vi "main.vi"() -> ()   [LabVIEW 2014]
uses:
  UerDefineControl/quit.ctl
  UerDefineControl/MMMdsc.ctl
  UerDefineControl/chax.ctl
  UerDefineControl/timee.ctl
  UerDefineControl/power.ctl
  <vilib>/Math Plots/3D Math Plots/3D Surface/3D Surface XCtrl/3D Surface.xctl
  CYY/strr.ctl
  UerDefineControl/qiehuan.ctl
  controls/State.ctl
  Acquisition/User Specified Data.ctl
  Acquisition/HW Configuration.ctl
  Acquisition/AcqControls/Analysis Configuration.ctl
  Acquisition/AcqControls/New Data Behavior.ctl
  support/Message Queue/Enqueue Message (Single).vi
  <vilib>/imath/engines/lvmath2/RunTimeEngine/Managers/WorkSpace/UID Generator.vi
  <vilib>/imath/engines/lvmath2/RunTimeEngine/BuiltInFunctions/max/1 input/NIMS_max(RV).vi
  <instcachedir>/0/NIMS_max(RV)_237633DB1D604D5BA7001287DF3C7957.lvgen/NIMS_max(RV)_237633DB1D604D5BA7001287DF3C7957_000.vi
  <vilib>/imath/engines/lvmath2/RunTimeEngine/BuiltInFunctions/min/1 input/NIMS_min(RV).vi
  <instcachedir>/0/NIMS_min(RV)_EE2DD3E2888846108C5160A664B67832.lvgen/NIMS_min(RV)_EE2DD3E2888846108C5160A664B67832_000.vi
  <vilib>/imath/engines/lvmath2/RunTimeEngine/BuiltInFunctions/linramp/NIMS_linramp.vi
  <vilib>/imath/engines/lvmath2/RunTimeEngine/BuiltInFunctions/meshgrid2d/NIMS_meshgrid2d(V,V).vi
  <instcachedir>/0/NIMS_meshgrid2d(V,V)_3733343E1C554A708015CFB0432C6A59.lvgen/NIMS_meshgrid2d(V,V)_3733343E1C554A708015CFB0432C6A59_000.vi
  <vilib>/imath/engines/lvmath2/RunTimeEngine/BuiltInFunctions/intrp2d_uneven/NIMS_[1o]_intrp2d_uneven.vi
  <vilib>/imath/engines/lvmath2/RunTimeEngine/RunTimeType/NIMS_RunTimeType_From StrictType (excl LVString).vi
  <instcachedir>/0/NIMS_RunTimeType_From StrictType (excl LVString)_15A5391EEA9C4AACB9955AC755B83D29.lvgen/NIMS_RunTimeType_From StrictType (excl LVString)_15A5391EEA9C4AACB9955AC755B83D29_000.vi
  <vilib>/imath/engines/lvmath2/RunTimeEngine/ErrorHandling/NIMS_Error From Error Code.vi
  <vilib>/imath/engines/lvmath2/RunTimeEngine/LocalVariableDefStatement/MC_LocalVariableDefStatement_Display.vi
  <vilib>/imath/engines/lvmath2/RunTimeEngine/Managers/SymbolTable/Clear UID.vi
  <vilib>/imath/engines/lvmath2/RunTimeEngine/NodeEndStatement/NIMS_NodeEndStatement_Output.vi
  <instcachedir>/0/NIMS_NodeEndStatement_Output_53EC0D466D134D7ABD903AC30B43404B.lvgen/NIMS_NodeEndStatement_Output_53EC0D466D134D7ABD903AC30B43404B_002.vi
  <vilib>/imath/engines/lvmath2/RunTimeEngine/ErrorHandling/NIMS_Finalize Error.vi
  <vilib>/Math Plots/3D Math Plots/3D Surface/3D Surface Datatype/Public/Plot Helper (Matrix).vi
  <vilib>/Math Plots/3D Math Plots/3D Mesh/3D Mesh Datatype/Public/Plot Helper (Matrix).vi
  <vilib>/Math Plots/3D Math Plots/3D Contour/3D Contour Datatype/Public/Plot Helper (Matrix).vi
  <vilib>/imath/engines/lvmath2/RunTimeEngine/BuiltInFunctions/plot/NIMS_plot(RM, RM, Str).vi
  <vilib>/imathl/engines/lvmath/Functions/Error Handling/Create Error.vi
  Acquisition/Acquisitions.lvlib
  AreaSettingD/SettingD.llb/SettingD.lvlib
  DetectElecrodes/DetectElectros.lvlib
  PowerElectrode/PowerElectrodes.lvlib
  DSCBoard/Dsc_Board_Dlg.lvlib
  DscBoardDistributeElectrodes/DscBoardDistributeElectrodes.lvlib
  Sample/Sample.lvlib
  DataBase/DataBase.lvlib
  <vilib>/Math Plots/3D Math Plots/3D Surface/3D Surface Datatype/3D Surface Datatype.lvclass
  <vilib>/imath/engines/lvmath2/RunTimeEngine/Managers/SymbolTable/NIMS_WorkSpace.lvlib
  <vilib>/Math Plots/3D Math Plots/3D Contour/3D Contour Datatype/3D Contour Datatype.lvclass
  <vilib>/imath/engines/lvmath2/RunTimeEngine/BuiltInFunctions/mesh/NIMS_mesh(RM, RM).vi
  <vilib>/imath/engines/lvmath2/RunTimeEngine/BuiltInFunctions/grid/NIMS_grid(Enums).vi
  ChaxuConfig/ChaxuConfig.lvlib
  HardWare/HardWareConfig.lvlib
  <vilib>/Math Plots/3D Math Plots/3D Mesh/3D Mesh Datatype/3D Mesh Datatype.lvclass
  PowerControl/PowerControl.lvlib
  support/Message Queue/Message Queue.lvlib
  CYY/cyy.lvlib
  LeakageFenxi/LeakageFenXi.lvlib
panel:
  in  "界面切换":T1
  in  "电源控制":T2
  in  "定时检测":T3
  in  "SampleInfo":bool
  in  "电极配置信息查询":T4
  in  "Mdsc":T5
  in  "手动检测":T6
  in  "退出":T7
  out "采样过程中 ... 请不要进行其它操作":u32(slide) scale=0.0..400.0
  in  "采集板分配电极":bool
  in  "供电电极配置":bool
  in  "检测电极配置":bool
  in  "区域配置":bool
  in  "选项卡控件":enum32{"主界面", "数据监测界面", "测试数据", "测试数据 2"}(tab)
  out "Info 2":string
  out "3D Surface 3":refnum<class "3D Plot Datatype.lvclass">[](xcontrol) caption="三维曲面"
  out "Info":T8
  out "3D Surface":refnum<class "3D Plot Datatype.lvclass">[](xcontrol) caption="三维曲面"
  in  "数据监测界面":i32(listbox)
  out "定时采样信息D":string[][](array[string])
  out "定时检测事件":bool
  out "是否采样":bool
  in  "频率":dbl=1.0
  out "电流":string
  out "字符串":string="下层膜"
  out "选定检测区域":string
  out "数据采集模块地址":string
  out "elecNum":i32
  out "detec_electrode_name":string
  out "电压回来":string
  out "项标识符":string
  out "电压频率":string
  out "电压倍数":string
  out "Hz":i32
  out "实际输出电压":string
  out "电压系数":string
  out "输出电压值":string
  out "电压05V":string
  out "实际输出电压压":dbl
  out "电压系数输出":dbl
  out "回来电压":dbl
  out "NY":bool
  in  "设置按钮":bool
  # "Welcome to use Leakage Detection System !"
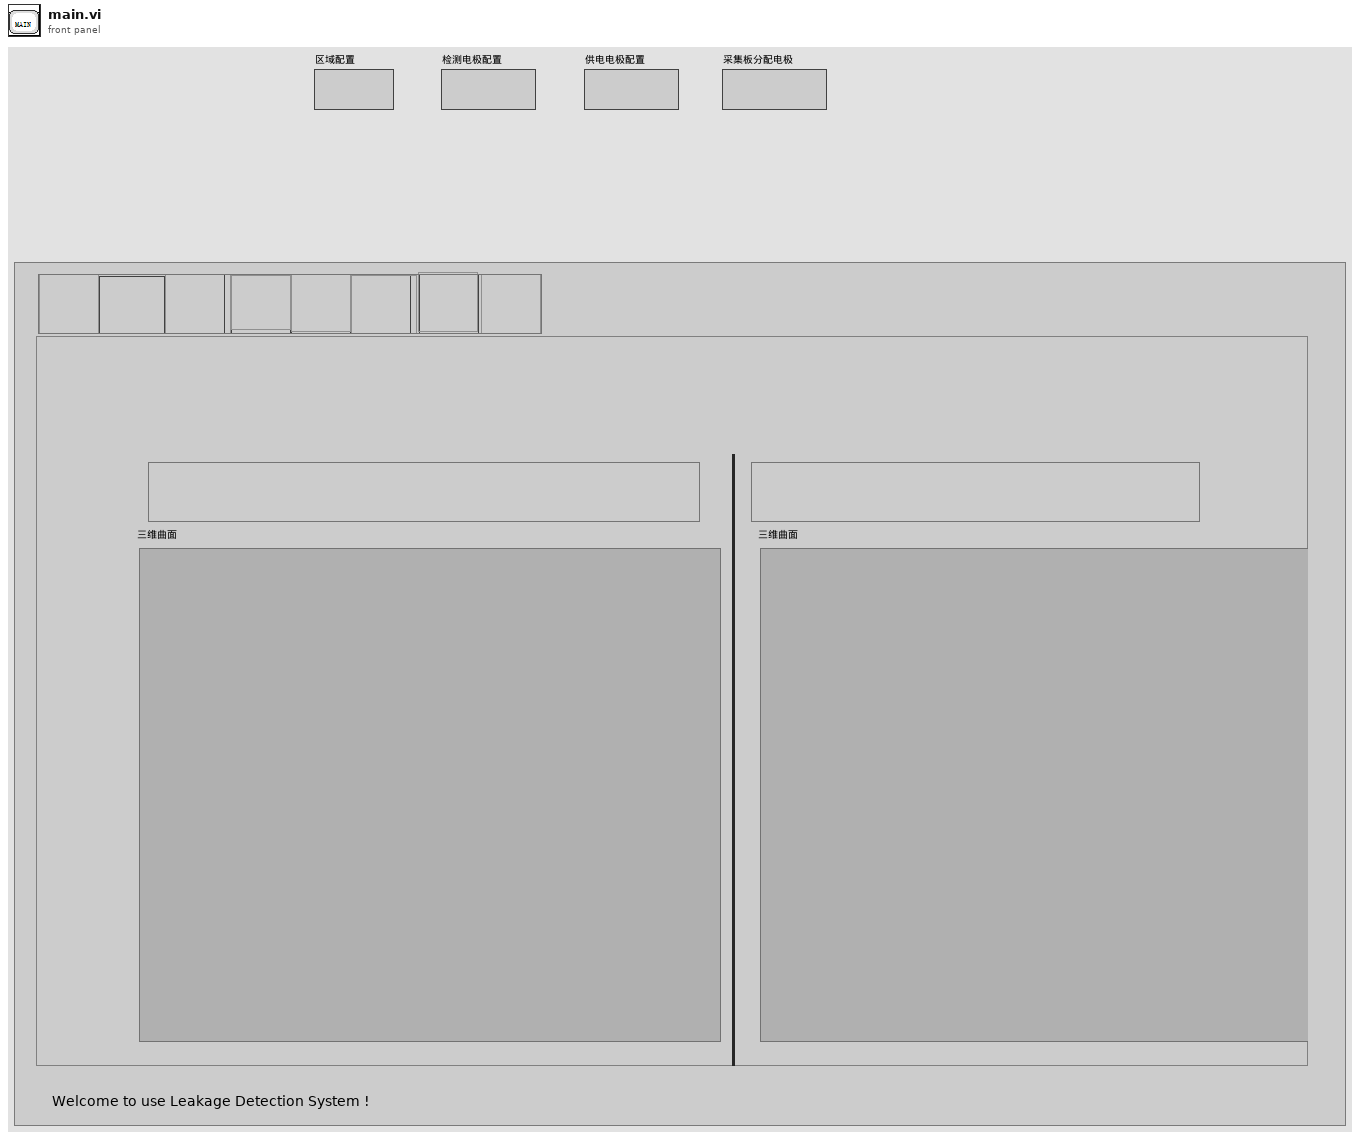
[diagram p1: front panel]
types:
  T1 = typedef "qiehuan.ctl" = bool
  T2 = typedef "power.ctl" = bool
  T3 = typedef "timee.ctl" = bool
  T4 = typedef "chax.ctl" = bool
  T5 = typedef "MMMdsc.ctl" = bool
  T6 = typedef "手动.ctl" = bool
  T7 = typedef "quit.ctl" = bool
  T8 = typedef "strr.ctl" = string
  T9 = cluster{"区域名称":string, "采样位置":string, "采样时间":string, "时":string, "分":string}
  T10 = typedef "State.ctl" = enum16{"Idle", "AOoutputting", "Timing", "SamplingAndSaving", "StartSample", "StopSample"}
  T11 = typedef "Message Queue.lvlib/All Message Queues.ctl" = cluster{"UI":refnum<queue>, "Acquisition":refnum<queue>, "Logging":refnum<queue>}
  T12 = cluster{"Max Input":dbl, "Min Input":dbl, "Sample Rate":dbl, "Sample Num":dbl, "DAQmx Task":refnum<k21>, "物理通道":tag}
  T13 = typedef "HardWareConfig.lvlib/Hardware Configures.ctl" = cluster{"Max Input":dbl, "Min Input":dbl, "Sample Rate":dbl, "Sample Num":dbl, "DAQmx Task":refnum<k21>, "物理通道":tag}
  T14 = enum32{"invalid app kind", "Development System", "Run Time System", "Student Edition", "Embedded LabVIEW", "Evaluation", "Custom"}
  T15 = enum32{"Invalid", "Standard", "Closed", "Hidden", "Minimized", "Maximized"}
  T16 = typedef "Acquisitions.lvlib/HW Configuration.ctl" = cluster{"Physical Channel":tag, "Maximum Input":dbl, "Minimum Input":dbl, "Sample Rate":dbl, "Number of Samples":i32}
  T17 = cluster{"Dev1ASData":cluster{"DevChSampData":cluster{"通道编号":string, "Data":dbl}[], "dscAddress":string}, "Dev2ASData":cluster{"DevChSampData":cluster{"通道编号":string, "Data":dbl}[], "dscAddress":string}, "Dev3ASData":cluster{"DevChSampData":cluster{"通道编号":string, "Data":dbl}[], "dscAddress":string}, "Dev4ASData":cluster{"DevChSampData":cluster{"通道编号":string, "Data":dbl}[], "dscAddress":string}, "Dev5ASData":cluster{"DevChSampData":cluster{"通道编号":string, "Data":dbl}[], "dscAddress":string}, "Dev6ASData":cluster{"DevChSampData":cluster{"通道编号":string, "Data":dbl}[], "dscAddress":string}, "Dev7ASData":cluster{"DevChSampData":cluster{"通道编号":string, "Data":dbl}[], "dscAddress":string}, "Dev8ASData":cluster{"DevChSampData":cluster{"通道编号":string, "Data":dbl}[], "dscAddress":string}, "Dev9ASData":cluster{"DevChSampData":cluster{"通道编号":string, "Data":dbl}[], "dscAddress":string}, "Dev10ASData":cluster{"DevChSampData":cluster{"通道编号":string, "Data":dbl}[], "dscAddress":string}, "Dev11ASData":cluster{"DevChSampData":cluster{"通道编号":string, "Data":dbl}[], "dscAddress":string}, "Dev12ASData":cluster{"DevChSampData":cluster{"通道编号":string, "Data":dbl}[], "dscAddress":string}, "Dev13ASData":cluster{"DevChSampData":cluster{"通道编号":string, "Data":dbl}[], "dscAddress":string}}
  T18 = typedef "Acquisitions.lvlib/User Specified Data.ctl" = cluster{"Hardware Configuration":T16, "Analysis Configuration":T19, "New Data Behavior":T20, "HWInfo":string}
  T19 = typedef "Acquisitions.lvlib/Analysis Configuration.ctl" = cluster{"Statistics":bool}
  T20 = typedef "Acquisitions.lvlib/New Data Behavior.ctl" = enum16{"Replace", "Overlay", "Append"}
  T21 = cluster{"Core":cluster{"Current VI Reference":refnum<vi>, "Close Panel on Exit?":bool}, "Your Boolean data":bool, "Your string data":string, "User Specified":T18, "手动采样信息":cluster{"选定检测区域":string, "采样位置":string, "电源电压":string, "电源电流":string, "电源频率":string, "检测方式":string, "备注":string}, "ManualSampleInfo":cluster{string, "date/time string":string, "选定检测区域":string, "采样位置":string, "检测方式":string, string, string, "电源电压":string, "电源电流":string, "备注":string}, "SampleData":dbl[], "AcquireData":waveform(dbl)[], "DevChSampleData":cluster{"数据采集模块地址":string, "0ChData":cluster{"通道编号":string, "Data":dbl}, "1ChData":cluster{"通道编号":string, "Data":dbl}, "2ChData":cluster{"通道编号":string, "Data":dbl}, "3ChData":cluster{"通道编号":string, "Data":dbl}, "4ChData":cluster{"通道编号":string, "Data":dbl}, "5ChData":cluster{"通道编号":string, "Data":dbl}, "6ChData":cluster{"通道编号":string, "Data":dbl}, "7ChData":cluster{"通道编号":string, "Data":dbl}, "8ChData":cluster{"通道编号":string, "Data":dbl}, "9ChData":cluster{"通道编号":string, "Data":dbl}, "10ChData":cluster{"通道编号":string, "Data":dbl}, "11ChData":cluster{"通道编号":string, "Data":dbl}, "12ChData":cluster{"通道编号":string, "Data":dbl}, "13ChData":cluster{"通道编号":string, "Data":dbl}, "14ChData":cluster{"通道编号":string, "Data":dbl}, "15ChData":cluster{"通道编号":string, "Data":dbl}, "16ChData":cluster{"通道编号":string, "Data":dbl}, "17ChData":cluster{"通道编号":string, "Data":dbl}, "18ChData":cluster{"通道编号":string, "Data":dbl}, "19ChData":cluster{"通道编号":string, "Data":dbl}, "20ChData":cluster{"通道编号":string, "Data":dbl}, "21ChData":cluster{"通道编号":string, "Data":dbl}, "22ChData":cluster{"通道编号":string, "Data":dbl}, "23ChData":cluster{"通道编号":string, "Data":dbl}, "24ChData":cluster{"通道编号":string, "Data":dbl}, "25ChData":cluster{"通道编号":string, "Data":dbl}, "26ChData":cluster{"通道编号":string, "Data":dbl}, "27ChData":cluster{"通道编号":string, "Data":dbl}, "28ChData":cluster{"通道编号":string, "Data":dbl}, "29ChData":cluster{"通道编号":string, "Data":dbl}, "30ChData":cluster{"通道编号":string, "Data":dbl}, "31ChData":cluster{"通道编号":string, "Data":dbl}}, "DevChSampData":cluster{"通道编号":string, "Data":dbl}[], "SampleInfoTime":string, "SampleData":string[][], "3DData":cluster{"X":dbl[], "Y":dbl[], "Z":dbl[]}, "定时采样信息":cluster{"检测区域":string, "检测频率":string, "时":u16, "分钟":u16, "供电位置":string, "是否启动":string, "备注":string}, "TimeSampleInfo":cluster{string, "采样时间":string, "检测区域":string, "供电位置":string, "采样方式":string, string, string, "电源电压":string, "电源电流":string, "备注":string}, "nCHData":cluster{"Dev1SampData":cluster{"通道编号":string, "Data":dbl}[], "Dev2SampData":cluster{"通道编号":string, "Data":dbl}[], "Dev3SampData":cluster{"通道编号":string, "Data":dbl}[], "Dev4SampData":cluster{"通道编号":string, "Data":dbl}[], "Dev5SampData":cluster{"通道编号":string, "Data":dbl}[], "Dev6SampData":cluster{"通道编号":string, "Data":dbl}[], "Dev7SampData":cluster{"通道编号":string, "Data":dbl}[], "Dev8SampData":cluster{"通道编号":string, "Data":dbl}[], "Dev9SampData":cluster{"通道编号":string, "Data":dbl}[], "Dev10SampData":cluster{"通道编号":string, "Data":dbl}[], "Dev11SampData":cluster{"通道编号":string, "Data":dbl}[], "Dev12SampData":cluster{"通道编号":string, "Data":dbl}[], "Dev13SampData":cluster{"通道编号":string, "Data":dbl}[]}, "DevNASSData":cluster{"Dev1ASData":cluster{"DevChSampData":cluster{"通道编号":string, "Data":dbl}[], "dscAddress":string}, "Dev2ASData":cluster{"DevChSampData":cluster{"通道编号":string, "Data":dbl}[], "dscAddress":string}, "Dev3ASData":cluster{"DevChSampData":cluster{"通道编号":string, "Data":dbl}[], "dscAddress":string}, "Dev4ASData":cluster{"DevChSampData":cluster{"通道编号":string, "Data":dbl}[], "dscAddress":string}, "Dev5ASData":cluster{"DevChSampData":cluster{"通道编号":string, "Data":dbl}[], "dscAddress":string}, "Dev6ASData":cluster{"DevChSampData":cluster{"通道编号":string, "Data":dbl}[], "dscAddress":string}, "Dev7ASData":cluster{"DevChSampData":cluster{"通道编号":string, "Data":dbl}[], "dscAddress":string}, "Dev8ASData":cluster{"DevChSampData":cluster{"通道编号":string, "Data":dbl}[], "dscAddress":string}, "Dev9ASData":cluster{"DevChSampData":cluster{"通道编号":string, "Data":dbl}[], "dscAddress":string}, "Dev10ASData":cluster{"DevChSampData":cluster{"通道编号":string, "Data":dbl}[], "dscAddress":string}, "Dev11ASData":cluster{"DevChSampData":cluster{"通道编号":string, "Data":dbl}[], "dscAddress":string}, "Dev12ASData":cluster{"DevChSampData":cluster{"通道编号":string, "Data":dbl}[], "dscAddress":string}, "Dev13ASData":cluster{"DevChSampData":cluster{"通道编号":string, "Data":dbl}[], "dscAddress":string}}, "PowTN":bool, "记录数":i32, "是否存在记录":bool, "power_f":string, "时分":string, "电压倍数":string, "回来电压":string, "回来电流":string, "Area_name":string, "电压系数":string, "基准电压":string, "手动采样到AO电压":string}
  T22 = typedef "LVPoint32TypeDef.ctl" = cluster{"Horizontal":i32, "Vertical":i32}
  T23 = typedef "LVRowAndColumnTypeDef.ctl" = cluster{"Row":i32, "Column":i32}
  T24 = cluster{string, "采样时间":string, "检测区域":string, "供电位置":string, "采样方式":string, string, string, "电源电压":string, "电源电流":string, "备注":string}
  T25 = cluster{"Dev1SampData":cluster{"通道编号":string, "Data":dbl}[], "Dev2SampData":cluster{"通道编号":string, "Data":dbl}[], "Dev3SampData":cluster{"通道编号":string, "Data":dbl}[], "Dev4SampData":cluster{"通道编号":string, "Data":dbl}[], "Dev5SampData":cluster{"通道编号":string, "Data":dbl}[], "Dev6SampData":cluster{"通道编号":string, "Data":dbl}[], "Dev7SampData":cluster{"通道编号":string, "Data":dbl}[], "Dev8SampData":cluster{"通道编号":string, "Data":dbl}[], "Dev9SampData":cluster{"通道编号":string, "Data":dbl}[], "Dev10SampData":cluster{"通道编号":string, "Data":dbl}[], "Dev11SampData":cluster{"通道编号":string, "Data":dbl}[], "Dev12SampData":cluster{"通道编号":string, "Data":dbl}[], "Dev13SampData":cluster{"通道编号":string, "Data":dbl}[]}
  T26 = cluster{"采样时间":string, string, "检测区域":string, "供电位置":string, "采样方式":string, "电源电压":string, string, "电源电流":string, string, "备注":string}
  T27 = cluster{"检测区域":string, "检测频率":string, "时":u16, "分钟":u16, "供电位置":string, "是否启动":string, "备注":string}
  T28 = cluster{"数据采集模块地址":string, "0ChData":cluster{"通道编号":string, "Data":dbl}, "1ChData":cluster{"通道编号":string, "Data":dbl}, "2ChData":cluster{"通道编号":string, "Data":dbl}, "3ChData":cluster{"通道编号":string, "Data":dbl}, "4ChData":cluster{"通道编号":string, "Data":dbl}, "5ChData":cluster{"通道编号":string, "Data":dbl}, "6ChData":cluster{"通道编号":string, "Data":dbl}, "7ChData":cluster{"通道编号":string, "Data":dbl}, "8ChData":cluster{"通道编号":string, "Data":dbl}, "9ChData":cluster{"通道编号":string, "Data":dbl}, "10ChData":cluster{"通道编号":string, "Data":dbl}, "11ChData":cluster{"通道编号":string, "Data":dbl}, "12ChData":cluster{"通道编号":string, "Data":dbl}, "13ChData":cluster{"通道编号":string, "Data":dbl}, "14ChData":cluster{"通道编号":string, "Data":dbl}, "15ChData":cluster{"通道编号":string, "Data":dbl}, "16ChData":cluster{"通道编号":string, "Data":dbl}, "17ChData":cluster{"通道编号":string, "Data":dbl}, "18ChData":cluster{"通道编号":string, "Data":dbl}, "19ChData":cluster{"通道编号":string, "Data":dbl}, "20ChData":cluster{"通道编号":string, "Data":dbl}, "21ChData":cluster{"通道编号":string, "Data":dbl}, "22ChData":cluster{"通道编号":string, "Data":dbl}, "23ChData":cluster{"通道编号":string, "Data":dbl}, "24ChData":cluster{"通道编号":string, "Data":dbl}, "25ChData":cluster{"通道编号":string, "Data":dbl}, "26ChData":cluster{"通道编号":string, "Data":dbl}, "27ChData":cluster{"通道编号":string, "Data":dbl}, "28ChData":cluster{"通道编号":string, "Data":dbl}, "29ChData":cluster{"通道编号":string, "Data":dbl}, "30ChData":cluster{"通道编号":string, "Data":dbl}, "31ChData":cluster{"通道编号":string, "Data":dbl}}
  T29 = cluster{string, "date/time string":string, "选定检测区域":string, "采样位置":string, "检测方式":string, string, string, "电源电压":string, "电源电流":string, "备注":string}
  T30 = cluster{"选定检测区域":string, "采样位置":string, "电源电压":string, "电源电流":string, "电源频率":string, "检测方式":string, "备注":string}
  T31 = cluster{"Current VI Reference":refnum<vi>, "Close Panel on Exit?":bool}
  T32 = cluster{"DevChSampData":cluster{"通道编号":string, "Data":dbl}[], "dscAddress":string}
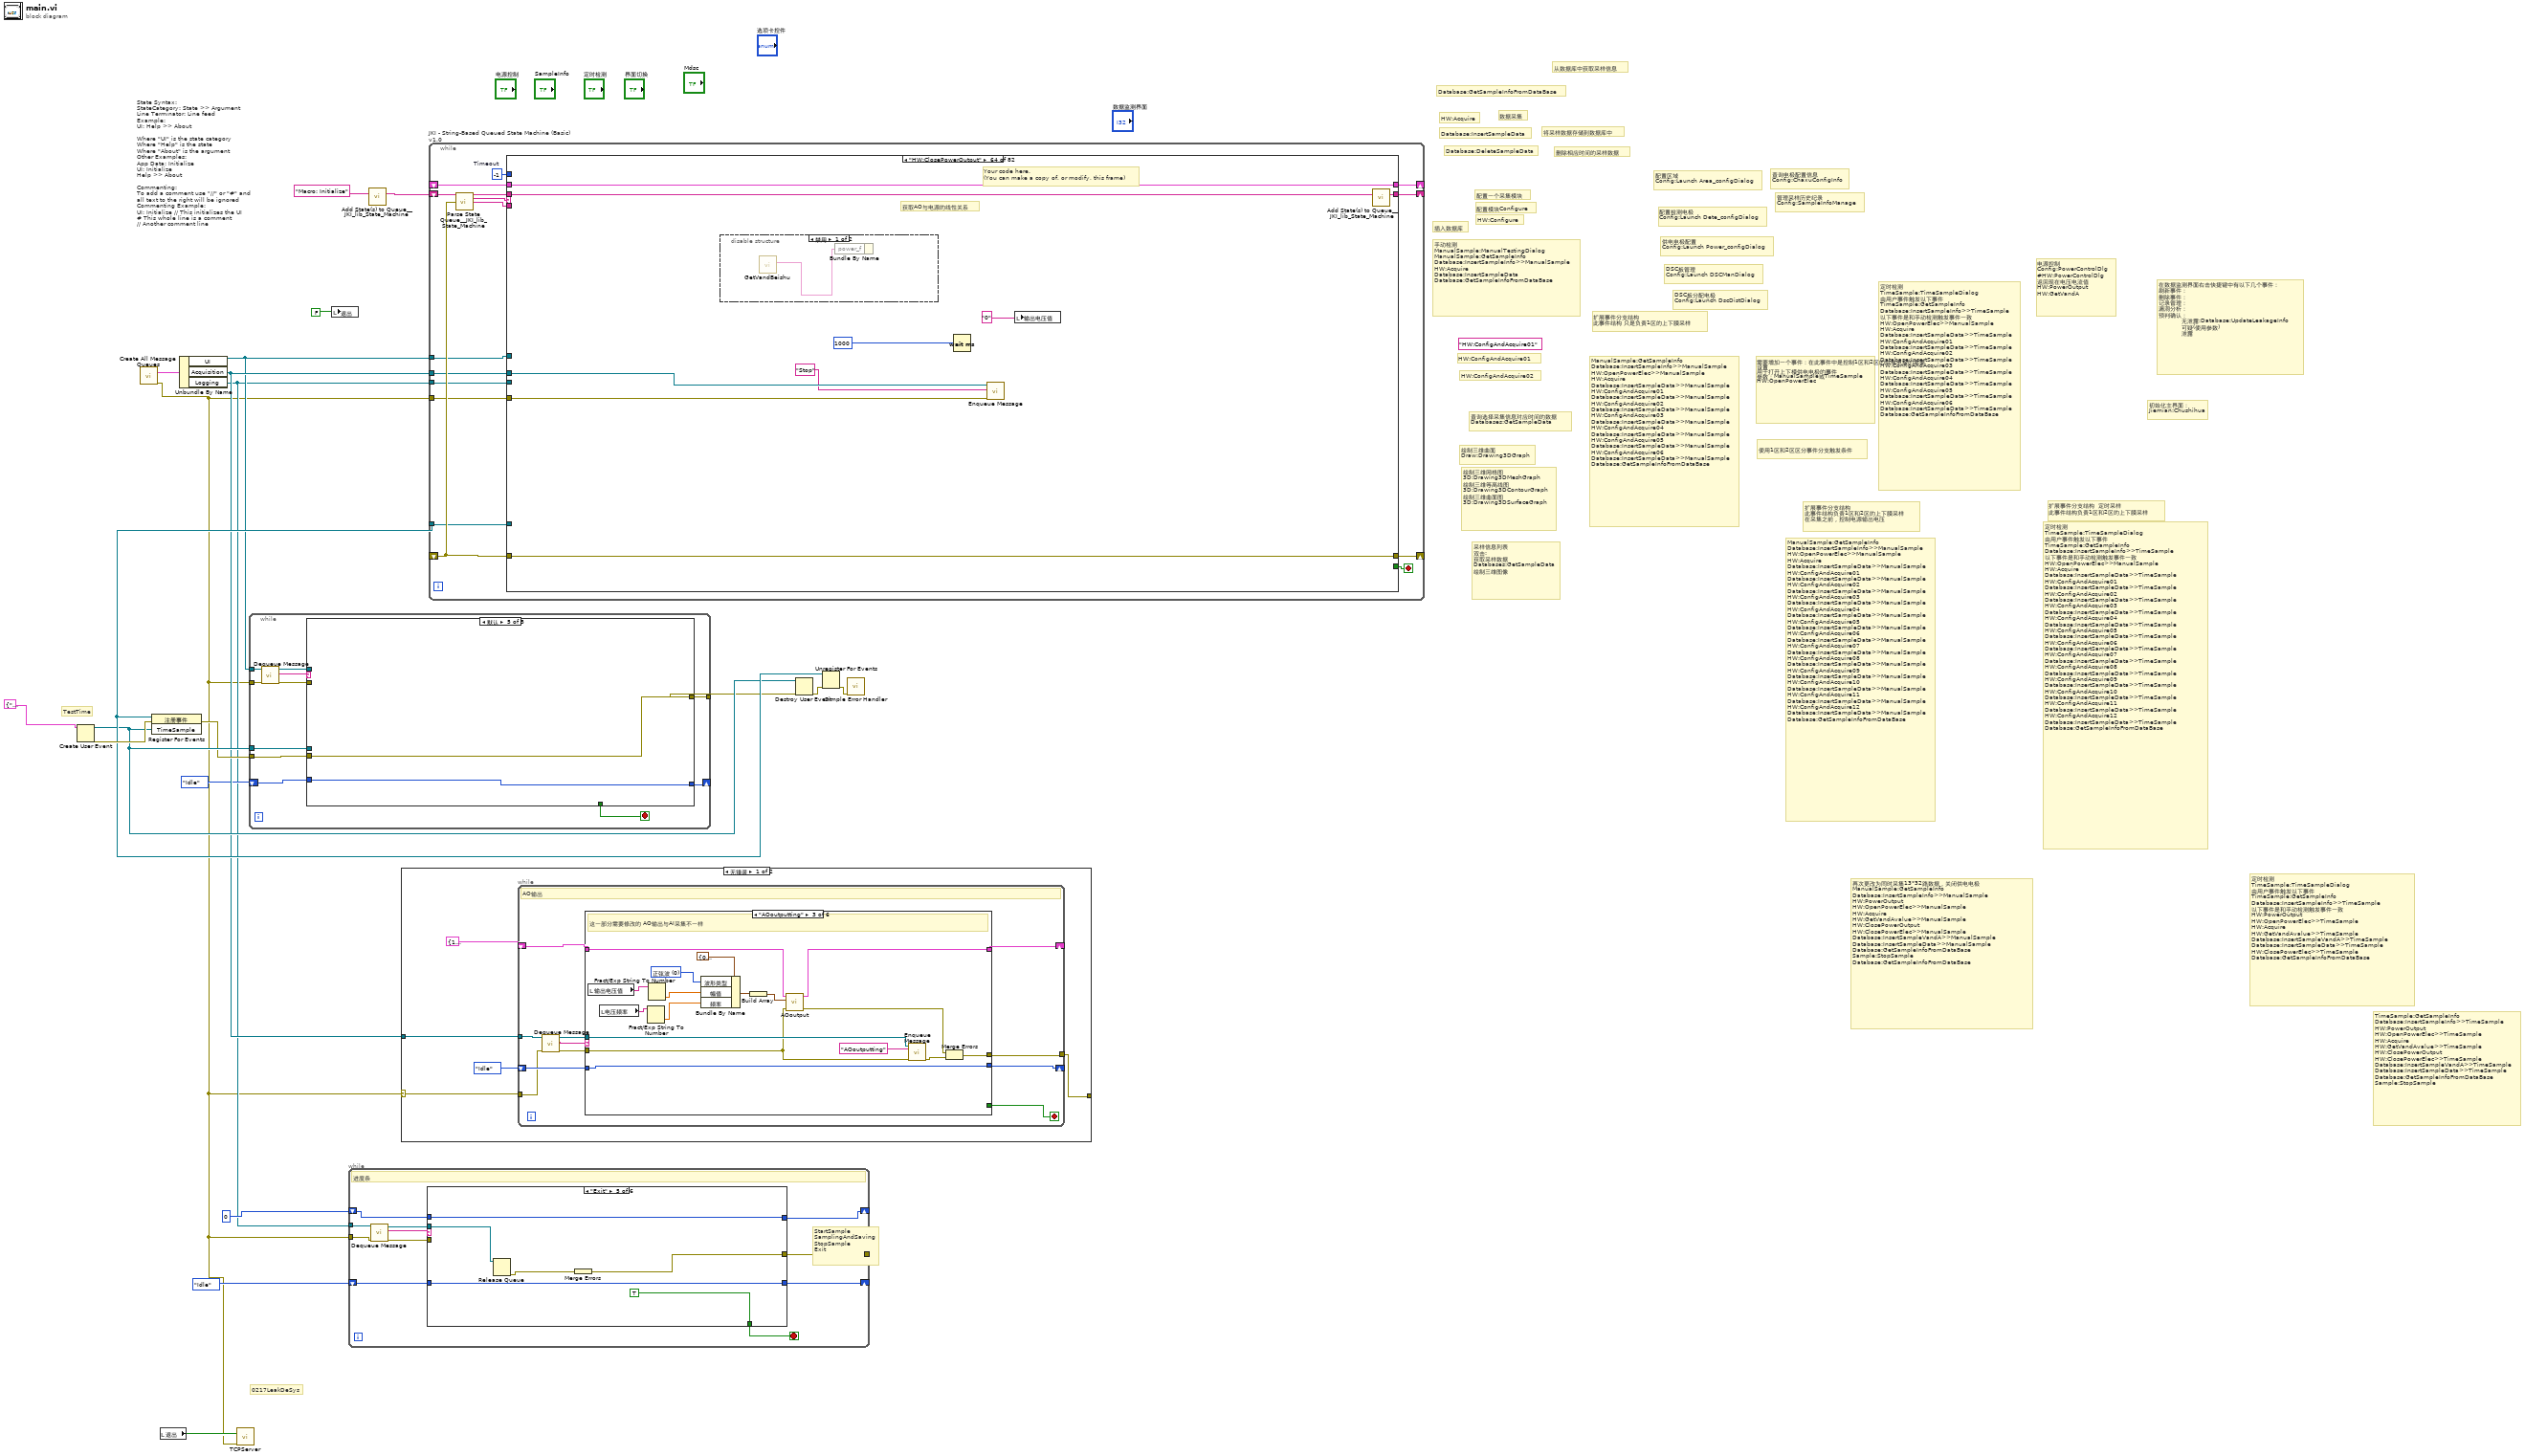
[diagram p0: block diagram]
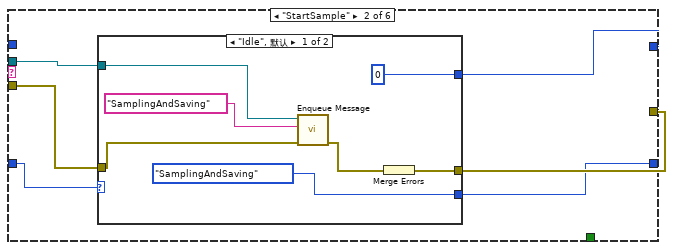
[diagram p3: hidden frame]
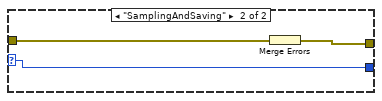
[diagram p4: hidden frame]
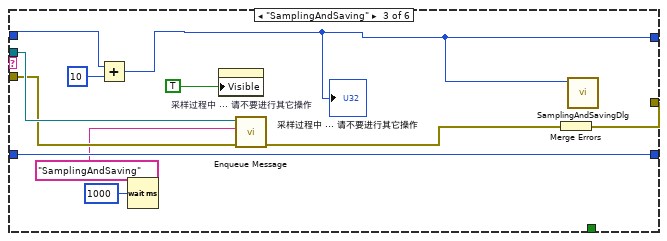
[diagram p5: hidden frame]
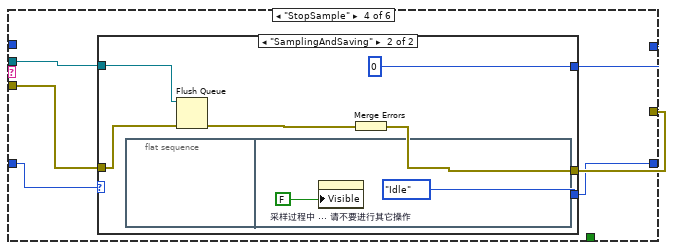
[diagram p6: hidden frame]
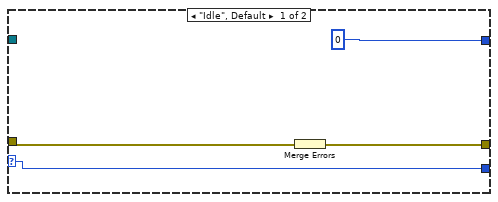
[diagram p7: hidden frame]
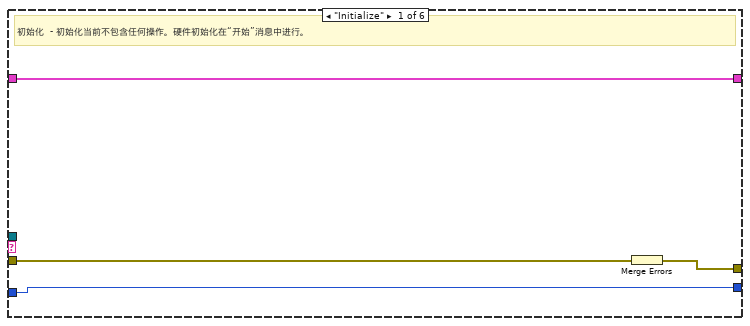
[diagram p9: hidden frame]
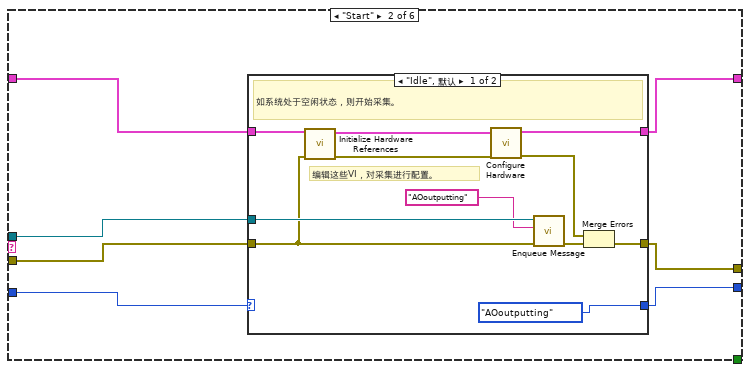
[diagram p10: hidden frame]
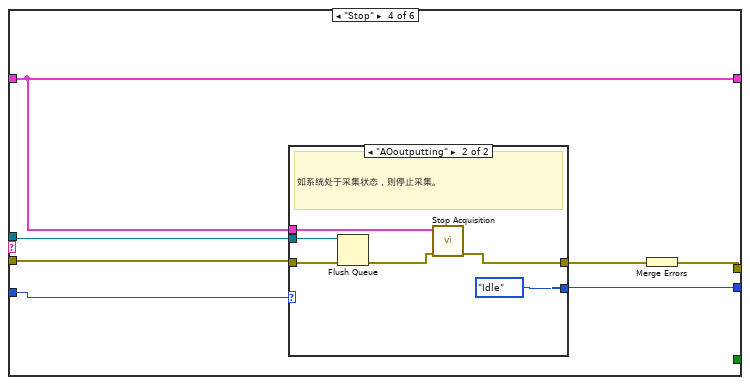
[diagram p12: hidden frame]
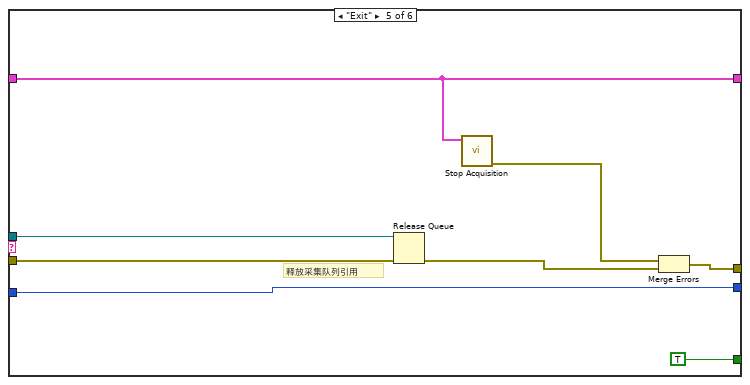
[diagram p14: hidden frame]
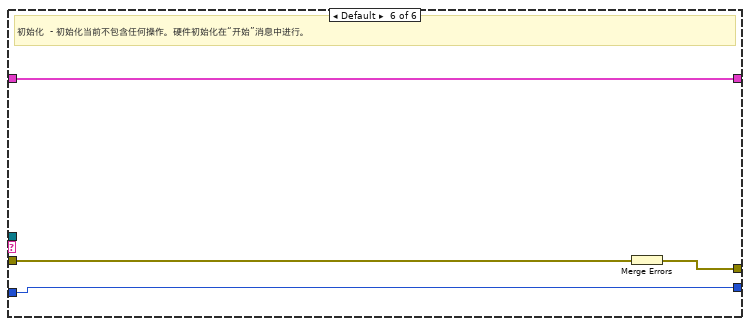
[diagram p15: hidden frame]
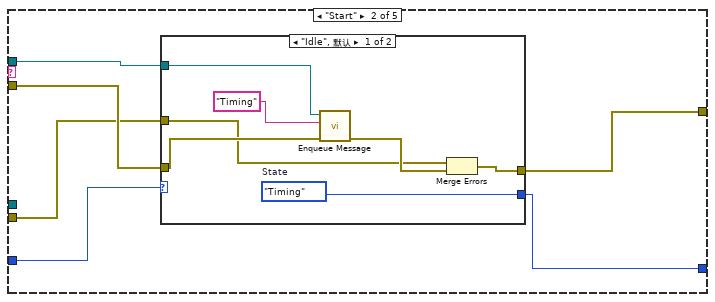
[diagram p18: hidden frame]
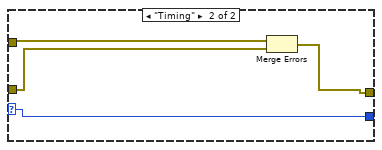
[diagram p19: hidden frame]
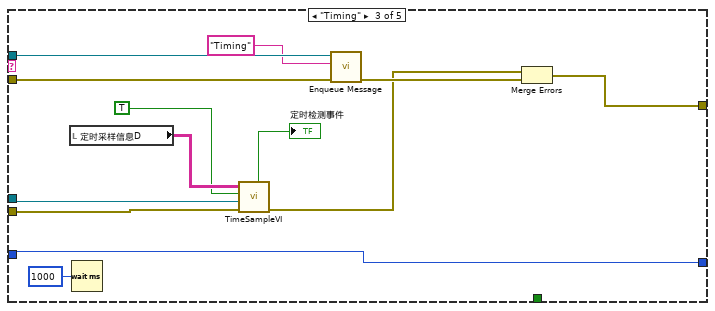
[diagram p20: hidden frame]
diagram:
  (unwired) "HW:ConfigAndAcquire01"
  # "0217LeakDeSys"
  # "TimeSample:GetSampleInfo\nDatabase:InsertSampleInfo>>TimeSample\nHW:PowerOutput\nHW:OpenPowerElec>>TimeSample\nHW:Acquire\nHW:GetVandAvalue>>TimeSample\nHW:ClosePowerOutput\nHW:ClosePowerElec>>TimeSample\nDatabase:InsertSampleVandA>>TimeSample\nDatabase:InsertSampleData>>TimeSample\nDatabase:GetSampleInfoFromDataBase\nSample:StopSample"
  # "StartSample\nSamplingAndSaving\nStopSample\nExit"
  # "采样信息列表\n双击:\n获取采样数据\nDatabases:GetSampleData\n绘制三维图像"
  # "绘制三维网格图\n3D:Drawing3DMeshGraph\n绘制三维等高线图\n3D:Drawing3DContourGraph\n绘制三维曲面图\n3D:Drawing3DSurfaceGraph"
  # "定时检测\nTimeSample:TimeSampleDialog\n由用户事件触发以下事件\nTimeSample:GetSampleInfo\nDatabase:InsertSampleInfo>>TimeSample\n以下事件是和手动检测触发事件一致\nHW:PowerOutput\nHW:OpenPowerElec>>TimeSample\nHW:Acquire\nHW:GetVandAvalue>>TimeSample\nDatabase:InsertSampleVandA>>TimeSample\nDatabase:InsertSampleData>>TimeSample\nHW:ClosePowerElec>>TimeSample\nDatabase:GetSampleInfoFromDataBase"
  # "初始化主界面：\nJiemian:Chushihua"
  # "在数据监测界面右击快捷键中有以下几个事件：\n刷新事件：\n删除事件：\n记录管理：\n漏洞分析：\n预判确认：\n            无泄露:Database:UpdateLeakageInfo\n            可疑(使用参数)\n            泄露"
  # "删除相应时间的采样数据"
  # "Database:DeleteSampleData"
  # "再次更改为同时采集13*32路数据，关闭供电电极\nManualSample:GetSampleInfo\nDatabase:InsertSampleInfo>>ManualSample\nHW:PowerOutput\nHW:OpenPowerElec>>ManualSample\nHW:Acquire\nHW:GetVandAvalue>>ManualSample\nHW:ClosePowerOutput\nHW:ClosePowerElec>>ManualSample\nDatabase:InsertSampleVandA>>ManualSample\nDatabase:InsertSampleData>>ManualSample\nDatabase:GetSampleInfoFromDataBase\nSample:StopSample\nDatabase:GetSampleInfoFromDataBase"
  # "电源控制\nConfig:PowerControlDlg\n#HW:PowerControlDlg\n返回现在电压电流值\nHW:PowerOutput\nHW:GetVandA"
  # "扩展事件分支结构  定时采样\n此事件结构负责1区和2区的上下膜采样"
  # "定时检测\nTimeSample:TimeSampleDialog\n由用户事件触发以下事件\nTimeSample:GetSampleInfo\nDatabase:InsertSampleInfo>>TimeSample\n以下事件是和手动检测触发事件一致\nHW:OpenPowerElec>>ManualSample\nHW:Acquire\nDatabase:InsertSampleData>>TimeSample\nHW:ConfigAndAcquire01\nDatabase:InsertSampleData>>TimeSample\nHW:ConfigAndAcquire02\nDatabase:InsertSampleData>>TimeSample\nHW:ConfigAndAcquire03\nDatabase:InsertSampleData>>TimeSample\nHW:ConfigAndAcquire04\nDatabase:InsertSampleData>>TimeSample\nHW:ConfigAndAcquire05\nDatabase:InsertSampleData>>TimeSample\nHW:ConfigAndAcquire06\nDatabase:InsertSampleData>>TimeSample\nHW:ConfigAndAcquire07\nDatabase:InsertSampleData>>TimeSample\nHW:ConfigAndAcquire08\nDatabase:InsertSampleData>>TimeSample\nHW:ConfigAndAcquire09\nDatabase:InsertSampleData>>TimeSample\nHW:ConfigAndAcquire10\nDatabase:InsertSampleData>>TimeSample\nHW:ConfigAndAcquire11\nDatabase:InsertSampleData>>TimeSample\nHW:ConfigAndAcquire12\nDatabase:InsertSampleData>>TimeSample\nDatabase:GetSampleInfoFromDataBase"
  # "扩展事件分支结构\n此事件结构负责1区和2区的上下膜采样\n在采集之前，控制电源输出电压"
  # "ManualSample:GetSampleInfo\nDatabase:InsertSampleInfo>>ManualSample\nHW:OpenPowerElec>>ManualSample\nHW:Acquire\nDatabase:InsertSampleData>>ManualSample\nHW:ConfigAndAcquire01\nDatabase:InsertSampleData>>ManualSample\nHW:ConfigAndAcquire02\nDatabase:InsertSampleData>>ManualSample\nHW:ConfigAndAcquire03\nDatabase:InsertSampleData>>ManualSample\nHW:ConfigAndAcquire04\nDatabase:InsertSampleData>>ManualSample\nHW:ConfigAndAcquire05\nDatabase:InsertSampleData>>ManualSample\nHW:ConfigAndAcquire06\nDatabase:InsertSampleData>>ManualSample\nHW:ConfigAndAcquire07\nDatabase:InsertSampleData>>ManualSample\nHW:ConfigAndAcquire08\nDatabase:InsertSampleData>>ManualSample\nHW:ConfigAndAcquire09\nDatabase:InsertSampleData>>ManualSample\nHW:ConfigAndAcquire10\nDatabase:InsertSampleData>>ManualSample\nHW:ConfigAndAcquire11\nDatabase:InsertSampleData>>ManualSample\nHW:ConfigAndAcquire12\nDatabase:InsertSampleData>>ManualSample\nDatabase:GetSampleInfoFromDataBase"
  # "使用1区和2区区分事件分支触发条件"
  # "需要增加一个事件：在此事件中是控制1区和2区的供电电极的需要设置\n用于打开上下模供电电极的事件\n参数：ManualSample或TimeSample\nHW:OpenPowerElec"
  # "TestTime"
  # "定时检测\nTimeSample:TimeSampleDialog\n由用户事件触发以下事件\nTimeSample:GetSampleInfo\nDatabase:InsertSampleInfo>>TimeSample\n以下事件是和手动检测触发事件一致\nHW:OpenPowerElec>>ManualSample\nHW:Acquire\nDatabase:InsertSampleData>>TimeSample\nHW:ConfigAndAcquire01\nDatabase:InsertSampleData>>TimeSample\nHW:ConfigAndAcquire02\nDatabase:InsertSampleData>>TimeSample\nHW:ConfigAndAcquire03\nDatabase:InsertSampleData>>TimeSample\nHW:ConfigAndAcquire04\nDatabase:InsertSampleData>>TimeSample\nHW:ConfigAndAcquire05\nDatabase:InsertSampleData>>TimeSample\nHW:ConfigAndAcquire06\nDatabase:InsertSampleData>>TimeSample\nDatabase:GetSampleInfoFromDataBase"
  # "管理采样历史纪录\nConfig:SampleInfoManage"
  # "查询电极配置信息\nConfig:ChaxuConfigInfo"
  # "绘制三维曲面\nDraw:Drawing3DGraph"
  # "查询选择采集信息对应时间的数据\nDatabases:GetSampleData"
  # "HW:ConfigAndAcquire02"
  # "扩展事件分支结构\n此事件结构 只是负责1区的上下膜采样"
  # "ManualSample:GetSampleInfo\nDatabase:InsertSampleInfo>>ManualSample\nHW:OpenPowerElec>>ManualSample\nHW:Acquire\nDatabase:InsertSampleData>>ManualSample\nHW:ConfigAndAcquire01\nDatabase:InsertSampleData>>ManualSample\nHW:ConfigAndAcquire02\nDatabase:InsertSampleData>>ManualSample\nHW:ConfigAndAcquire03\nDatabase:InsertSampleData>>ManualSample\nHW:ConfigAndAcquire04\nDatabase:InsertSampleData>>ManualSample\nHW:ConfigAndAcquire05\nDatabase:InsertSampleData>>ManualSample\nHW:ConfigAndAcquire06\nDatabase:InsertSampleData>>ManualSample\nDatabase:GetSampleInfoFromDataBase"
  # "HW:ConfigAndAcquire01"
  # "将采样数据存储到数据库中"
  # "数据采集"
  # "从数据库中获取采样信息"
  # "Database:InsertSampleData"
  # "Database:GetSampleInfoFromDataBase"
  # "插入数据库"
  # "手动检测\nManualSample:ManualTestingDialog\nManualSample:GetSampleInfo\nDatabase:InsertSampleInfo>>ManualSample\nHW:Acquire\nDatabase:InsertSampleData\nDatabase:GetSampleInfoFromDataBase"
  # "DSC板分配电极\nConfig:Launch DscDistDialog"
  # "DSC板管理\nConfig:Launch DSCManDialog"
  # "供电电极配置\nConfig:Launch Power_configDialog"
  # "配置检测电极\nConfig:Launch Dete_configDialog"
  # "配置区域\nConfig:Launch Area_configDialog"
  # "HW:Acquire"
  # "HW:Configure"
  # "配置模块Configure"
  # "配置一个采集模块"
  # "State Syntax:\nStateCategory: State >> Argument\nLine Terminator: Line feed\nExample:\nUI: Help >> About\n\nWhere \"UI\" is the state category\nWhere \"Help\" is the state\nWhere \"About\" is the argument\nOther Examples:\nApp Data: Initialize\nUI: Initialize\nHelp >> About\n\nCommenting:\nTo add a comment use \"//\" or \"#\" and all text to the right will be ignored\nCommenting Example:\nUI: Initialize // This initializes the UI\n# This whole line is a comment\n// Another comment line"
  n1 = Create User Event(user event datatype=T9 {"区域名称"="", "采样位置"="", "采样时间"="", "时"="", "分"=""} ("TimeSample")) -> (user event=w14:refnum<user-event>, error out=w18:errorcluster)  [unwired: 1 in]
  n2 = call "Create All Message Queues.vi"() -> ("error out"=w1:errorcluster, "Message Queues out"=w11:T11)  [unwired: 10 in]
  n3 = register-events(error in=w18, w14) -> (reference out=w15:refnum<event-registration>, error out=w13:errorcluster)  [unwired: 1 in]
  n4 = local read "退出"() -> (w2:T7)
  n5 = Unbundle By Name(w11) -> ("UI"=w8:refnum<queue>, "Acquisition"=w10:refnum<queue>, "Logging"=w5:refnum<queue>)
  n6 = call "TCPServer.vi"("错误输入（无错误）"=w1, "stop"=w2) -> ()  [unwired: 8 in, 2 out]
  n7 = while {
    tunnel: w14 -> [w31]
    tunnel: w13 -> [w30]
    tunnel: [w29] -> w12
    tunnel: w8 -> [w27]
    tunnel: w1 -> [w26]
    shift-right: [w21] -> _
    shift-left: State."Idle" ("State") -> [w22]
    stop <- w28 stop-if-true
    n8 = call "Dequeue Message.vi"("error in (no error)"=w26, "Message Queue"=w27) -> ("error out"=w23:errorcluster, "Message"=w25:string, "dup Message Queue"=w24:refnum<queue>)  [unwired: 6 in, 1 out]
    n9 = case shown="默认" w25 {
      tunnel: w31 -> [_ _ w52 _ _]
      tunnel: w30 -> [w33 w37 w63 w65 w71]
      tunnel: [w33 w36 w56 w64 w71] -> w29
      tunnel: [_ _ _ TRUE _] -> w28
      tunnel: w24 -> [_ w39 w60 w66 _]
      tunnel: w23 -> [_ w38 w59 _ _]
      tunnel: w22 -> [w32 w34 w61 w68 w70]
      tunnel: [w32 w35 w61 w68 w70] -> w21
      frame "Initialize" {
      }
      frame "Start" {
        n10 = case shown="\"Idle\", 默认" w34 {
          selector: w34 -> [_ w50]
          tunnel: w39 -> [w46 _]
          tunnel: w38 -> [w45 w47]
          tunnel: [w44 w49] -> w36
          tunnel: [w40 w50] -> w35
          tunnel: w37 -> [w41 w48]
          frame "Idle", Default {
            w40 = State."Timing"  # State
            n11 = call-poly "Enqueue Message.vi"("error in (no error)"=w45, "Message"="Timing", "Message Queue"=w46) -> ("error out"=w43:errorcluster)  [unwired: 7 in, 1 out]
            n12 = Merge Errors(w41, w43) -> (w44:errorcluster)
          }
          frame "Timing" {
            n13 = Merge Errors(w48, w47) -> (w49:errorcluster)
          }
        }
      }
      frame "Timing" {
        n14 = local read "定时采样信息D"() -> (w54:string[][])
        n15 = Wait (ms)(milliseconds to wait=u32 1000 ("等待时间（毫秒）")) -> ()  [unwired: 1 out]
        n16 = call "TimeSampleVI.vi"("定时采样信息D"=w54, "错误输入（无错误）"=w63, "TimeSample"=w52, "开启定时采样"=TRUE) -> ("错误输出"=w57:errorcluster, "布尔"=→"定时检测事件":bool)  [unwired: 5 in, 1 out]
        n17 = call-poly "Enqueue Message.vi"("error in (no error)"=w59, "Message"="Timing", "Message Queue"=w60) -> ("error out"=w58:errorcluster)  [unwired: 7 in, 1 out]
        n18 = Merge Errors(w57, w58) -> (w56:errorcluster)
      }
      frame "Exit" {
        n19 = Release Queue(queue=w66, error in (no error)=w65) -> (error out=w67:errorcluster)  [unwired: 1 in, 2 out]
        n20 = Merge Errors(w65, w67) -> (w64:errorcluster)
      }
      frame Default {
      }
    }
  }
  n21 = local write "退出"(FALSE) -> ()
  n22 = while {
    tunnel: [w82] -> _
    shift-right: [w76] -> _
    shift-left: State."Idle" ("State") -> [w77]
    shift-right: [w74] -> _
    shift-left: 0 -> [w75]
    tunnel: w5 -> [w73]
    tunnel: w1 -> [w72]
    stop <- w81 stop-if-true
    # "进度条"
    n23 = call "Dequeue Message.vi"("error in (no error)"=w72, "Message Queue"=w73) -> ("error out"=w78:errorcluster, "Message"=w80:string, "dup Message Queue"=w79:refnum<queue>)  [unwired: 6 in, 1 out]
    n24 = case shown="\"Exit\"" w80 {
      tunnel: [w84 w89 w107 w116 w131 w137] -> w82
      tunnel: [_ _ _ _ TRUE _] -> w81
      tunnel: w79 -> [_ w91 w110 w118 w132 _]
      tunnel: w78 -> [w84 w90 w109 w117 _ w137]
      tunnel: w77 -> [w85 w87 w111 w114 w134 w138]
      tunnel: [w85 w88 w111 w115 w134 w138] -> w76
      tunnel: w75 -> [w83 _ w103 _ w130 w136]
      tunnel: [w83 w86 w102 w113 w130 w136] -> w74
      frame "Initialize" {
      }
      frame "StartSample" {
        n25 = case shown="\"Idle\", 默认" w87 {
          selector: w87 -> [_ w101]
          tunnel: w91 -> [w98 _]
          tunnel: w90 -> [w97 w99]
          tunnel: [w96 w100] -> w89
          tunnel: [State."SamplingAndSaving" ("State") w101] -> w88
          tunnel: [0 _] -> w86
          frame "Idle", Default {
            n26 = call-poly "Enqueue Message.vi"("error in (no error)"=w97, "Message"="SamplingAndSaving", "Message Queue"=w98) -> ("error out"=w95:errorcluster)  [unwired: 7 in, 1 out]
            n27 = Merge Errors(w95) -> (w96:errorcluster)
          }
          frame "SamplingAndSaving" {
            n28 = Merge Errors(w99) -> (w100:errorcluster)
          }
        }
      }
      frame "SamplingAndSaving" {
        n29 = Add(x=w103, y=10) -> (x+y=w102:i32)
        "采样过程中 ... 请不要进行其它操作" <- w102
        n30 = Wait (ms)(milliseconds to wait=u32 1000 ("等待时间（毫秒）")) -> ()  [unwired: 1 out]
        n31 = property on="采样过程中 ... 请不要进行其它操作" class="Slide (严格)"("Visible"=TRUE) -> ()  [unwired: 2 in, 2 out]
        n32 = call-poly "Enqueue Message.vi"("error in (no error)"=w109, "Message"="SamplingAndSaving", "Message Queue"=w110) -> ("error out"=w108:errorcluster)  [unwired: 7 in, 1 out]
        n33 = Merge Errors(w108) -> (w107:errorcluster)
        n34 = call "SamplingAndSavingDlg.vi"("采样过程中...in"=w102) -> ()  [unwired: 11 in]
      }
      frame "StopSample" {
        n35 = case shown="\"SamplingAndSaving\"" w114 {
          selector: w114 -> [w121 _]
          tunnel: w118 -> [_ w126]
          tunnel: w117 -> [w120 w125]
          tunnel: [w122 w128] -> w116
          tunnel: [w121 State."Idle" ("State")] -> w115
          tunnel: [0 0] -> w113
          frame "Idle", Default {
            n36 = Merge Errors(w120) -> (w122:errorcluster)
          }
          frame "SamplingAndSaving" {
            n37 = flat-sequence {
              frame #0 {
              }
              frame #1 {
                n38 = property on="采样过程中 ... 请不要进行其它操作" class="Slide (严格)"("Visible"=FALSE) -> ()  [unwired: 2 in, 2 out]
              }
            }
            n39 = Flush Queue(queue=w126, error in (no error)=w125) -> (error out=w124:errorcluster)  [unwired: 2 out]
            n40 = Merge Errors(w124) -> (w128:errorcluster)
          }
        }
      }
      frame "Exit" {
        n41 = Release Queue(queue=w132) -> (error out=w133:errorcluster)  [unwired: 2 in, 2 out]
        n42 = Merge Errors(w133) -> (w131:errorcluster)
      }
      frame Default {
      }
    }
  }
  n43 = call <vilib>:"Add State(s) to Queue__JKI_lib_State_Machine.vi"("State(s) in (\"\")"="Macro: Initialize") -> ("States Out"=w20:string)  [unwired: 14 in]
  n44 = case shown="无错误" w1 {
    selector: w1 -> [w142 w224]
    tunnel: [w143 w224] -> _
    tunnel: w10 -> [w139 _]
    frame No Error {
      n45 = while {
        tunnel: [w154] -> w143
        tunnel: w142 -> [w147]
        shift-right: [w152] -> _
        shift-left: State."Idle" ("State") -> [w151]
        shift-right: [w153] -> _
        shift-left: T12 {"Max Input"=10.0, "Min Input"=-10.0, "Sample Rate"=5000.0, "Sample Num"=5000.0, "DAQmx Task"="", "物理通道"="Dev17/ao0"} ("Hardware Configuration") -> [w145]
        tunnel: w139 -> [w146]
        stop <- w150 stop-if-true
        # "AO输出"
        n46 = call "Dequeue Message.vi"("error in (no error)"=w147, "Message Queue"=w146) -> ("error out"=w148:errorcluster, "Message"=w144:string, "dup Message Queue"=w149:refnum<queue>)  [unwired: 6 in, 1 out]
        n47 = case shown="\"AOoutputting\"" w144 {
          tunnel: [w156 w160 w193 w199 w215 w221] -> w154
          tunnel: w145 -> [w158 w161 w196 w197 w213 w223]
          tunnel: [w158 w159 w195 w197 w213 w223] -> w153
          tunnel: w148 -> [w157 w163 w190 w203 w218 w222]
          tunnel: [w155 w164 w188 w200 w217 w220] -> w152
          tunnel: w151 -> [w155 w165 w188 w201 w217 w220]
          tunnel: w149 -> [_ w162 w191 w202 w219 _]
          tunnel: [_ _ _ _ TRUE _] -> w150
          frame "Initialize" {
            # "初始化  - 初始化当前不包含任何操作。硬件初始化在“开始”消息中进行。"
            n48 = Merge Errors(w157) -> (w156:errorcluster)
          }
          frame "Start" {
            n49 = case shown="\"Idle\", 默认" w165 {
              selector: w165 -> [_ w177]
              tunnel: [w176 w179] -> w160
              tunnel: w161 -> [w170 w178]
              tunnel: w163 -> [w169 w179]
              tunnel: w162 -> [w174 _]
              tunnel: [w166 w178] -> w159
              tunnel: [State."AOoutputting" ("State") w177] -> w164
              frame "Idle", Default {
                # "编辑这些VI，对采集进行配置。"
                # "如系统处于空闲状态，则开始采集。"
                n50 = call "Initialize Hardware References.vi"("error in (no error)"=w169, "Hardware Resources in"=w170) -> ("error out"=w168:errorcluster, "Hardware Resources out"=w167:T13)  [unwired: 8 in]
                n51 = call "Configure Hardware.vi"("error in (no error)"=w168, "Hardware Resources in"=w167) -> ("error out"=w173:errorcluster, "Hardware Resources out"=w166:T13)  [unwired: 8 in]
                n52 = call-poly "Enqueue Message.vi"("error in (no error)"=w169, "Message"="AOoutputting", "Message Queue"=w174) -> ("error out"=w175:errorcluster)  [unwired: 7 in, 1 out]
                n53 = Merge Errors(w173, w175) -> (w176:errorcluster)
              }
              frame "AOoutputting" {
                # "系统已开始采集。忽略“开始”消息。"
              }
            }
          }
          frame "AOoutputting" {
            w184 = u16 0 items=["正弦波", "三角波", "方波", "锯齿波"] ("波形类型")
            # "这一部分需要修改的 AO输出与AI采集不一样"
            n54 = local read "输出电压值"() -> (w183:string)
            n55 = local read "电压频率"() -> (w181:string)
            n56 = Fract/Exp String To Number(string=w181) -> (number=w180:dbl)  [unwired: 3 in, 1 out]
            n57 = Fract/Exp String To Number(string=w183) -> (number=w182:dbl)  [unwired: 3 in, 1 out]
            n58 = Bundle By Name(cluster=cluster{"波形类型":u16, "幅值":dbl, "频率":dbl} {"波形类型"=0, "幅值"=1.0, "频率"=1.0} ("簇"), "波形类型"=w184, "幅值"=w182, "频率"=w180) -> (w186:cluster{"波形类型":u16, "幅值":dbl, "频率":dbl})
            n59 = Build Array(w186) -> (w185:cluster{"波形类型":u16, "幅值":dbl, "频率":dbl}[])
            n60 = call "AOoutput.vi"("error in (no error)"=w190, "波形参数"=w185, "Hardware Resources in"=w196) -> ("error out"=w194:errorcluster, "Hardware Resources out"=w195:T13)  [unwired: 6 in, 1 out]
            n61 = call-poly "Enqueue Message.vi"("error in (no error)"=w190, "Message"="AOoutputting", "Message Queue"=w191) -> ("error out"=w189:errorcluster)  [unwired: 7 in, 1 out]
            n62 = Merge Errors(w194, w189) -> (w193:errorcluster)
          }
          frame "Stop" {
            n63 = case shown="\"AOoutputting\"" w201 {
              selector: w201 -> [w205 _]
              tunnel: w203 -> [w204 w211]
              tunnel: w202 -> [_ w210]
              tunnel: [w205 State."Idle" ("State")] -> w200
              tunnel: [w204 w206] -> w198
              tunnel: w197 -> [_ w208]
              frame "Idle", Default {
                # "系统已处于空闲状态。忽略“停止”消息。"
              }
              frame "AOoutputting" {
                # "如系统处于采集状态，则停止采集。"
                n64 = Flush Queue(queue=w210, error in (no error)=w211) -> (error out=w207:errorcluster)  [unwired: 2 out]
                n65 = call "Stop Acquisition.vi"("error in (no error)"=w207, "Hardware Resources in"=w208) -> ("error out"=w206:errorcluster)  [unwired: 9 in]
              }
            }
            n66 = Merge Errors(w198) -> (w199:errorcluster)
          }
          frame "Exit" {
            # "释放采集队列引用"
            n67 = Release Queue(queue=w219, error in (no error)=w218) -> (error out=w214:errorcluster)  [unwired: 1 in, 2 out]
            n68 = call "Stop Acquisition.vi"("Hardware Resources in"=w213) -> ("error out"=w212:errorcluster)  [unwired: 10 in]
            n69 = Merge Errors(w212, w214) -> (w215:errorcluster)
          }
          frame Default {
            # "初始化  - 初始化当前不包含任何操作。硬件初始化在“开始”消息中进行。"
            n70 = Merge Errors(w222) -> (w221:errorcluster)
          }
        }
      }
    }
    frame Error {
    }
  }
  n71 = while "JKI - String-Based Queued State Machine (Basic) v1.0" {
    shift-right: [w233] -> _
    shift-left: _ -> [w232]
    shift-right: [w236] -> _
    shift-left: _ -> [w230]
    shift-right: [w235] -> _
    shift-left: w20 -> [w237]
    tunnel: w15 -> [w229]
    tunnel: w10 -> [w228]
    tunnel: w1 -> [w227]
    tunnel: w8 -> [w226]
    tunnel: w5 -> [w225]
    stop <- w234 stop-if-true
    w231 = -1  # Timeout
    n72 = call <vilib>:"Parse State Queue__JKI_lib_State_Machine.vi"("State Queue"=w237, "Error In (no error)"=w230) -> ("Remaining States"=w239:string, "Current State"=w240:string, "Arguments"=w238:string)  [unwired: 11 in]
    n73 = case shown="\"HW:ClosePowerOutput\"" w240 {
      selector: w240 -> [_ _ w438 _ _ _ _ _ _ _ _ _ _ _ _ _ _ _ _ _ _ _ _ _ _ _ _ _ _ _ _ _ _ _ _ _ _ _ _ _ _ _ _ _ _ _ _ _ _ _ _ _ _ _ _ _ _ _ _ _ _ _ _ _ _ _ _ _ _ _ _ _ _ _ _ _ _ _ _ _ _ _]
      tunnel: w239 -> [w250 w437 w442 w460 w466 w471 w475 w508 w514 w518 w524 w530 w541 w567 w572 w588 w592 w596 w600 w604 w616 w627 w861 w1095 w1103 w1222 w1326 w1430 w1530 w1582 w1595 w1599 w1607 w1615 w1622 w1632 w1659 w1669 w1687 w1698 w1706 w1715 w1722 w1729 w1733 w1756 w1765 w1773 w1789 w1803 w1810 w1814 w1824 w1837 w1842 w1847 w1852 w1857 w1862 w1867 w1871 w1879 w1926 w1949 w1969 w2008 w2025 w2128 w2138 w2148 w2159 w2170 w2181 w2192 w2203 w2214 w2225 w2236 w2247 w2258 w2269 w2277]
      tunnel: w238 -> [_ _ _ _ _ _ _ _ _ _ _ w525 w535 _ _ _ _ _ _ _ _ _ _ _ _ _ _ _ _ _ _ _ w1600 _ _ w1623 _ w1665 _ w1692 _ _ _ _ _ _ _ _ _ _ _ _ _ _ _ _ _ _ _ _ _ w1875 _ _ _ w2003 w2022 _ _ _ _ _ _ _ _ _ _ _ _ _ _ _]
      tunnel: w232 -> [w248 w434 w440 w451 w463 w469 w472 _ w509 w515 w522 w528 w537 w564 w569 w585 w589 w593 w597 w601 w613 w624 w858 w1093 w1100 w1219 w1323 w1427 w1527 w1579 w1590 w1596 w1604 w1613 w1619 w1629 w1653 w1663 w1685 w1696 w1703 w1712 w1719 w1726 w1730 w1744 w1761 w1770 w1775 w1797 w1807 w1811 w1820 w1835 w1840 w1845 w1850 w1855 w1860 w1865 w1868 w1874 w1923 w1943 w1952 w1995 w2021 w2122 w2130 w2140 w2150 w2161 w2172 w2183 w2194 w2205 w2216 w2227 w2238 w2249 w2260 w2271]
      tunnel: [w247 w435 w444 w457 errorcluster {"status"=FALSE, "code"=0, "source"=""} ("error out") w468 w473 w505 w510 w516 w521 w526 w538 w565 w570 w586 w590 w594 w598 w602 w614 w625 w859 w1085 w1101 w1220 w1324 w1428 w1528 w1580 w1593 w1597 w1605 w1608 w1620 w1630 w1655 w1667 w1677 w1693 w1704 w1713 w1720 w1727 w1731 w1754 w1762 w1771 w1777 w1800 w1808 w1812 w1821 w1833 w1838 w1843 w1848 w1853 w1858 w1863 w1869 w1872 w1924 w1947 w1967 w2006 w2018 w2118 w2136 w2146 w2157 w2168 w2179 w2190 w2201 w2212 w2223 w2234 w2245 w2256 w2267 w2273] -> w236
      tunnel: w230 -> [w246 w435 w443 w457 w462 w468 w473 w505 w511 w516 w521 w527 w539 w565 w570 w586 w590 w594 w598 w602 w614 w625 w859 w1085 w1101 w1220 w1324 w1428 w1528 w1580 w1593 w1597 w1605 w1609 w1620 w1630 w1656 w1667 w1677 w1694 w1704 w1713 w1720 w1727 w1731 w1754 w1763 w1771 w1777 w1801 w1808 w1812 w1822 w1834 w1839 w1844 w1849 w1854 w1859 w1864 w1869 w1873 w1924 w1947 w1967 w2006 w2019 w2118 w2136 w2146 w2157 w2168 w2179 w2190 w2201 w2212 w2223 w2234 w2245 w2256 w2267 w2274]
      tunnel: [w249 w436 w441 w459 w465 w470 w474 w507 w513 w517 w523 w529 w540 w566 w571 w587 w591 w595 w599 w603 w615 w626 w860 w1094 w1102 w1221 w1325 w1429 w1529 w1581 w1594 w1598 w1606 w1614 w1621 w1631 w1658 w1668 w1686 w1697 w1705 w1714 w1721 w1728 w1732 w1755 w1764 w1772 w1788 w1802 w1809 w1813 w1823 w1836 w1841 w1846 w1851 w1856 w1861 w1866 w1870 w1878 w1925 w1948 w1968 w2007 w2024 w2127 w2137 w2147 w2158 w2169 w2180 w2191 w2202 w2213 w2224 w2235 w2246 w2257 w2268 w2276] -> w235
      tunnel: [_ _ _ _ _ TRUE _ _ _ _ _ _ _ _ _ _ _ _ _ _ _ _ _ _ _ _ _ _ _ _ _ _ _ _ _ _ _ _ _ _ _ _ _ _ _ _ _ _ _ _ _ _ _ _ _ _ _ _ _ _ _ _ _ _ _ _ _ _ _ _ _ _ _ _ _ _ _ _ _ _ _ _] -> w234
      tunnel: [w245 w434 w440 w458 w463 w469 w472 w506 w509 w515 w522 w528 w537 w564 w569 w585 w589 w593 w597 w601 w613 w624 w858 w1093 w1100 w1219 w1323 w1427 w1527 w1579 w1589 w1596 w1604 w1613 w1619 w1629 w1652 w1663 w1685 w1696 w1703 w1712 w1719 w1726 w1730 w1743 w1760 w1770 w1774 w1796 w1807 w1811 w1819 w1835 w1840 w1845 w1850 w1855 w1860 w1865 w1868 w1874 w1922 w1943 w1951 w1987 w2021 w2126 w2129 w2139 w2149 w2160 w2171 w2182 w2193 w2204 w2215 w2226 w2237 w2248 w2259 w2270] -> w233
      tunnel: w231 -> [w244 _ _ _ _ _ _ _ _ _ _ _ _ _ _ _ _ _ _ _ _ _ _ _ _ _ _ _ _ _ _ _ _ _ _ _ _ _ _ _ _ _ _ _ _ _ _ _ _ _ _ _ _ _ _ _ _ _ _ _ _ _ _ _ _ _ _ _ _ _ _ _ _ _ _ _ _ _ _ _ _ _]
      tunnel: w229 -> [w243 _ _ _ _ _ _ _ _ _ _ _ _ _ _ _ _ _ _ _ _ _ _ _ _ _ _ _ _ _ _ _ _ _ _ _ _ _ _ _ _ _ _ _ _ _ _ _ _ _ _ _ _ _ _ _ _ _ _ _ _ _ _ _ _ _ _ _ _ _ _ _ _ _ _ _ _ _ _ _ _ _]
      tunnel: w228 -> [_ _ _ _ _ _ _ _ _ _ _ _ _ _ _ w578 _ _ _ _ _ _ _ _ _ _ _ _ _ _ _ _ _ _ _ _ _ _ _ _ _ _ _ _ _ _ _ _ _ _ _ _ _ _ _ _ _ _ _ _ _ _ w1920 w1946 _ _ _ _ _ _ _ _ _ _ _ _ _ _ _ _ _ _]
      tunnel: w227 -> [w241 _ _ _ _ _ _ _ _ _ _ _ _ _ _ w575 _ _ _ _ _ _ _ _ _ _ _ _ _ _ _ _ _ _ _ _ _ _ _ _ _ _ w1717 w1723 _ _ _ _ _ w1793 _ _ _ _ _ _ _ _ _ _ _ _ w1921 w1944 _ _ _ _ _ _ _ _ _ _ _ _ _ _ _ _ _ _]
      tunnel: w226 -> [_ _ _ _ _ _ _ _ _ _ _ _ _ _ _ w577 _ _ _ _ _ _ _ _ _ _ _ _ _ _ _ _ _ _ _ _ _ _ _ _ _ _ w1718 _ _ _ _ _ _ _ _ _ _ _ _ _ _ _ _ _ _ _ _ _ _ _ _ _ _ _ _ _ _ _ _ _ _ _ _ _ _ _]
      tunnel: w225 -> [w242 _ _ _ _ _ _ _ _ _ _ _ _ _ _ w576 _ _ _ _ _ _ _ _ _ _ _ _ _ _ _ _ _ _ _ _ _ _ _ _ _ _ _ w1725 _ _ _ _ _ w1792 _ _ _ _ _ _ _ _ _ _ _ _ _ _ _ _ _ _ _ _ _ _ _ _ _ _ _ _ _ _ _ _]
      frame "", "Event Structure", "Idle" {
        # "executes when the state queue is empty"
        n74 = event shown="[7] \"数据监测界面\": 双击" {
          selector: w243 -> [_ _ _ _ _ _ _ _ _ _ _ _ _ _ _ _ _ _ _ _]
          dyn-events: _ -> [_ _ _ _ _ _ _ _ _ _ _ _ _ _ _ _ _ _ _ _]
          timeout: w244 -> [_ _ _ _ _ _ _ _ _ _ _ _ _ _ _ _ _ _ _ _]
          tunnel: w250 -> [w254 w261 w269 w275 w308 w313 w318 w331 w340 w382 w387 w392 w397 w402 w407 w412 w417 w422 w427 w433]
          tunnel: [w253 w260 w268 w274 w307 w312 w317 w330 w339 w381 w386 w391 w396 w401 w406 w411 w416 w421 w426 w432] -> w249
          tunnel: w248 -> [w251 w258 w266 w272 w301 w310 w315 w324 w333 w379 w384 w389 w394 w399 w404 w409 w414 w419 w424 w430]
          tunnel: [w252 w259 w267 w273 w306 w311 w316 w329 w338 w380 w385 w390 w395 w400 w405 w410 w415 w420 w425 w431] -> w247
          tunnel: w246 -> [w252 w259 w267 w273 w306 w311 w316 w329 w338 w380 w385 w390 w395 w400 w405 w410 w415 w420 w425 w431]
          tunnel: [w251 w258 w266 w272 w300 w310 w315 w323 w332 w379 w384 w389 w394 w399 w404 w409 w414 w419 w424 w430] -> w245
          tunnel: w242 -> [_ _ _ _ w303 _ _ _ _ _ _ _ _ _ _ _ _ _ _ _]
          tunnel: w241 -> [_ _ _ _ w302 _ _ _ _ _ _ _ _ _ _ _ _ _ _ _]
          event Timeout {
            n75 = event-data() -> ()  [unwired: 1 in, 1 out]
            n76 = call <vilib>:"Add State(s) to Queue__JKI_lib_State_Machine.vi"("State(s) in (\"\")"=w254) -> ("States Out"=w253:string)  [unwired: 14 in]
          }
          event Value Change {
            n77 = event-data() -> ("NewVal"=w257:T1)  [unwired: 1 in, 5 out]
            n78 = case shown="真" w257 {
              tunnel: [0 1] -> w256
              tunnel: ["jiemian:GengxinJiemian" "jiemian:chushihuaSampleInfo"] -> w255
              frame False {
                (unwired) "Jiemian:Chushihua"
                # "Jiemian:Chushihua"
              }
              frame True {
              }
            }
            n79 = local write "选项卡控件"(w256) -> ()
            n80 = call <vilib>:"Add State(s) to Queue__JKI_lib_State_Machine.vi"("State(s) in Front (\"\")"=w255, "State(s) in (\"\")"=w261) -> ("States Out"=w260:string)  [unwired: 13 in]
          }
          event "选项卡控件": Value Change {
            n81 = event-data() -> ()  [unwired: 1 in, 6 out]
            n82 = call <vilib>:"Add State(s) to Queue__JKI_lib_State_Machine.vi"("State(s) in (\"\")"=w269) -> ("States Out"=w268:string)  [unwired: 14 in]
          }
          event Menu Selection (User) {
            n83 = event-data() -> ("ItemTag"=w271:string)  [unwired: 1 in, 6 out]
            "项标识符" <- w271
            n84 = case shown="\"帮助(H)\", 默认" w271 {
              tunnel: ["Congfig:helpDlg" "" "" "Macro: Exit" "Macro: Exit" "ManualSample:ManualTestingDialog>>About" "TimeSample:TimeSampleDialog" "Config:SampleInfoManage" "Config:PowerControlDlg" "Config:Launch Area_configDialog" "Config:Launch Dete_configDialog" "Config:Launch Power_configDialog" "Config:Launch DSCManDialog" "Config:Launch DscDistDialog" "Config:ChaxuConfigInfo"] -> w270
              frame "帮助(H)", Default {
              }
              frame "数据监测" {
                n85 = local write "选项卡控件"(0) -> ()
              }
              frame "数据显示" {
                n86 = local write "选项卡控件"(1) -> ()
              }
              frame "ExitExit" {
              }
              frame "ExitE" {
              }
              frame "手动检测" {
              }
              frame "定时检测" {
              }
              frame "检测记录查询" {
              }
              frame "电源控制" {
              }
              frame "区域配置" {
              }
              frame "检测电极配置" {
              }
              frame "供电电极配置" {
              }
              frame "DSC板配置" {
              }
              frame "DSC板电极分配" {
              }
              frame "配置信息查询" {
              }
            }
            n87 = call <vilib>:"Add State(s) to Queue__JKI_lib_State_Machine.vi"("State(s) in Front (\"\")"=w270, "State(s) in (\"\")"=w275) -> ("States Out"=w274:string)  [unwired: 13 in]
          }
          event User Event {
            (unwired) "TimeSample:GetSampleInfo\nDatabase:InsertSampleInfo>>TimeSample\nHW:OpenPowerElec>>ManualSample\nHW:Acquire\nDatabase:InsertSampleData>>TimeSample\nHW:ConfigAndAcquire01\nDatabase:InsertSampleData>>TimeSample\nHW:ConfigAndAcquire02\nDatabase:InsertSampleData>>TimeSample\nHW:ConfigAndAcquire03\nDatabase:InsertSampleData>>TimeSample\nHW:ConfigAndAcquire04\nDatabase:InsertSampleData>>TimeSample\nHW:ConfigAndAcquire05\nDatabase:InsertSampleData>>TimeSample\nHW:ConfigAndAcquire06\nDatabase:InsertSampleData>>TimeSample\nHW:ConfigAndAcquire07\nDatabase:InsertSampleData>>TimeSample\nHW:ConfigAndAcquire08\nDatabase:InsertSampleData>>TimeSample\nHW:ConfigAndAcquire09\nDatabase:InsertSampleData>>TimeSample\nHW:ConfigAndAcquire10\nDatabase:InsertSampleData>>TimeSample\nHW:ConfigAndAcquire11\nDatabase:InsertSampleData>>TimeSample\nHW:ConfigAndAcquire12\nDatabase:InsertSampleData>>TimeSample\nDatabase:GetSampleInfoFromDataBase"
            n88 = event-data() -> ("区域名称"=w299:string, "采样位置"=w298:string, "采样时间"=w297:string, "时"=w296:string, "分"=w294:string)  [unwired: 1 in, 4 out]
            n89 = Decimal String To Number(string=w294) -> (number=w293:i32)  [unwired: 2 in, 1 out]
            n90 = Decimal String To Number(string=w296) -> (number=w295:i32)  [unwired: 2 in, 1 out]
            n91 = Bundle By Name(cluster=w301, "定时采样信息.检测区域"=w299, "定时采样信息.供电位置"=w298, "时分"=w297, "定时采样信息.分钟"=w293, "定时采样信息.时"=w295) -> (w300:T21)
            n92 = call-poly "Enqueue Message.vi"("error in (no error)"=w302, "Message"="StartSample", "Message Queue"=w303) -> ()  [unwired: 7 in, 2 out]
            n93 = call <vilib>:"Add State(s) to Queue__JKI_lib_State_Machine.vi"("State(s) in Front (\"\")"="TimeSample:GetSampleInfo\nDatabase:InsertSampleInfo>>TimeSample\nHW:PowerOutput\nHW:OpenPowerElec>>TimeSample\nHW:Acquire\nHW:GetVandAvalue>>TimeSample\nHW:ClosePowerOutput\nHW:ClosePowerElec>>TimeSample\nDatabase:InsertSampleVandA>>TimeSample\nDatabase:InsertSampleData>>TimeSample\nDatabase:GetSampleInfoFromDataBase\nSample:StopSample\njiemian:GengxinJiemian", "State(s) in (\"\")"=w308) -> ("States Out"=w307:string)  [unwired: 13 in]
          }
          event "SampleInfo": Value Change {
            n94 = event-data() -> ()  [unwired: 1 in, 6 out]
            n95 = call <vilib>:"Add State(s) to Queue__JKI_lib_State_Machine.vi"("State(s) in Front (\"\")"="Config:SampleInfoManage", "State(s) in (\"\")"=w313) -> ("States Out"=w312:string)  [unwired: 13 in]
          }
          event Value Change {
            n96 = event-data() -> ()  [unwired: 1 in, 6 out]
            n97 = call <vilib>:"Add State(s) to Queue__JKI_lib_State_Machine.vi"("State(s) in Front (\"\")"="Config:ChaxuConfigInfo", "State(s) in (\"\")"=w318) -> ("States Out"=w317:string)  [unwired: 13 in]
          }
          event "数据监测界面": Double Click {
            (unwired) "Databases:GetSampleData\nDraw:Drawing3DGraph\n3D:Drawing3DSurfaceGraph\nDraw:Drawing3DDlg"
            # "查询当前行所对应时间存储的数据"
            n98 = event-data() -> ("Row"=w327:i32)  [unwired: 1 in, 8 out]
            n99 = property on="数据监测界面" class="MCListbox (严格)"() -> ("ItemNames"=w328:string[][])  [unwired: 2 in, 2 out]
            n100 = Index Array(array=w328, index (row)=w327) -> (element=w321:string[])  [unwired: 1 in]
            n101 = Index Array(array=w321, index=0 ("索引")) -> (element=w325:string)
            n102 = Index Array(array=w321, index=1) -> (element=w319:string)
            n103 = Bundle By Name(cluster=w324, "SampleInfoTime"=w325, "Area_name"=w319) -> (w323:T21)
            n104 = call <vilib>:"Add State(s) to Queue__JKI_lib_State_Machine.vi"("State(s) in Front (\"\")"="Databases:GetSampleData\nDraw:Drawing3DGraph\nDraw:Drawing3DDlg", "State(s) in (\"\")"=w331) -> ("States Out"=w330:string)  [unwired: 13 in]
          }
          event "数据监测界面": Shortcut Menu Selection (User) {
            (unwired) "Databases:GetSampleData\nDraw:Drawing3DGraph\n3D:Drawing3DSurfaceGraph\nDraw:Drawing3DDlg"
            # "查询当前行所对应时间存储的数据"
            n105 = event-data() -> ("ItemTag"=w337:string, "Coords"=w335:T22)  [unwired: 1 in, 6 out]
            n106 = invoke on="数据监测界面" class="MCListbox (严格)" method="Point To Row Column"("Point"=w335) -> ("CellPosition"=w334:T23)  [unwired: 6 in, 6 out]
            n107 = case shown="\"无泄漏\"" w337 {
              tunnel: ["jiemian:genxinjianceshuju" "Databases:DeleteOneSampleInfo\nDatabase:GetSampleInfoFromDataBase\nDatabase:DeleteSampleData\n" "Config:SampleInfoManage" "Databases:GetSampleData\nDraw:Drawing3DGraph\nDraw:Drawing3DDlg" _ "Database:UpdateLeakageInfo>>无泄漏\nDatabase:GetSampleInfoFromDataBase" "Database:UpdateLeakageInfo>>可疑\nDatabase:GetSampleInfoFromDataBase" "Database:UpdateLeakageInfo>>泄露\nDatabase:GetSampleInfoFromDataBase"] -> w336
              tunnel: w334 -> [_ w348 _ w355 _ w364 w370 w376]
              tunnel: w333 -> [w342 w346 w349 w353 w359 w361 w367 w373]
              tunnel: [w342 w345 w349 w352 w359 w360 w366 w372] -> w332
              frame "刷新", Default {
                (unwired) "Database:GetSampleInfoFromDataBase"
                # "获取所有采样信息"
              }
              frame "删除" {
                # "删除选中的采样信息记录"
                n108 = control-ref of="数据监测界面"() -> (w343:refnum<vi>)
                n109 = call "GetSampleTime.vi"("CellPosition"=w348, "MulticolumnListbox输入"=w343) -> ("SampleTime"=w347:string)  [unwired: 8 in, 1 out]
                n110 = Bundle By Name(cluster=w346, "SampleInfoTime"=w347) -> (w345:T21)
              }
              frame "记录管理" {
              }
              frame "漏洞分析" {
                # "5是曲面图\n4是网格图\n3是等高线图"
                n111 = control-ref of="数据监测界面"() -> (w356:refnum<vi>)
                n112 = disable-structure shown="禁用" {
                  frame Disabled {
                    n113 = local write "选项卡控件"(5) -> ()
                  }
                  frame Enabled {
                  }
                }
                n114 = call "GetSampleTime.vi"("CellPosition"=w355, "MulticolumnListbox输入"=w356) -> ("Area_name"=w351:string, "SampleTime"=w354:string)  [unwired: 8 in]
                n115 = Bundle By Name(cluster=w353, "SampleInfoTime"=w354, "Area_name"=w351) -> (w352:T21)
              }
              frame "预判确认" {
              }
              frame "无泄漏" {
                n116 = control-ref of="数据监测界面"() -> (w363:refnum<vi>)
                n117 = call "GetSampleTime.vi"("CellPosition"=w364, "MulticolumnListbox输入"=w363) -> ("SampleTime"=w362:string)  [unwired: 8 in, 1 out]
                n118 = Bundle By Name(cluster=w361, "SampleInfoTime"=w362) -> (w360:T21)
              }
              frame "可疑" {
                n119 = control-ref of="数据监测界面"() -> (w369:refnum<vi>)
                n120 = call "GetSampleTime.vi"("CellPosition"=w370, "MulticolumnListbox输入"=w369) -> ("SampleTime"=w368:string)  [unwired: 8 in, 1 out]
                n121 = Bundle By Name(cluster=w367, "SampleInfoTime"=w368) -> (w366:T21)
              }
              frame "泄漏" {
                n122 = control-ref of="数据监测界面"() -> (w375:refnum<vi>)
                n123 = call "GetSampleTime.vi"("CellPosition"=w376, "MulticolumnListbox输入"=w375) -> ("SampleTime"=w374:string)  [unwired: 8 in, 1 out]
                n124 = Bundle By Name(cluster=w373, "SampleInfoTime"=w374) -> (w372:T21)
              }
            }
            n125 = call <vilib>:"Add State(s) to Queue__JKI_lib_State_Machine.vi"("State(s) in Front (\"\")"=w336, "State(s) in (\"\")"=w340) -> ("States Out"=w339:string)  [unwired: 13 in]
          }
          event Value Change {
            (unwired) "Config:PowerControlDlg\nHW:PowerOutput\nHW:GetVandA"
            n126 = event-data() -> ()  [unwired: 1 in, 6 out]
            n127 = call <vilib>:"Add State(s) to Queue__JKI_lib_State_Machine.vi"("State(s) in Front (\"\")"="Config:PowerControlDlg", "State(s) in (\"\")"=w382) -> ("States Out"=w381:string)  [unwired: 13 in]
          }
          event Value Change {
            n128 = event-data() -> ()  [unwired: 1 in, 6 out]
            n129 = call <vilib>:"Add State(s) to Queue__JKI_lib_State_Machine.vi"("State(s) in Front (\"\")"="ManualSample:ManualTestingDialog>>About", "State(s) in (\"\")"=w387) -> ("States Out"=w386:string)  [unwired: 13 in]
          }
          event Value Change {
            n130 = event-data() -> ()  [unwired: 1 in, 6 out]
            n131 = call <vilib>:"Add State(s) to Queue__JKI_lib_State_Machine.vi"("State(s) in Front (\"\")"="TimeSample:TimeSampleDialog", "State(s) in (\"\")"=w392) -> ("States Out"=w391:string)  [unwired: 13 in]
          }
          event "区域配置": Value Change {
            n132 = event-data() -> ()  [unwired: 1 in, 6 out]
            n133 = call <vilib>:"Add State(s) to Queue__JKI_lib_State_Machine.vi"("State(s) in Front (\"\")"="Config:Launch Area_configDialog", "State(s) in (\"\")"=w397) -> ("States Out"=w396:string)  [unwired: 13 in]
          }
          event "检测电极配置": Value Change {
            n134 = event-data() -> ()  [unwired: 1 in, 6 out]
            n135 = call <vilib>:"Add State(s) to Queue__JKI_lib_State_Machine.vi"("State(s) in Front (\"\")"="Config:Launch Dete_configDialog", "State(s) in (\"\")"=w402) -> ("States Out"=w401:string)  [unwired: 13 in]
          }
          event "供电电极配置": Value Change {
            n136 = event-data() -> ()  [unwired: 1 in, 6 out]
            n137 = call <vilib>:"Add State(s) to Queue__JKI_lib_State_Machine.vi"("State(s) in Front (\"\")"="Config:Launch Power_configDialog", "State(s) in (\"\")"=w407) -> ("States Out"=w406:string)  [unwired: 13 in]
          }
          event Value Change {
            n138 = event-data() -> ()  [unwired: 1 in, 6 out]
            n139 = call <vilib>:"Add State(s) to Queue__JKI_lib_State_Machine.vi"("State(s) in Front (\"\")"="Config:Launch DSCManDialog", "State(s) in (\"\")"=w412) -> ("States Out"=w411:string)  [unwired: 13 in]
          }
          event "采集板分配电极": Value Change {
            n140 = event-data() -> ()  [unwired: 1 in, 6 out]
            n141 = call <vilib>:"Add State(s) to Queue__JKI_lib_State_Machine.vi"("State(s) in Front (\"\")"="Config:Launch DscDistDialog", "State(s) in (\"\")"=w417) -> ("States Out"=w416:string)  [unwired: 13 in]
          }
          event "设置按钮": Value Change {
            n142 = event-data() -> ()  [unwired: 1 in, 6 out]
            n143 = call <vilib>:"Add State(s) to Queue__JKI_lib_State_Machine.vi"("State(s) in Front (\"\")"="HW:Configure", "State(s) in (\"\")"=w422) -> ("States Out"=w421:string)  [unwired: 13 in]
          }
          event Value Change {
            # "Exit Button Value Change (pressed) Event\n(this executes Macro: Exit to terminate the VI)"
            n144 = event-data() -> ()  [unwired: 1 in, 1 out]
            n145 = call <vilib>:"Add State(s) to Queue__JKI_lib_State_Machine.vi"("State(s) in Front (\"\")"="Macro: Exit", "State(s) in (\"\")"=w427) -> ("States Out"=w426:string)  [unwired: 13 in]
          }
          event Panel Close? {
            # "Discard the event because we'll close the front panel ourselves in Macro: Exit"
            # "Close Panel button (pressed) Event\n(this executes Macro: Exit to terminate the VI)"
            n146 = event-data() -> ()  [unwired: 1 in, 1 out]
            n147 = call <vilib>:"Add State(s) to Queue__JKI_lib_State_Machine.vi"("State(s) in Front (\"\")"="Macro: Exit", "State(s) in (\"\")"=w433) -> ("States Out"=w432:string)  [unwired: 13 in]
            n148 = event-data("Discard?"=TRUE) -> ()  [unwired: 1 in, 1 out]
          }
        }
      }
      frame "---------- Core ----------" {
        # "Do not put any code in this frame.\n(it is a separator no-op)"
        n149 = call <vilib>:"Add State(s) to Queue__JKI_lib_State_Machine.vi"("State(s) in (\"\")"=w437) -> ("States Out"=w436:string)  [unwired: 14 in]
      }
      frame Default {
        w447 = 42 items=["No error", "Argument error", "Memory is full", "Out of zone", "End of file", "File already open", "Generic file I/O error", "File not found", "File permission error", "Disk is full", "Duplicate path", "Too many files open", "System feature not enabled", "Resource file not found", "Cannot add resource", "Resource not found", "Image not found", "Image memory error", "Pen does not exist", "Config type invalid", "Config token not found", "Config parse error", "Config memory error", "Bad external code format", "Bad external code offset", "External code not present", "Null window", "Destroy window error", "Null menu", "Print aborted", "Bad print record", "Print driver error", "Windows error during printing", "Memory error during printing", "Print dialog error", "Generic print error", "Invalid device refnum", "Device not found", "Device parameter error", "Device unit error", "Cannot open device", "Device call aborted", "Generic error", "Cancelled by user", "Object ID too low", "Object ID too high", "Object not in heap", "Unknown heap", "Unknown object (invalid DefProc)", "Unknown object (DefProc not in table)", "Message out of range", "Invalid (null) method", "Unknown message", "Manager call not supported", "Bad address", "Network operation in progress", "Network operation timed out", "Connection is busy", "Network attribute not supported", "Network error", "Address in use", "System out of memory", "Connection aborted", "Connection refused", "Not connected", "Already connected", "Connection closed", "Initialization error (interapplication manager)", "Bad occurrence", "Wait on unbound occurrence handler", "Occurrence queue overflow", "Datalog type conflict", "Unused", "Unrecognized type (interapplication manager)", "Memory corrupt", "Failed to make temporary DLL", "Old CIN version", "Drag socket not found", "Failed to load drop-object", "Failed to register OLE object", "Failed to release OLE object", "Format specifier type mismatch", "Unknown format specifier", "Too few format specifiers", "Too many format specifiers", "Scan failed", "Newer CIN version", "Error converting to variant", "Runtime menu error", "Password tampered", "Variant attribute not found", "Incompatible variant data type", "Event data is not available", "Event Store is not present", "Occurrence is not found", "Event Queue is not created", "Event info is not available", "Refnum passed is NULL", "Error retrieving Class GUID", "Error retrieving CoClass GUID", "Error retrieving TypeLib GUID.", "Bad built application magic bytes.", "Specific driver is different from the specific driver associated with the Logical Name.", "There is no session opened to the class driver.", "Max Error", "MAX - Error with config objects", "MAX - Error loading configuration", "MAX - Group not supported"]
        # "Current State"
        # "Do not delete, rename, or modify this frame.\n(this is used to capture unhandled states and typos)"
        # "Handle mistyped state name (developer tool)"
        n150 = Format Into String(format string="Software Exception: Unhandled State \"%s\"." ("message"), error in=w443, w438) -> (resulting string=w446:string, error out=w445:errorcluster)  [unwired: 1 in]
        n151 = call <vilib>:"Error Cluster From Error Code.vi"("show call chain? (False)"=TRUE, "error in (no error)"=w445, "error message (\"\")"=w446, "error code (0)"=w447) -> ("error out"=w444:errorcluster)  [unwired: 5 in]
        n152 = call <vilib>:"Add State(s) to Queue__JKI_lib_State_Machine.vi"("State(s) in (\"\")"=w442) -> ("States Out"=w441:string)  [unwired: 14 in]
      }
      frame "Initialize Core Data" {
        # "Do not delete, rename, or modify this frame.\n(this is used to determine panel behavior on exit)"
        # "originally closed?"
        # "exe?"
        # "If panel starts closed or is an EXE, then close it when we exit"
        n153 = property class="VI"() -> ("Front Panel.Open"=w456:bool)  [unwired: 2 in, 2 out]
        n154 = property class="App"() -> ("App.Kind"=w455:T14)  [unwired: 2 in, 2 out]
        n155 = control-ref of="Current VI Reference"() -> (w449:refnum<vi>)
        n156 = Not(x=w456) -> (.not. x?=w453:bool)
        n157 = Equal?(x=w455, y=T14."Run Time System" ("Application:Kind")) -> (x = y?=w452:bool)
        n158 = Or(x=w453, y=w452) -> (x .or. y?=w450:bool)
        n159 = Bundle By Name(cluster=w451, "Core.Current VI Reference"=w449, "Core.Close Panel on Exit?"=w450) -> (w458:T21)
        n160 = call <vilib>:"Add State(s) to Queue__JKI_lib_State_Machine.vi"("State(s) in (\"\")"=w460) -> ("States Out"=w459:string)  [unwired: 14 in]
      }
      frame "Error Handler" {
        # "Unhandled Error -- Display it"
        # "Handle any errors here.\nYou can also output any states to clean-up after errors occur"
        # "Clear error"
        n161 = call <vilib>:"General Error Handler.vi"("error in (no error)"=w462) -> ()  [unwired: 10 in, 5 out]
        n162 = call <vilib>:"Add State(s) to Queue__JKI_lib_State_Machine.vi"("State(s) in Front (\"\")"="/* Post Error States", "State(s) in (\"\")"=w466) -> ("States Out"=w465:string)  [unwired: 13 in]
      }
      frame "Exit" {
        # "Do not put any code in this frame.\n(No errors that occur here will be handled.)"
        n163 = call <vilib>:"Add State(s) to Queue__JKI_lib_State_Machine.vi"("State(s) in (\"\")"=w471) -> ("States Out"=w470:string)  [unwired: 14 in]
      }
      frame "---------- Data ----------" {
        # "Do not put any code in this frame.\n(It is a separator no-op. You can make a copy of this frame to create a new Data frame)"
        n164 = call <vilib>:"Add State(s) to Queue__JKI_lib_State_Machine.vi"("State(s) in (\"\")"=w475) -> ("States Out"=w474:string)  [unwired: 14 in]
      }
      frame "Data: Initialize" {
        w476 = ""  # 手动采样到AO电压
        w477 = ""  # 基准电压
        w478 = ""  # 电压系数
        w479 = ""  # Area_name
        w480 = ""  # 回来电流
        w481 = ""  # 回来电压
        w482 = ""  # 电压倍数
        w483 = ""  # 时分
        w484 = ""  # power_f
        w485 = TRUE  # 是否存在记录
        w486 = 0  # 记录数
        w487 = TRUE  # PowTN
        w488 = T24 {"", "采样时间"="", "检测区域"="", "供电位置"="", "采样方式"="", "", "", "电源电压"="", "电源电流"="", "备注"=""}  # TimeSampleInfo
        w489 = T17 {"Dev1ASData"={"DevChSampData"=[], "dscAddress"=""}, "Dev2ASData"={"DevChSampData"=[], "dscAddress"=""}, "Dev3ASData"={"DevChSampData"=[], "dscAddress"=""}, "Dev4ASData"={"DevChSampData"=[], "dscAddress"=""}, "Dev5ASData"={"DevChSampData"=[], "dscAddress"=""}, "Dev6ASData"={"DevChSampData"=[], "dscAddress"=""}, "Dev7ASData"={"DevChSampData"=[], "dscAddress"=""}, "Dev8ASData"={"DevChSampData"=[], "dscAddress"=""}, "Dev9ASData"={"DevChSampData"=[], "dscAddress"=""}, "Dev10ASData"={"DevChSampData"=[], "dscAddress"=""}, "Dev11ASData"={"DevChSampData"=[], "dscAddress"=""}, "Dev12ASData"={"DevChSampData"=[], "dscAddress"=""}, "Dev13ASData"={"DevChSampData"=[], "dscAddress"=""}}  # DevNASSData
        w490 = T25 {"Dev1SampData"=[], "Dev2SampData"=[], "Dev3SampData"=[], "Dev4SampData"=[], "Dev5SampData"=[], "Dev6SampData"=[], "Dev7SampData"=[], "Dev8SampData"=[], "Dev9SampData"=[], "Dev10SampData"=[], "Dev11SampData"=[], "Dev12SampData"=[], "Dev13SampData"=[]}  # nCHData
        (unwired) T26 {"采样时间"="", "", "检测区域"="", "供电位置"="", "采样方式"="", "电源电压"="", "", "电源电流"="", "", "备注"=""}  # TimeSampleInfo
        w491 = T27 {"检测区域"="2区", "检测频率"="每天采样", "时"=10, "分钟"=26, "供电位置"="下层膜检测", "是否启动"="是", "备注"=""}  # 定时采样信息
        w492 = cluster{"X":dbl[], "Y":dbl[], "Z":dbl[]} {"X"=[], "Y"=[], "Z"=[]}  # 3DData
        w494 = ""  # SampleInfoTime
        w495 = cluster{"通道编号":string, "Data":dbl}[] []  # DevChSampData
        w496 = T28 {"数据采集模块地址"="", "0ChData"={"通道编号"="", "Data"=0.0}, "1ChData"={"通道编号"="", "Data"=0.0}, "2ChData"={"通道编号"="", "Data"=0.0}, "3ChData"={"通道编号"="", "Data"=0.0}, "4ChData"={"通道编号"="", "Data"=0.0}, "5ChData"={"通道编号"="", "Data"=0.0}, "6ChData"={"通道编号"="", "Data"=0.0}, "7ChData"={"通道编号"="", "Data"=0.0}, "8ChData"={"通道编号"="", "Data"=0.0}, "9ChData"={"通道编号"="", "Data"=0.0}, "10ChData"={"通道编号"="", "Data"=0.0}, "11ChData"={"通道编号"="", "Data"=0.0}, "12ChData"={"通道编号"="", "Data"=0.0}, "13ChData"={"通道编号"="", "Data"=0.0}, "14ChData"={"通道编号"="", "Data"=0.0}, "15ChData"={"通道编号"="", "Data"=0.0}, "16ChData"={"通道编号"="", "Data"=0.0}, "17ChData"={"通道编号"="", "Data"=0.0}, "18ChData"={"通道编号"="", "Data"=0.0}, "19ChData"={"通道编号"="", "Data"=0.0}, "20ChData"={"通道编号"="", "Data"=0.0}, "21ChData"={"通道编号"="", "Data"=0.0}, "22ChData"={"通道编号"="", "Data"=0.0}, "23ChData"={"通道编号"="", "Data"=0.0}, "24ChData"={"通道编号"="", "Data"=0.0}, "25ChData"={"通道编号"="", "Data"=0.0}, "26ChData"={"通道编号"="", "Data"=0.0}, "27ChData"={"通道编号"="", "Data"=0.0}, "28ChData"={"通道编号"="", "Data"=0.0}, "29ChData"={"通道编号"="", "Data"=0.0}, "30ChData"={"通道编号"="", "Data"=0.0}, "31ChData"={"通道编号"="", "Data"=0.0}}  # DevChSampleData
        w497 = waveform(dbl)[] []  # AcquireData
        w498 = dbl[] []  # SampleData
        w499 = T29 {"", "date/time string"="", "选定检测区域"="", "采样位置"="", "检测方式"="", "", "", "电源电压"="", "电源电流"="", "备注"=""}  # ManualSampleInfo
        w500 = T30 {"选定检测区域"="", "采样位置"="", "电源电压"="", "电源电流"="", "电源频率"="", "检测方式"="", "备注"=""}  # 手动采样信息
        w501 = T18 {"Hardware Configuration"={"Physical Channel"="", "Maximum Input"=0.0, "Minimum Input"=0.0, "Sample Rate"=0.0, "Number of Samples"=0}, "Analysis Configuration"={"Statistics"=TRUE}, "New Data Behavior"=enum."Replace", "HWInfo"=""}  # User Specified
        w502 = T31 {"Current VI Reference"=refnum, "Close Panel on Exit?"=FALSE}  # Core
        w504 = TRUE  # Your Boolean data
        w503 = ""  # Your string data
        # "Data names and types of shift register data are defined by this bundle."
        # "Initialize the shift-register data, here.\n(data names are defined by what you wire into the bundle function)"
        n165 = call <vilib>:"Add State(s) to Queue__JKI_lib_State_Machine.vi"("State(s) in (\"\")"=w508) -> ("States Out"=w507:string)  [unwired: 14 in]
        n166 = Bundle("Core"=w502, "Your Boolean data"=w504, "Your string data"=w503, "User Specified"=w501, "手动采样信息"=w500, "ManualSampleInfo"=w499, "SampleData"=w498, "AcquireData"=w497, "DevChSampleData"=w496, "DevChSampData"=w495, "SampleInfoTime"=w494, "SampleData"=string[][] [["001", "39", "0", "-1"], ["102", "37", "0", "0"], ["103", "40", "2", "1"], ["104", "38", "2", "2"], ["105", "36", "2", "3"], ["106", "41", "4", "4"], ["107", "39", "4", "4"], ["108", "37", "4", "5"], ["109", "35", "4", "6"], ["110", "40", "6", "7"], ["111", "36", "6", "7"], ["112", "41", "8", "8"], ["113", "39", "8", "8"], ["114", "37", "8", "9"], ["115", "35", "8", "9"], ["116", "40", "10", "9"], ["117", "38", "10", "9"], ["118", "36", "10", "10"], ["119", "34", "10", "10"], ["120", "39", "12", "10"], ["121", "37", "12", "9"], ["122", "40", "14", "10"], ["123", "38", "14", "9"], ["124", "36", "14", "9"], ["125", "41", "16", "9"], ["126", "39", "16", "8"], ["127", "37", "16", "8"], ["128", "35", "16", "7"], ["129", "40", "18", "7"], ["130", "36", "17.75", "6"], ["131", "70", "0", "6"], ["132", "60", "0", "5"], ["133", "50", "0", "-1"], ["134", "40", "8", "0"], ["135", "32", "8", "1"], ["136", "40", "0", "2"], ["137", "32", "0", "3"], ["138", "40", "8", "4"], ["139", "32", "8", "4"], ["140", "40", "0", "5"], ["141", "70", "0", "6"], ["142", "60", "0", "7"], ["201", "33", "0", "7"], ["202", "31", "0", "8"], ["203", "34", "2", "8"], ["204", "32", "2", "9"], ["205", "30", "2", "9"], ["206", "28", "2", "9"], ["207", "33", "4", "9"], ["208", "31", "4", "10"], ["209", "29", "4", "10"], ["210", "27", "4", "10"], ["211", "34", "6", "9"], ["212", "30", "6", "10"], ["213", "28", "6", "9"], ["214", "33", "8", "9"], ["215", "31", "8", "9"], ["216", "29", "8", "8"], ["217", "27", "8", "8"], ["218", "32", "10", "7"], ["219", "30", "10", "7"], ["220", "28", "10", "6"], ["221", "33", "12", "6"], ["222", "31", "12", "5"], ["223", "34", "14", "-1"], ["224", "32", "14", "0"], ["225", "30", "14", "1"], ["226", "28", "14", "2"], ["227", "33", "16", "3"], ["228", "31", "16", "4"], ["229", "29", "16", "4"], ["230", "34", "17.5", "5"], ["231", "30", "17", "6"], ["232", "28", "17", "7"], ["233", "40", "0", "7"], ["234", "30", "0", "8"], ["235", "24", "8", "8"], ["236", "16", "8", "9"], ["237", "24", "0", "9"], ["238", "16", "0", "9"], ["239", "24", "8", "9"], ["240", "32", "0", "10"], ["241", "24", "0", "10"], ["242", "16", "0", "10"], ["243", "50", "0", "9"], ["244", "40", "0", "10"], ["245", "30", "0", "9"], ["301", "23", "27", "9"], ["302", "24", "25", "9"], ["303", "25", "21", "8"], ["304", "26", "19", "8"], ["305", "27", "26", "7"], ["306", "28", "24", "7"], ["307", "29", "22", "6"], ["308", "30", "20", "6"], ["309", "31", "18", "5"], ["310", "32", "25", "-1"], ["311", "33", "23", "0"], ["312", "34", "21", "1"], ["313", "35", "19", "2"], ["314", "36", "17", "3"], ["315", "37", "24", "4"], ["316", "38", "22", "4"], ["317", "39", "18", "5"], ["318", "40", "25", "6"], ["319", "41", "23", "7"], ["320", "42", "21", "7"], ["321", "43", "19", "8"], ["322", "44", "26", "8"], ["323", "45", "24", "9"], ["324", "46", "22", "9"], ["325", "47", "20", "9"], ["326", "48", "18", "9"], ["327", "49", "27", "10"], ["328", "50", "25", "10"], ["329", "51", "21", "10"], ["330", "52", "19", "9"], ["331", "53", "26", "10"], ["332", "54", "24", "9"], ["333", "55", "22", "9"], ["334", "56", "20", "9"], ["335", "57", "27", "8"], ["336", "58", "25", "8"], ["337", "59", "23", "7"], ["338", "60", "21", "7"], ["339", "61", "19", "6"], ["340", "24", "17", "6"], ["341", "22", "17", "5"], ["342", "18", "17.5", "-1"], ["401", "15", "0", "0"], ["402", "13", "0", "1"], ["403", "16", "2", "2"], ["404", "14", "2", "3"], ["405", "12", "2", "4"], ["406", "15", "4", "4"], ["", "", "", "5"], ["408", "11", "4", "6"], ["409", "16", "6", "7"], ["410", "12", "6", "7"], ["411", "47", "8", "8"], ["412", "15", "8", "8"], ["413", "13", "8", "9"], ["414", "11", "8", "9"], ["415", "16", "10", "9"], ["416", "14", "10", "9"], ["417", "12", "10", "10"], ["418", "10", "10", "10"], ["419", "15", "12", "10"], ["420", "13", "12", "9"], ["421", "18", "14", "10"], ["422", "16", "14", "9"], ["423", "14", "14", "9"], ["424", "12", "14", "9"], ["425", "17", "16", "8"], ["426", "15", "16", "8"], ["427", "13", "16", "7"], ["428", "16", "17.5", "7"], ["429", "12", "18", "6"], ["430", "10", "18", "6"], ["431", "30", "0", "5"], ["432", "20", "0", "-1"], ["433", "0", "0", "0"], ["434", "8", "0", "1"], ["435", "0", "0", "2"], ["436", "16", "8", "3"], ["437", "8", "8", "4"], ["438", "0", "8", "4"], ["439", "20", "0", "5"], ["440", "10", "0", "6"], ["441", "0", "0", "7"], ["501", "10", "2", "7"], ["502", "8", "2", "8"], ["503", "6", "2", "8"], ["504", "4", "2", "9"], ["505", "2", "2", "9"], ["506", "0", "2", "9"], ["507", "9", "4", "9"], ["508", "7", "4", "10"], ["509", "5", "4", "10"], ["510", "3", "4", "10"], ["511", "1", "4", "9"], ["512", "10", "6", "10"], ["513", "6", "6", "9"], ["514", "4", "6", "9"], ["515", "2", "6", "9"], ["516", "0", "6", "8"], ["517", "9", "8", "8"], ["518", "7", "8", "7"], ["519", "5", "8", "7"], ["520", "3", "8", "6"], ["521", "1", "8", "6"], ["522", "8", "10", "5"], ["523", "6", "10", "-1"], ["524", "4", "10", "0"], ["525", "2", "10", "1"], ["526", "0", "10", "2"], ["527", "9", "12", "3"], ["528", "7", "12", "4"], ["529", "3", "12", "4"], ["530", "1", "12", "5"], ["531", "0", "18", "6"], ["532", "10", "14", "7"], ["533", "8", "14", "7"], ["534", "6", "14", "8"], ["535", "4", "14", "8"], ["536", "2", "14", "9"], ["537", "0", "14", "9"], ["538", "11", "16", "9"], ["539", "9", "16", "9"], ["540", "7", "16", "10"], ["541", "5", "16", "10"], ["542", "3", "16", "10"], ["543", "1", "16", "9"], ["544", "6", "18", "10"], ["545", "4", "18", "9"], ["", "", "", "9"], ["", "", "", "9"], ["", "", "", "8"], ["", "", "", "8"], ["", "", "", "7"], ["", "", "", "7"], ["", "", "", "6"], ["", "", "", "6"], ["", "", "", "5"]], "3DData"=w492, "定时采样信息"=w491, "TimeSampleInfo"=w488, "nCHData"=w490, "DevNASSData"=w489, "PowTN"=w487, "记录数"=w486, "是否存在记录"=w485, "power_f"=w484, "时分"=w483, "电压倍数"=w482, "回来电压"=w481, "回来电流"=w480, "Area_name"=w479, "电压系数"=w478, "基准电压"=w477, "手动采样到AO电压"=w476) -> (w506:T21)  [unwired: 1 in]
      }
      frame "Data: Cleanup" {
        # "Cleanup any data and references, here.\n(this is called automatically, by the Macro: Exit)"
        n167 = Unbundle By Name(w509) -> ("Core.Current VI Reference"=w512:refnum<vi>)
        n168 = Close Reference(reference=w512, error in (no error)=w511) -> (error out=w510:errorcluster)
        n169 = call <vilib>:"Add State(s) to Queue__JKI_lib_State_Machine.vi"("State(s) in (\"\")"=w514) -> ("States Out"=w513:string)  [unwired: 14 in]
      }
      frame "---------- UI ----------" {
        # "Do not put any code in this frame.\n(It is a separator no-op. You can make a copy of this frame to create a new UI frame)"
        n170 = call <vilib>:"Add State(s) to Queue__JKI_lib_State_Machine.vi"("State(s) in (\"\")"=w518) -> ("States Out"=w517:string)  [unwired: 14 in]
      }
      frame "UI: Initialize" {
        (unwired) "Database:GetSampleInfoFromDataBase\nJiemian:Chushihua"
        # "Initialize the User Interface, here.\n(this is called automatically, by the Macro: Init)"
        n171 = property on="采样过程中 ... 请不要进行其它操作" class="Slide (严格)"("Visible"=FALSE) -> ()  [unwired: 2 in, 2 out]
        n172 = call <vilib>:"Add State(s) to Queue__JKI_lib_State_Machine.vi"("State(s) in Front (\"\")"="jiemian:chushihuaSampleInfo\nJiemian:Chushihua", "State(s) in (\"\")"=w524) -> ("States Out"=w523:string)  [unwired: 13 in]
      }
      frame "UI: Cursor Set" {
        # "Argument"
        # "Set and Unset Cursor Busy.\n(Usage: \"UI: Cursor Set >> Busy|Idle\")"
        n173 = case shown="\"Idle\", 默认" w525 {
          tunnel: w527 -> [w532 w534]
          tunnel: [w531 w533] -> w526
          frame "Idle", Default {
            n174 = call <vilib>:"Unset Busy.vi"("error in (no error)"=w532) -> ("error out"=w531:errorcluster)  [unwired: 10 in]
          }
          frame "Busy" {
            n175 = call <vilib>:"Set Busy.vi"("error in (no error)"=w534) -> ("error out"=w533:errorcluster)  [unwired: 9 in, 1 out]
          }
        }
        n176 = call <vilib>:"Add State(s) to Queue__JKI_lib_State_Machine.vi"("State(s) in (\"\")"=w530) -> ("States Out"=w529:string)  [unwired: 14 in]
      }
      frame "UI: Front Panel State" {
        # "Argument"
        # "Set Front Panel Open or Closed\n(Usage: \"UI: Front Panel State >> Open|Close\")"
        n177 = Unbundle By Name(w537) -> ("Core.Current VI Reference"=w536:refnum<vi>)
        n178 = case shown="\"Open\", 默认" w535 {
          tunnel: w539 -> [w545 w558]
          tunnel: [w547 w559] -> w538
          tunnel: w536 -> [w546 w556]
          frame "Open", Default {
            n179 = property class="VI"(reference=w546, error in=w545) -> (reference out=w543:refnum<vi>, error out=w544:errorcluster, "Front Panel.Open"=w542:bool)
            n180 = case shown="假" w542 {
              tunnel: [w550 w553] -> w547
              tunnel: w544 -> [w549 w553]
              tunnel: w543 -> [w548 _]
              frame False {
                n181 = invoke class="VI" method="FP.Open"(reference=w548, error in=w549, "Activate"=TRUE, "State"=T15."Standard") -> (error out=w550:errorcluster)  [unwired: 1 in, 4 out]
              }
              frame True {
              }
            }
          }
          frame "Close" {
            n182 = property class="VI"(reference=w556, error in=w558) -> (reference out=w555:refnum<vi>, error out=w557:errorcluster, "Front Panel.Open"=w554:bool)
            n183 = case shown="真" w554 {
              tunnel: [w560 w563] -> w559
              tunnel: w557 -> [w560 w562]
              tunnel: w555 -> [_ w561]
              frame False {
              }
              frame True {
                n184 = invoke class="VI" method="FP.Close"(reference=w561, error in=w562) -> (error out=w563:errorcluster)  [unwired: 1 in, 2 out]
              }
            }
          }
        }
        n185 = call <vilib>:"Add State(s) to Queue__JKI_lib_State_Machine.vi"("State(s) in (\"\")"=w541) -> ("States Out"=w540:string)  [unwired: 14 in]
      }
      frame "---------- Macro ----------" {
        # "Do not put any code in this frame.\n(It is a separator no-op. You can make a copy of this frame to create a new Macro frame)"
        n186 = call <vilib>:"Add State(s) to Queue__JKI_lib_State_Machine.vi"("State(s) in (\"\")"=w567) -> ("States Out"=w566:string)  [unwired: 14 in]
      }
      frame "Macro: Initialize" {
        w568 = "Data: Initialize\nInitialize Core Data\nUI: Initialize\nUI: Front Panel State >> Open\nSample:LoadSampleSetInfo\nSample:StartTimeSample"  # Data: Initialize Initialize Core Data UI: Initialize UI: Front Panel State >> Open Sample:LoadSampleSetInfo Sample:StartTimeSample
        # "Initialization Macro\n(This is called once, when the VI starts)"
        n187 = call <vilib>:"Add State(s) to Queue__JKI_lib_State_Machine.vi"("State(s) in Front (\"\")"=w568, "State(s) in (\"\")"=w572) -> ("States Out"=w571:string)  [unwired: 13 in]
      }
      frame "Macro: Exit" {
        w573 = TRUE ("Priority Message? (F)")
        w574 = "Exit"
        # "Exit Macro\n(This is called once, when the VI exits)"
        n188 = Unbundle By Name(w585) -> ("Core.Close Panel on Exit?"=w584:bool)
        n189 = call-poly "Enqueue Message.vi"("Priority Message? (F)"=w573, "error in (no error)"=w575, "Message"=w574, "Message Queue"=w578) -> ()  [unwired: 6 in, 2 out]
        n190 = call-poly "Enqueue Message.vi"("Priority Message? (F)"=w573, "error in (no error)"=w575, "Message"=w574, "Message Queue"=w576) -> ()  [unwired: 6 in, 2 out]
        n191 = call-poly "Enqueue Message.vi"("Priority Message? (F)"=w573, "error in (no error)"=w575, "Message"=w574, "Message Queue"=w577) -> ()  [unwired: 6 in, 2 out]
        n192 = Select(t="UI: Front Panel State >> Close", s=w584, f="") -> (s? t:f=w581:string)
        n193 = call <vilib>:"Add State(s) to Queue__JKI_lib_State_Machine.vi"("State(s) in (\"\")"=w581, "State(s) at Back (\"\")"="Data: Cleanup\nExit") -> ("States Out"=w579:string)  [unwired: 13 in]
        n194 = call <vilib>:"Add State(s) to Queue__JKI_lib_State_Machine.vi"("State(s) in Front (\"\")"=w579, "State(s) in (\"\")"=w588) -> ("States Out"=w587:string)  [unwired: 13 in]
      }
      frame "---------- New Category ----------" {
        # "Template Separator\n(You can make a copy of, or modify, this frame)"
        n195 = call <vilib>:"Add State(s) to Queue__JKI_lib_State_Machine.vi"("State(s) in (\"\")"=w592) -> ("States Out"=w591:string)  [unwired: 14 in]
      }
      frame "New Category: 1" {
        # "Your code here.\n(You can make a copy of, or modify, this frame)"
        n196 = call <vilib>:"Add State(s) to Queue__JKI_lib_State_Machine.vi"("State(s) in (\"\")"=w596) -> ("States Out"=w595:string)  [unwired: 14 in]
      }
      frame "New Category: 2" {
        # "Your code here.\n(You can make a copy of, or modify, this frame)"
        n197 = call <vilib>:"Add State(s) to Queue__JKI_lib_State_Machine.vi"("State(s) in (\"\")"=w600) -> ("States Out"=w599:string)  [unwired: 14 in]
      }
      frame "------------Jiemian--------------" {
        # "Your code here.\n(You can make a copy of, or modify, this frame)"
        n198 = call <vilib>:"Add State(s) to Queue__JKI_lib_State_Machine.vi"("State(s) in (\"\")"=w604) -> ("States Out"=w603:string)  [unwired: 14 in]
      }
      frame "jiemian:genxinjianceshuju" {
        # "Your code here.\n(You can make a copy of, or modify, this frame)"
        n199 = call "SelectData.vi"("SQL query"="select * from t_sample_info;") -> ("recordset data"=w609:variant[][])  [unwired: 7 in, 1 out]
        n200 = call "ReadDataFromDatabase.vi"("长度"=10, "index"=0, "recordset data"=w609) -> ("所有记录"=w607:string[][])  [unwired: 7 in, 1 out]
        n201 = control-ref of="数据监测界面"() -> (w606:refnum<vi>)
        n202 = Array Subset(array=w607, index (col)=1 ("禁用的索引 (列)")) -> (w611:string[][])  [unwired: 3 in]
        n203 = property on="属性节点" class="MCListbox (严格)"(reference=w606, "ItemNames"=w611) -> ()  [unwired: 1 in, 2 out]
        n204 = call <vilib>:"Add State(s) to Queue__JKI_lib_State_Machine.vi"("State(s) in (\"\")"=w616) -> ("States Out"=w615:string)  [unwired: 14 in]
      }
      frame "Jiemian:Chushihua" {
        # "Your code here.\n(You can make a copy of, or modify, this frame)"
        n205 = call "SelectData.vi"("SQL query"="select area_name from t_area;") -> ("recordset data"=w622:variant[][])  [unwired: 7 in, 1 out]
        n206 = local write "选项卡控件"(0) -> ()
        n207 = call "ReadDataFromDatabase.vi"("长度"=1, "index"=0, "recordset data"=w622) -> ("所有记录"=w619:string[][])  [unwired: 7 in, 1 out]
        n208 = for {
          N: 2 -> [_]
          tunnel: w619 -> [w638] mode=indexing
          i -> [w632]
          n209 = call "GetSampleTime.vi"("所有记录输入"=w638) -> ("area_name"=w630:string, "所有记录输出"=w637:string[][])  [unwired: 9 in]
          n210 = Index Array(array=w637, index (row)=0 ("索引 (行)")) -> (element=w635:string[])  [unwired: 1 in]
          n211 = Index Array(array=w635, index=0 ("索引")) -> (element=w629:string)
          n212 = call "GetSampleData.vi"("SampleInfoTime"=w629) -> ("记录数"=w628:i32, "所有记录"=w633:string[][])  [unwired: 7 in, 2 out]
          n213 = call "IndexSampleData.vi"("SampleData"=w633) -> ("SampleDataXYZ"=w631:cluster{"X":dbl[], "Y":dbl[], "Z":dbl[]})  [unwired: 7 in, 3 out]
          n214 = case shown="1" w632 {
            tunnel: w631 -> [w643 w749]
            tunnel: w630 -> [w642 w748]
            tunnel: w629 -> [w641 w747]
            tunnel: w628 -> [w639 w746]
            frame 0, Default {
              n215 = Greater Than 0?(x=w639) -> (x > 0?=w640:bool)
              n216 = case shown="真" w640 {
                tunnel: w643 -> [_ w655]
                tunnel: w642 -> [_ w647]
                tunnel: w641 -> [_ w646]
                frame False {
                  n217 = local write "Info"("无采样数据") -> ()
                }
                frame True {
                  n218 = Unbundle By Name(w655) -> ("X"=w654:dbl[], "Y"=w653:dbl[], "Z"=w652:dbl[])
                  n219 = mathscript code="xi=linspace(min(a),max(a),70);\nyi=linspace(min(b),max(b),27);\n[Xi,Yi]=meshgrid(xi,yi);\nZi=griddata(a,b,c,Xi,Yi,'cubic')"("a"=w654, "b"=w653, "c"=w652) -> ("Xi"=w650:dbl[][], "Yi"=w649:dbl[][], "Zi"=w648:dbl[][])  [unwired: 1 in, 1 out]
                  n220 = call "lianjieStr.vi"("data"=w646, "area_name"=w647) -> ("连接后字符串"=→"Info":string)  [unwired: 9 in]
                  n221 = call-poly <vilib>:"Plot Helper.vi"("z matrix"=w648, "y matrix"=w649, "x matrix"=w650) -> ("3D Plot lvclass Array out"=→"3D Surface":refnum<class "3D Plot Datatype.lvclass">[])  [unwired: 3 in, 5 out]
                }
              }
            }
            frame 1 {
              n222 = Greater Than 0?(x=w746) -> (x > 0?=w745:bool)
              n223 = case shown="真" w745 {
                tunnel: w749 -> [_ w758]
                tunnel: w748 -> [_ w753]
                tunnel: w747 -> [_ w752]
                frame False {
                  n224 = local write "Info 2"("无采样数据") -> ()
                }
                frame True {
                  n225 = Unbundle By Name(w758) -> ("X"=w761:dbl[], "Y"=w760:dbl[], "Z"=w759:dbl[])
                  n226 = call "lianjieStr.vi"("data"=w752, "area_name"=w753) -> ("连接后字符串"=→"Info 2":string)  [unwired: 9 in]
                  n227 = mathscript code="xi=linspace(min(a),max(a),70);\nyi=linspace(min(b),max(b),27);\n[Xi,Yi]=meshgrid(xi,yi);\nZi=griddata(a,b,c,Xi,Yi,'cubic')\n%mesh(Xi,Yi,Zi);\n%grid on\n%surfc(Xi,Yi,Zi);"("a"=w761, "b"=w760, "c"=w759) -> ("Xi"=w756:dbl[][], "Yi"=w755:dbl[][], "Zi"=w754:dbl[][])  [unwired: 1 in, 1 out]
                  n228 = call-poly <vilib>:"Plot Helper.vi"("z matrix"=w754, "y matrix"=w755, "x matrix"=w756) -> ("3D Plot lvclass Array out"=→"3D Surface 3":refnum<class "3D Plot Datatype.lvclass">[])  [unwired: 3 in, 5 out]
                }
              }
            }
          }
        }
        n229 = call <vilib>:"Add State(s) to Queue__JKI_lib_State_Machine.vi"("State(s) in (\"\")"=w627) -> ("States Out"=w626:string)  [unwired: 14 in]
      }
      frame "jiemian:GengxinJiemian" {
        # "Your code here.\n(You can make a copy of, or modify, this frame)"
        n230 = call "SelectData.vi"("SQL query"="select area_name from t_area;") -> ("recordset data"=w856:variant[][])  [unwired: 7 in, 1 out]
        n231 = local write "选项卡控件"(0) -> ()
        n232 = call "ReadDataFromDatabase.vi"("长度"=1, "index"=0, "recordset data"=w856) -> ("所有记录"=w853:string[][])  [unwired: 7 in, 1 out]
        n233 = for {
          N: 2 -> [_]
          tunnel: w853 -> [w872] mode=indexing
          i -> [w866]
          n234 = call "GetSampleTime.vi"("所有记录输入"=w872) -> ("area_name"=w864:string, "所有记录输出"=w871:string[][])  [unwired: 9 in]
          n235 = Index Array(array=w871, index (row)=0 ("索引 (行)")) -> (element=w869:string[])  [unwired: 1 in]
          n236 = Index Array(array=w869, index=0 ("索引")) -> (element=w863:string)
          n237 = call "GetSampleData.vi"("SampleInfoTime"=w863) -> ("记录数"=w862:i32, "所有记录"=w867:string[][])  [unwired: 7 in, 2 out]
          n238 = call "IndexSampleData.vi"("SampleData"=w867) -> ("SampleDataXYZ"=w865:cluster{"X":dbl[], "Y":dbl[], "Z":dbl[]})  [unwired: 7 in, 3 out]
          n239 = case shown="0, 默认" w866 {
            tunnel: w865 -> [w877 w983]
            tunnel: w864 -> [w876 w982]
            tunnel: w863 -> [w875 w981]
            tunnel: w862 -> [w873 w980]
            frame 0, Default {
              n240 = Greater Than 0?(x=w873) -> (x > 0?=w874:bool)
              n241 = case shown="真" w874 {
                tunnel: w877 -> [_ w889]
                tunnel: w876 -> [_ w885]
                tunnel: w875 -> [_ w884]
                frame False {
                  n242 = local write "Info"("无采样数据") -> ()
                }
                frame True {
                  n243 = Unbundle By Name(w889) -> ("X"=w888:dbl[], "Y"=w887:dbl[], "Z"=w886:dbl[])
                  n244 = mathscript code="xi=linspace(min(a),max(a),70);\nyi=linspace(min(b),max(b),27);\n[Xi,Yi]=meshgrid(xi,yi);\nZi=griddata(a,b,c,Xi,Yi,'cubic')"("a"=w888, "b"=w887, "c"=w886) -> ("Xi"=w883:dbl[][], "Yi"=w882:dbl[][], "Zi"=w881:dbl[][])  [unwired: 1 in, 1 out]
                  n245 = call "lianjieStr.vi"("data"=w884, "area_name"=w885) -> ("连接后字符串"=w879:string)  [unwired: 9 in]
                  n246 = local write "Info"(w879) -> ()
                  n247 = call-poly <vilib>:"Plot Helper.vi"("z matrix"=w881, "y matrix"=w882, "x matrix"=w883) -> ("3D Plot lvclass Array out"=w880:refnum<class "3D Plot Datatype.lvclass">[])  [unwired: 3 in, 5 out]
                  n248 = local write "3D Surface"(w880) -> ()
                }
              }
            }
            frame 1 {
              n249 = Greater Than 0?(x=w980) -> (x > 0?=w979:bool)
              n250 = case shown="假" w979 {
                tunnel: w983 -> [_ w992]
                tunnel: w982 -> [_ w988]
                tunnel: w981 -> [_ w987]
                frame False {
                  n251 = local write "Info 2"("无采样数据") -> ()
                }
                frame True {
                  n252 = Unbundle By Name(w992) -> ("X"=w995:dbl[], "Y"=w994:dbl[], "Z"=w993:dbl[])
                  n253 = call "lianjieStr.vi"("data"=w987, "area_name"=w988) -> ("连接后字符串"=w985:string)  [unwired: 9 in]
                  n254 = mathscript code="xi=linspace(min(a),max(a),70);\nyi=linspace(min(b),max(b),27);\n[Xi,Yi]=meshgrid(xi,yi);\nZi=griddata(a,b,c,Xi,Yi,'cubic')\n%mesh(Xi,Yi,Zi);\n%grid on\n%surfc(Xi,Yi,Zi);"("a"=w995, "b"=w994, "c"=w993) -> ("Xi"=w991:dbl[][], "Yi"=w990:dbl[][], "Zi"=w989:dbl[][])  [unwired: 1 in, 1 out]
                  n255 = local write "Info 2"(w985) -> ()
                  n256 = call-poly <vilib>:"Plot Helper.vi"("z matrix"=w989, "y matrix"=w990, "x matrix"=w991) -> ("3D Plot lvclass Array out"=w986:refnum<class "3D Plot Datatype.lvclass">[])  [unwired: 3 in, 5 out]
                  n257 = local write "3D Surface 3"(w986) -> ()
                }
              }
            }
          }
        }
        n258 = call <vilib>:"Add State(s) to Queue__JKI_lib_State_Machine.vi"("State(s) in (\"\")"=w861) -> ("States Out"=w860:string)  [unwired: 14 in]
      }
      frame "jiemian:chushihuaSampleInfo" {
        # "Your code here.\n(You can make a copy of, or modify, this frame)"
        n259 = disable-structure shown="禁用" {
          frame Disabled {
            n260 = call "SelectData.vi"("SQL query"="select *from t_sample_info;") -> ("recordset data"=w1098:variant[][])  [unwired: 7 in, 1 out]
            n261 = call "ReadDataFromDatabase.vi"("长度"=10, "index"=0, "recordset data"=w1098) -> ()  [unwired: 7 in, 2 out]
          }
          frame Enabled {
          }
        }
        n262 = call "SelectData.vi"("SQL query"="select *from t_sample_info;") -> ("recordset data"=w1089:variant[][])  [unwired: 7 in, 1 out]
        n263 = call "ReadDataFromDatabase.vi"("长度"=10, "index"=0, "recordset data"=w1089) -> ("所有记录"=w1086:string[][])  [unwired: 7 in, 1 out]
        n264 = Array Subset(array=w1086, index (col)=1 ("禁用的索引 (列)")) -> (w1091:string[][])  [unwired: 3 in]
        n265 = property on="数据监测界面" class="MCListbox (严格)"("ItemNames"=w1091) -> ()  [unwired: 2 in, 2 out]
        n266 = call <vilib>:"Add State(s) to Queue__JKI_lib_State_Machine.vi"("State(s) in (\"\")"=w1095) -> ("States Out"=w1094:string)  [unwired: 14 in]
      }
      frame "---------------3D----------------" {
        # "Your code here.\n(You can make a copy of, or modify, this frame)"
        n267 = disable-structure shown="禁用" {
          disable-tunnel: w1100 -> [w1107 _]
          frame Disabled {
            n268 = Unbundle By Name(w1107) -> ("3DData.X"=w1106:dbl[], "3DData.Y"=w1105:dbl[], "3DData.Z"=w1104:dbl[])
            n269 = mathscript code="xi=linspace(min(a),max(a),70);\nyi=linspace(min(b),max(b),27);\n[Xi,Yi]=meshgrid(xi,yi);\nZi=griddata(a,b,c,Xi,Yi,'cubic')\nmesh(Xi,Yi,Zi);\ngrid on"("a"=w1106, "b"=w1105, "c"=w1104) -> ()  [unwired: 1 in, 1 out]
          }
          frame Enabled {
          }
        }
        n270 = call <vilib>:"Add State(s) to Queue__JKI_lib_State_Machine.vi"("State(s) in (\"\")"=w1103) -> ("States Out"=w1102:string)  [unwired: 14 in]
      }
      frame "3D:Drawing3DSurfaceGraph" {
        # "3D曲面图\n3D Surface Graph\n3D网格图\n3D Mesh Graph"
        # "Your code here.\n(You can make a copy of, or modify, this frame)"
        n271 = Unbundle By Name(w1219) -> ("3DData.X"=w1218:dbl[], "3DData.Y"=w1217:dbl[], "3DData.Z"=w1216:dbl[], "记录数"=w1215:i32)
        n272 = Greater Than 0?(x=w1215) -> (x > 0?=w1214:bool)
        n273 = case shown="真" w1214 {
          tunnel: w1218 -> [_ w1228]
          tunnel: w1217 -> [_ w1227]
          tunnel: w1216 -> [_ w1226]
          frame False {
          }
          frame True {
            n274 = mathscript code="xi=linspace(min(a),max(a),70);\nyi=linspace(min(b),max(b),27);\n[Xi,Yi]=meshgrid(xi,yi);\nZi=griddata(a,b,c,Xi,Yi,'cubic')\n%mesh(Xi,Yi,Zi);\n%grid on\n%surfc(Xi,Yi,Zi);"("a"=w1228, "b"=w1227, "c"=w1226) -> ("Xi"=w1225:dbl[][], "Yi"=w1223:dbl[][], "Zi"=w1224:dbl[][])  [unwired: 1 in, 1 out]
            n275 = call-poly <vilib>:"Plot Helper.vi"("z matrix"=w1224, "y matrix"=w1223, "x matrix"=w1225) -> ()  [unwired: 3 in, 6 out]
          }
        }
        n276 = call <vilib>:"Add State(s) to Queue__JKI_lib_State_Machine.vi"("State(s) in (\"\")"=w1222) -> ("States Out"=w1221:string)  [unwired: 14 in]
      }
      frame "3D:Drawing3DMeshGraph" {
        # "3D曲面图\n3D Surface Graph\n3D网格图\n3D Mesh Graph\n3D等高线\n3DContourGraph"
        # "Your code here.\n(You can make a copy of, or modify, this frame)"
        n277 = Unbundle By Name(w1323) -> ("3DData.X"=w1322:dbl[], "3DData.Y"=w1321:dbl[], "3DData.Z"=w1320:dbl[], "记录数"=w1319:i32)
        n278 = Greater Than 0?(x=w1319) -> (x > 0?=w1318:bool)
        n279 = case shown="真" w1318 {
          tunnel: w1322 -> [_ w1332]
          tunnel: w1321 -> [_ w1331]
          tunnel: w1320 -> [_ w1330]
          frame False {
          }
          frame True {
            n280 = mathscript code="xi=linspace(min(a),max(a),70);\nyi=linspace(min(b),max(b),27);\n[Xi,Yi]=meshgrid(xi,yi);\nZi=griddata(a,b,c,Xi,Yi,'cubic')\n%mesh(Xi,Yi,Zi);\n%grid on\n%surfc(Xi,Yi,Zi);"("a"=w1332, "b"=w1331, "c"=w1330) -> ("Xi"=w1329:dbl[][], "Yi"=w1328:dbl[][], "Zi"=w1327:dbl[][])  [unwired: 1 in, 1 out]
            n281 = call-poly <vilib>:"Plot Helper.vi"("z matrix"=w1327, "y matrix"=w1328, "x matrix"=w1329) -> ()  [unwired: 3 in, 6 out]
          }
        }
        n282 = call <vilib>:"Add State(s) to Queue__JKI_lib_State_Machine.vi"("State(s) in (\"\")"=w1326) -> ("States Out"=w1325:string)  [unwired: 14 in]
      }
      frame "3D:Drawing3DContourGraph" {
        # "3D曲面图\n3D Surface Graph\n3D网格图\n3D Mesh Graph\n3D等高线\n3DContourGraph"
        n283 = Unbundle By Name(w1427) -> ("3DData.X"=w1426:dbl[], "3DData.Y"=w1425:dbl[], "3DData.Z"=w1424:dbl[], "记录数"=w1423:i32)
        n284 = Greater Than 0?(x=w1423) -> (x > 0?=w1422:bool)
        n285 = case shown="真" w1422 {
          tunnel: w1426 -> [_ w1436]
          tunnel: w1425 -> [_ w1435]
          tunnel: w1424 -> [_ w1434]
          frame False {
          }
          frame True {
            n286 = mathscript code="xi=linspace(min(a),max(a),70);\nyi=linspace(min(b),max(b),27);\n[Xi,Yi]=meshgrid(xi,yi);\nZi=griddata(a,b,c,Xi,Yi,'cubic')\n%mesh(Xi,Yi,Zi);\n%grid on\n%surfc(Xi,Yi,Zi);"("a"=w1436, "b"=w1435, "c"=w1434) -> ("Xi"=w1433:dbl[][], "Yi"=w1432:dbl[][], "Zi"=w1431:dbl[][])  [unwired: 1 in, 1 out]
            n287 = call-poly <vilib>:"Plot Helper.vi"("z matrix"=w1431, "y matrix"=w1432, "x matrix"=w1433) -> ()  [unwired: 3 in, 6 out]
          }
        }
        n288 = call <vilib>:"Add State(s) to Queue__JKI_lib_State_Machine.vi"("State(s) in (\"\")"=w1430) -> ("States Out"=w1429:string)  [unwired: 14 in]
      }
      frame "----------Draw---------" {
        w1526 = i32[] [1, 2, 3, 4, 5, 6, 7, 7]
        # "Your code here.\n(You can make a copy of, or modify, this frame)"
        n289 = mathscript code="%x=[1,2,3,4,5,6,7];\n%y=[1,2,3,4.5,4,5,6]\nplot(x,y)"("x"=w1526, "y"=w1526) -> ()  [unwired: 1 in, 1 out]
        n290 = call <vilib>:"Add State(s) to Queue__JKI_lib_State_Machine.vi"("State(s) in (\"\")"=w1530) -> ("States Out"=w1529:string)  [unwired: 14 in]
      }
      frame "Draw:Drawing3DDlg" {
        # "Your code here.\n(You can make a copy of, or modify, this frame)"
        n291 = Unbundle By Name(w1579) -> ("SampleData"=w1576:string[][], "3DData"=w1578:cluster{"X":dbl[], "Y":dbl[], "Z":dbl[]}, "是否存在记录"=w1577:bool, "SampleInfoTime"=w1575:string, "Area_name"=w1574:string)
        n292 = case shown="真" w1577 {
          selector: w1577 -> [_ w1587]
          tunnel: w1578 -> [_ w1588]
          tunnel: w1576 -> [_ w1586]
          tunnel: w1575 -> [_ w1585]
          tunnel: w1574 -> [_ w1584]
          frame False {
            n293 = One Button Dialog(message="无采集数据可以分析，请重新选择需要分析的采样日期" ("消息")) -> ()  [unwired: 1 in, 1 out]
          }
          frame True {
            (unwired) TRUE ("是否存在记录")
            (unwired) cluster{"X":dbl[], "Y":dbl[], "Z":dbl[]} {"X"=[], "Y"=[], "Z"=[]} ("3DData")
            n294 = call "LeakageFenxi.vi"("采样时间"=w1585, "Area_name"=w1584, "采样数据"=w1586, "是否存在记录"=w1587, "3DData"=w1588) -> ()  [unwired: 7 in]
          }
        }
        n295 = call <vilib>:"Add State(s) to Queue__JKI_lib_State_Machine.vi"("State(s) in (\"\")"=w1582) -> ("States Out"=w1581:string)  [unwired: 14 in]
      }
      frame "Draw:Drawing3DGraph" {
        (unwired) "3D:Drawing3DSurfaceGraph"
        n296 = Unbundle By Name(w1590) -> ("SampleData"=w1592:string[][])
        n297 = call "IndexSampleData.vi"("SampleData"=w1592) -> ("SampleDataXYZ"=w1591:cluster{"X":dbl[], "Y":dbl[], "Z":dbl[]})  [unwired: 7 in, 3 out]
        n298 = Bundle By Name(cluster=w1590, "3DData"=w1591) -> (w1589:T21)
        n299 = call <vilib>:"Add State(s) to Queue__JKI_lib_State_Machine.vi"("State(s) in (\"\")"=w1595) -> ("States Out"=w1594:string)  [unwired: 14 in]
      }
      frame "---------------DataBase------------" {
        # "Your code here.\n(You can make a copy of, or modify, this frame)"
        n300 = call <vilib>:"Add State(s) to Queue__JKI_lib_State_Machine.vi"("State(s) in (\"\")"=w1599) -> ("States Out"=w1598:string)  [unwired: 14 in]
      }
      frame "Database:UpdateLeakageInfo" {
        # "Your code here.\n(更新确认无泄露信息)"
        n301 = Unbundle By Name(w1604) -> ("SampleInfoTime"=w1601:string)
        n302 = Format Into String(format string="update t_sample_info\nset predict_yesno='%s'\nwhere sample_info_time='%s';", w1600, w1601) -> (resulting string=w1602:string)  [unwired: 2 in, 1 out]
        n303 = call "updateData.vi"("SQL query"=w1602) -> ()  [unwired: 10 in, 1 out]
        n304 = call <vilib>:"Add State(s) to Queue__JKI_lib_State_Machine.vi"("State(s) in (\"\")"=w1607) -> ("States Out"=w1606:string)  [unwired: 14 in]
      }
      frame "Database:DeleteSampleData" {
        # "Your code here.\n(You can make a copy of, or modify, this frame)"
        n305 = Unbundle By Name(w1613) -> ("SampleInfoTime"=w1611:string)
        n306 = Format Into String(format string="delete from t_test_data where sample_info_time='%s';", w1611) -> (resulting string=w1610:string)  [unwired: 2 in, 1 out]
        n307 = call "deleteData.vi"("error in"=w1609, "SQL query"=w1610) -> ("error out"=w1608:errorcluster)  [unwired: 9 in]
        n308 = call <vilib>:"Add State(s) to Queue__JKI_lib_State_Machine.vi"("State(s) in (\"\")"=w1615) -> ("States Out"=w1614:string)  [unwired: 14 in]
      }
      frame "Databases:DeleteOneSampleInfo" {
        # "Your code here.\n(You can make a copy of, or modify, this frame)"
        n309 = Unbundle By Name(w1619) -> ("SampleInfoTime"=w1617:string)
        n310 = Format Into String(format string="delete from t_sample_info where sample_info_time='%s';", w1617) -> (resulting string=w1616:string)  [unwired: 2 in, 1 out]
        n311 = call "deleteData.vi"("SQL query"=w1616) -> ()  [unwired: 10 in, 1 out]
        n312 = call <vilib>:"Add State(s) to Queue__JKI_lib_State_Machine.vi"("State(s) in (\"\")"=w1622) -> ("States Out"=w1621:string)  [unwired: 14 in]
      }
      frame "Database:InsertSampleVandA" {
        # "Your code here.\n(把电压值和电流值保存在数据库中)"
        n313 = case shown="\"ManualSample\"" w1623 {
          tunnel: w1629 -> [w1638 w1649]
          tunnel: [w1637 w1648] -> w1625
          tunnel: [w1635 w1645] -> w1627
          tunnel: [w1634 w1647] -> w1626
          frame "TimeSample", Default {
            n314 = Unbundle By Name(w1638) -> ("TimeSampleInfo.采样时间"=w1637:string, "回来电压"=w1636:string, "回来电流"=w1634:string)  [unwired: 1 out]
            n315 = call "GetOutputVandA.vi"("电压系数输入"="0.01", "回来电压"=w1636) -> ("实际输出电压"=w1635:string)  [unwired: 4 in, 5 out]
          }
          frame "ManualSample" {
            n316 = Unbundle By Name(w1649) -> ("ManualSampleInfo.date/time string"=w1648:string, "回来电压"=w1646:string, "回来电流"=w1647:string)  [unwired: 1 out]
            n317 = call "GetOutputVandA.vi"("电压系数输入"="0.01", "回来电压"=w1646) -> (0:"电压系数输出"=→"电压系数输出":dbl, 1:"实际输出电压"=→"实际输出电压":string, "字符串"=w1645:string, 3:"电压系数输出"=→"电压系数":string, "回来电压"=→"回来电压":dbl, 5:"实际输出电压"=→"实际输出电压压":dbl)  [unwired: 4 in]
          }
        }
        n318 = Format Into String(format string="update t_sample_info\nset supply_voltage='%s',supply_current='%s'\nwhere sample_info_time='%s';\n ", w1627, w1626, w1625) -> (resulting string=w1624:string)  [unwired: 2 in, 1 out]
        n319 = call "updateData.vi"("SQL query"=w1624) -> ()  [unwired: 10 in, 1 out]
        n320 = call <vilib>:"Add State(s) to Queue__JKI_lib_State_Machine.vi"("State(s) in (\"\")"=w1632) -> ("States Out"=w1631:string)  [unwired: 14 in]
      }
      frame "Databases:GetSampleData" {
        # "获取对应时间的数据"
        n321 = Unbundle By Name(w1653) -> ("SampleInfoTime"=w1657:string)
        n322 = call "GetSampleData.vi"("错误输入（无错误）"=w1656, "SampleInfoTime"=w1657) -> ("错误输出"=w1655:errorcluster, "是否存在记录"=w1650:bool, "记录数"=w1651:i32, "所有记录"=w1654:string[][])  [unwired: 6 in]
        n323 = Bundle By Name(cluster=w1653, "SampleData"=w1654, "记录数"=w1651, "是否存在记录"=w1650) -> (w1652:T21)
        n324 = call <vilib>:"Add State(s) to Queue__JKI_lib_State_Machine.vi"("State(s) in (\"\")"=w1659) -> ("States Out"=w1658:string)  [unwired: 14 in]
      }
      frame "Database:InsertSampleData" {
        # "Your code here.\n(You can make a copy of, or modify, this frame)"
        n325 = case shown="\"TimeSample\", 默认" w1665 {
          tunnel: w1663 -> [w1673 w1676]
          tunnel: [w1672 w1675] -> w1666
          tunnel: [w1671 w1674] -> w1664
          frame "TimeSample", Default {
            n326 = Unbundle By Name(w1673) -> ("TimeSampleInfo.采样时间"=w1672:string, "TimeSampleInfo.检测区域"=w1671:string)
          }
          frame "ManualSample" {
            n327 = Unbundle By Name(w1676) -> ("ManualSampleInfo.date/time string"=w1675:string, "ManualSampleInfo.选定检测区域"=w1674:string)
          }
        }
        "选定检测区域" <- w1664
        n328 = disable-structure shown="禁用" {
          disable-tunnel: w1663 -> [w1670 _]
          frame Disabled {
            n329 = Unbundle By Name(w1670) -> ()  [unwired: 2 out]
          }
          frame Enabled {
          }
        }
        n330 = Unbundle By Name(w1663) -> ("DevNASSData"=w1662:T17)
        n331 = call "InsertDevDataN.vi"("DevNASSData"=w1662, "选定检测区域"=w1664, "date/time string"=w1666) -> ("detec_electrode_name"=→"detec_electrode_name":string, "elecNum"=→"elecNum":i32)  [unwired: 5 in, 2 out]
        n332 = call <vilib>:"Add State(s) to Queue__JKI_lib_State_Machine.vi"("State(s) in (\"\")"=w1669) -> ("States Out"=w1668:string)  [unwired: 14 in]
      }
      frame "Database:GetSampleInfoFromDataBase" {
        # "Your code here.\n(You can make a copy of, or modify, this frame)"
        n333 = call "SelectData.vi"("SQL query"="select *from t_sample_info;") -> ("recordset data"=w1681:variant[][])  [unwired: 7 in, 1 out]
        n334 = disable-structure shown="禁用" {
          frame Disabled {
            n335 = call "SelectData.vi"("SQL query"="select *from t_sample_info;") -> ("recordset data"=w1690:variant[][])  [unwired: 7 in, 1 out]
            n336 = call "ReadDataFromDatabase.vi"("长度"=10, "index"=0, "recordset data"=w1690) -> ()  [unwired: 7 in, 2 out]
          }
          frame Enabled {
          }
        }
        n337 = call "ReadDataFromDatabase.vi"("长度"=10, "index"=0, "recordset data"=w1681) -> ("所有记录"=w1678:string[][])  [unwired: 7 in, 1 out]
        n338 = Array Subset(array=w1678, index (col)=1 ("禁用的索引 (列)")) -> (w1683:string[][])  [unwired: 3 in]
        n339 = property on="数据监测界面" class="MCListbox (严格)"("ItemNames"=w1683) -> ()  [unwired: 2 in, 2 out]
        n340 = call <vilib>:"Add State(s) to Queue__JKI_lib_State_Machine.vi"("State(s) in (\"\")"=w1687) -> ("States Out"=w1686:string)  [unwired: 14 in]
      }
      frame "Database:InsertSampleInfo" {
        # "Your code here.\n(You can make a copy of, or modify, this frame)"
        n341 = case shown="\"ManualSample\"" w1692 {
          tunnel: w1696 -> [w1700 w1702]
          tunnel: [w1699 w1701] -> w1695
          frame "TimeSample", Default {
            n342 = Unbundle By Name(w1700) -> ("TimeSampleInfo"=w1699:T24)
          }
          frame "ManualSample" {
            n343 = Unbundle By Name(w1702) -> ("ManualSampleInfo"=w1701:T29)
          }
        }
        n344 = call "InsertDataSampleInfo.vi"("error in"=w1694, "检测电极"=w1695) -> ("error out"=w1693:errorcluster)  [unwired: 9 in]
        n345 = call <vilib>:"Add State(s) to Queue__JKI_lib_State_Machine.vi"("State(s) in (\"\")"=w1698) -> ("States Out"=w1697:string)  [unwired: 14 in]
      }
      frame "---------Sample---------" {
        # "Your code here.\n(You can make a copy of, or modify, this frame)"
        n346 = call <vilib>:"Add State(s) to Queue__JKI_lib_State_Machine.vi"("State(s) in (\"\")"=w1706) -> ("States Out"=w1705:string)  [unwired: 14 in]
      }
      frame "Sample:LoadSampleSetInfo" {
        # "此状态只运行一次"
        # "Your code here.\n(You can make a copy of, or modify, this frame)"
        n347 = call "SelectData.vi"("SQL query"="select * from t_sample_set;") -> ("recordset data"=w1710:variant[][])  [unwired: 7 in, 1 out]
        n348 = call "ReadDataFromDatabase.vi"("长度"=9, "index"=0, "recordset data"=w1710) -> ("所有记录"=w1707:string[][])  [unwired: 7 in, 1 out]
        n349 = local write "定时采样信息D"(w1707) -> ()
        n350 = call <vilib>:"Add State(s) to Queue__JKI_lib_State_Machine.vi"("State(s) in (\"\")"=w1715) -> ("States Out"=w1714:string)  [unwired: 14 in]
      }
      frame "Sample:StartTimeSample" {
        # "Your code here.\n(You can make a copy of, or modify, this frame)"
        n351 = call-poly "Enqueue Message.vi"("error in (no error)"=w1717, "Message"="Start", "Message Queue"=w1718) -> ()  [unwired: 7 in, 2 out]
        n352 = call <vilib>:"Add State(s) to Queue__JKI_lib_State_Machine.vi"("State(s) in (\"\")"=w1722) -> ("States Out"=w1721:string)  [unwired: 14 in]
      }
      frame "Sample:StopSample" {
        # "Your code here.\n(You can make a copy of, or modify, this frame)"
        n353 = call-poly "Enqueue Message.vi"("error in (no error)"=w1723, "Message"="StopSample", "Message Queue"=w1725) -> ()  [unwired: 7 in, 2 out]
        n354 = call <vilib>:"Add State(s) to Queue__JKI_lib_State_Machine.vi"("State(s) in (\"\")"=w1729) -> ("States Out"=w1728:string)  [unwired: 14 in]
      }
      frame "-----------TimeSample----------" {
        # "Your code here.\n(You can make a copy of, or modify, this frame)"
        n355 = call <vilib>:"Add State(s) to Queue__JKI_lib_State_Machine.vi"("State(s) in (\"\")"=w1733) -> ("States Out"=w1732:string)  [unwired: 14 in]
      }
      frame "TimeSample:GetSampleInfo" {
        w1737 = T24 {"", "采样时间"="", "检测区域"="", "供电位置"="", "采样方式"="", "", "", "电源电压"="", "电源电流"="", "备注"=""}  # TimeSampleInfo
        w1749 = ""
        # "预判"
        # "Your code here.\n(定时检测信息)"
        n356 = Unbundle By Name(w1744) -> ("定时采样信息.检测区域"=w1736:string, "定时采样信息.时"=w1739:u16, "定时采样信息.分钟"=w1738:u16, "定时采样信息.供电位置"=w1735:string, "定时采样信息.备注"=w1747:string, "时分"=w1734:string)  [unwired: 2 out]
        n357 = Format Date/Time String(time format string (%c)="%Y-%m-%d" ("时间格式字符串(%c)")) -> (date/time string=w1742:string)  [unwired: 2 in]
        n358 = Number To Decimal String(number=w1739) -> ()  [unwired: 1 in, 1 out]
        n359 = Number To Decimal String ("数值至十进制数字符串转换")(number=w1738, width (-)=i16 2 ("宽度(-)")) -> ()  [unwired: 1 out]
        n360 = call "DigitToStr.vi"("时/分"=w1739) -> ()  [unwired: 10 in, 1 out]
        n361 = call "DigitToStr.vi"("时/分"=w1738) -> ()  [unwired: 10 in, 1 out]
        n362 = call <vilib>:"Space Constant.vi"() -> ("String"=w1741:string)
        n363 = Concatenate Strings(w1742, w1741, w1734) -> (w1751:string)
        n364 = Bundle(cluster=w1737, "0", "采样时间"=w1751, "检测区域"=w1736, "供电位置"=w1735, "采样方式"="定时检测", w1749, w1749, "电源电压"="", "电源电流"="", "备注"=w1747) -> (w1745:T24)
        n365 = Bundle By Name(cluster=w1744, "TimeSampleInfo"=w1745) -> (w1743:T21)
        n366 = call <vilib>:"Add State(s) to Queue__JKI_lib_State_Machine.vi"("State(s) in (\"\")"=w1756) -> ("States Out"=w1755:string)  [unwired: 14 in]
      }
      frame "TimeSample:TimeSampleDialog" {
        # "Your code here.\n(定时采样对话框)"
        n367 = call "TimeSampleDlg.vi"() -> ("定时采样信息"=→"定时采样信息D":string[][], "是否采样"=→"是否采样":bool)  [unwired: 8 in, 2 out]
        n368 = disable-structure shown="禁用" {
          disable-tunnel: w1763 -> [w1769 _]
          disable-tunnel: [w1768 _] -> w1762
          disable-tunnel: [w1767 _] -> w1757
          disable-tunnel: [w1766 _] -> _
          frame Disabled {
            n369 = call "TimeTestingDialog.vi"("错误输入"=w1769) -> ("错误输出"=w1768:errorcluster, "OKCancel"=w1766:bool, "定时采样设置输出"=w1767:T27)  [unwired: 8 in]
          }
          frame Enabled {
          }
        }
        n370 = Bundle By Name(cluster=w1761, "定时采样信息"=w1757) -> (w1760:T21)
        n371 = call <vilib>:"Add State(s) to Queue__JKI_lib_State_Machine.vi"("State(s) in (\"\")"=w1765) -> ("States Out"=w1764:string)  [unwired: 14 in]
      }
      frame "-----------ManualSample---------" {
        n372 = call <vilib>:"Add State(s) to Queue__JKI_lib_State_Machine.vi"("State(s) in (\"\")"=w1773) -> ("States Out"=w1772:string)  [unwired: 14 in]
      }
      frame "ManualSample:GetSampleInfo" {
        w1782 = ""
        n373 = Unbundle By Name(w1775) -> ("手动采样信息.选定检测区域"=w1785:string, "手动采样信息.采样位置"=w1784:string, "手动采样信息.电源电压"=w1781:string, "手动采样信息.电源电流"=w1780:string, "手动采样信息.检测方式"=w1783:string, "手动采样信息.备注"=w1779:string)  [unwired: 1 out]
        n374 = Format Date/Time String(time format string (%c)="%Y-%m-%d %H:%M" ("时间格式字符串(%c)")) -> (date/time string=w1786:string)  [unwired: 2 in]
        n375 = Bundle("0", "date/time string"=w1786, "选定检测区域"=w1785, "采样位置"=w1784, "检测方式"=w1783, w1782, w1782, "电源电压"=w1781, "电源电流"=w1780, "备注"=w1779) -> (w1776:T29)  [unwired: 1 in]
        n376 = Bundle By Name(cluster=w1775, "ManualSampleInfo"=w1776) -> (w1774:T21)
        n377 = call <vilib>:"Add State(s) to Queue__JKI_lib_State_Machine.vi"("State(s) in (\"\")"=w1789) -> ("States Out"=w1788:string)  [unwired: 14 in]
      }
      frame "ManualSample:ManualTestingDialog" {
        (unwired) "ManualSample:GetSampleInfo\nDatabase:InsertSampleInfo>>ManualSample\nHW:Acquire\nDatabase:InsertSampleData\nHW:ConfigAndAcquire01\nDatabase:InsertSampleData\nDatabase:GetSampleInfoFromDataBase"
        (unwired) "ManualSample:GetSampleInfo\nDatabase:InsertSampleInfo>>ManualSample\nHW:PowerOutput\nHW:OpenPowerElec>>ManualSample\nHW:Acquire\nHW:ClosePowerOutput\nHW:ClosePowerElec>>ManualSample\nDatabase:InsertSampleVandA>>ManualSample\nDatabase:InsertSampleData>>ManualSample\nDatabase:GetSampleInfoFromDataBase\nSample:StopSample"
        # "两个模块事件结构"
        # "这是获取手动采样对话框，提取一些信息"
        # "Database:InsertSampleInfo>>ManualSample"
        # "Your code here.\n(You can make a copy of, or modify, this frame)"
        n378 = call "ManualTestingDialog.vi"("error in"=w1801) -> ("error out"=w1800:errorcluster, "是否采样"=w1794:bool, "采样信息"=w1795:T30, "设置电源电压05V"=w1791:string)  [unwired: 5 in, 2 out]
        "电压05V" <- w1791
        n379 = Bundle By Name(cluster=w1797, "手动采样信息"=w1795, "手动采样到AO电压"=w1791) -> (w1796:T21)
        n380 = case shown="真" w1794 {
          tunnel: w1792 -> [_ w1805]
          tunnel: w1793 -> [_ w1804]
          frame False {
          }
          frame True {
            n381 = call-poly "Enqueue Message.vi"("error in (no error)"=w1804, "Message"="StartSample", "Message Queue"=w1805) -> ()  [unwired: 7 in, 2 out]
          }
        }
        n382 = Select(t="ManualSample:GetSampleInfo\nDatabase:InsertSampleInfo>>ManualSample\nHW:PowerOutput\nHW:OpenPowerElec>>ManualSample\nHW:Acquire\nHW:GetVandAvalue>>ManualSample\nHW:ClosePowerOutput\nHW:ClosePowerElec>>ManualSample\nDatabase:InsertSampleVandA>>ManualSample\nDatabase:InsertSampleData>>ManualSample\nDatabase:GetSampleInfoFromDataBase\nSample:StopSample\njiemian:GengxinJiemian", s=w1794, f="Database:GetSampleInfoFromDataBase") -> (s? t:f=w1798:string)
        n383 = call <vilib>:"Add State(s) to Queue__JKI_lib_State_Machine.vi"("State(s) in Front (\"\")"=w1798, "State(s) in (\"\")"=w1803) -> ("States Out"=w1802:string)  [unwired: 13 in]
      }
      frame "-------------Config-------------" {
        # "Your code here.\n(You can make a copy of, or modify, this frame)"
        n384 = call <vilib>:"Add State(s) to Queue__JKI_lib_State_Machine.vi"("State(s) in (\"\")"=w1810) -> ("States Out"=w1809:string)  [unwired: 14 in]
      }
      frame "Congfig:helpDlg" {
        # "Your code here.\n(You can make a copy of, or modify, this frame)"
        n385 = call "HelpDlg.vi"() -> ()  [unwired: 12 in]
        n386 = call <vilib>:"Add State(s) to Queue__JKI_lib_State_Machine.vi"("State(s) in (\"\")"=w1814) -> ("States Out"=w1813:string)  [unwired: 14 in]
      }
      frame "Config:PowerControlDlg" {
        # "Your code here.\n(电源控制对话框)"
        n387 = call "PowerControlDlg.vi"("error out"=w1822) -> ("error out"=w1821:errorcluster, "NY"=w1816:bool, "电源电压(V)out"=w1818:string, "电压系数out"=w1817:string)  [unwired: 6 in, 1 out]
        "NY" <- w1816
        n388 = case shown="真" w1816 {
          tunnel: w1816 -> [_ w1832]
          tunnel: w1820 -> [w1826 w1831]
          tunnel: [w1826 w1830] -> w1819
          tunnel: w1818 -> [_ w1829]
          tunnel: w1817 -> [_ w1828]
          tunnel: ["" "HW:PowerOutput\nHW:GetVandA\nHW:ClosePowerOutput"] -> w1815
          frame False {
          }
          frame True {
            n389 = Bundle By Name(cluster=w1831, "PowTN"=w1832, "电压系数"=w1828, "基准电压"=w1829) -> (w1830:T21)
          }
        }
        n390 = call <vilib>:"Add State(s) to Queue__JKI_lib_State_Machine.vi"("State(s) in Front (\"\")"=w1815, "State(s) in (\"\")"=w1824) -> ("States Out"=w1823:string)  [unwired: 13 in]
      }
      frame "Config:SampleInfoManage" {
        # "Your code here.\n(You can make a copy of, or modify, this frame)"
        n391 = call "DetecRecodManDlg.vi"("error in"=w1834) -> ("error out"=w1833:errorcluster)  [unwired: 10 in]
        n392 = call <vilib>:"Add State(s) to Queue__JKI_lib_State_Machine.vi"("State(s) in (\"\")"=w1837) -> ("States Out"=w1836:string)  [unwired: 14 in]
      }
      frame "Config:ChaxuConfigInfo" {
        # "Your code here.\n(You can make a copy of, or modify, this frame)"
        n393 = call "ChaxuConfigDlg.vi"("error in"=w1839) -> ("error out"=w1838:errorcluster)  [unwired: 10 in]
        n394 = call <vilib>:"Add State(s) to Queue__JKI_lib_State_Machine.vi"("State(s) in (\"\")"=w1842) -> ("States Out"=w1841:string)  [unwired: 14 in]
      }
      frame "Config:Launch DscDistDialog" {
        # "Your code here.\n(You can make a copy of, or modify, this frame)"
        n395 = call "Dsc_BoardElecMan.vi"("error in"=w1844) -> ("error out"=w1843:errorcluster)  [unwired: 10 in]
        n396 = call <vilib>:"Add State(s) to Queue__JKI_lib_State_Machine.vi"("State(s) in (\"\")"=w1847) -> ("States Out"=w1846:string)  [unwired: 14 in]
      }
      frame "Config:Launch DSCManDialog" {
        # "Your code here.\n(You can make a copy of, or modify, this frame)"
        n397 = call "Dsc_Board_Man_Dlg.vi"("error in"=w1849) -> ("error out"=w1848:errorcluster)  [unwired: 10 in]
        n398 = call <vilib>:"Add State(s) to Queue__JKI_lib_State_Machine.vi"("State(s) in (\"\")"=w1852) -> ("States Out"=w1851:string)  [unwired: 14 in]
      }
      frame "Config:Launch Power_configDialog" {
        # "Your code here.\n(You can make a copy of, or modify, this frame)"
        n399 = call "PowerElectrodesDlg.vi"("error in"=w1854) -> ("error out"=w1853:errorcluster)  [unwired: 10 in]
        n400 = call <vilib>:"Add State(s) to Queue__JKI_lib_State_Machine.vi"("State(s) in (\"\")"=w1857) -> ("States Out"=w1856:string)  [unwired: 14 in]
      }
      frame "Config:Launch Dete_configDialog" {
        # "Your code here.\n(You can make a copy of, or modify, this frame)"
        n401 = call "DetectElectroMan.vi"("error in (no error)"=w1859) -> ("error out"=w1858:errorcluster)  [unwired: 10 in]
        n402 = call <vilib>:"Add State(s) to Queue__JKI_lib_State_Machine.vi"("State(s) in (\"\")"=w1862) -> ("States Out"=w1861:string)  [unwired: 14 in]
      }
      frame "Config:Launch Area_configDialog" {
        # "Your code here.\n(You can make a copy of, or modify, this frame)"
        n403 = call "area_setting.vi"("error in (no error)"=w1864) -> ("error out (no error) 2"=w1863:errorcluster)  [unwired: 10 in]
        n404 = call <vilib>:"Add State(s) to Queue__JKI_lib_State_Machine.vi"("State(s) in (\"\")"=w1867) -> ("States Out"=w1866:string)  [unwired: 14 in]
      }
      frame "----------HW---------" {
        # "Your code here.\n(You can make a copy of, or modify, this frame)"
        n405 = call <vilib>:"Add State(s) to Queue__JKI_lib_State_Machine.vi"("State(s) in (\"\")"=w1871) -> ("States Out"=w1870:string)  [unwired: 14 in]
      }
      frame "HW:ClosePowerElec" {
        # "Your code here.\n(You can make a copy of, or modify, this frame)"
        n406 = case shown="\"ManualSample\"" w1875 {
          tunnel: w1874 -> [w1912 w1915]
          tunnel: [w1911 w1914] -> w1877
          tunnel: [w1910 w1913] -> w1876
          frame "TimeSample", Default {
            n407 = Unbundle By Name(w1912) -> ("TimeSampleInfo.供电位置"=w1911:string, "TimeSampleInfo.检测区域"=w1910:string)
          }
          frame "ManualSample" {
            n408 = Unbundle By Name(w1915) -> ("ManualSampleInfo.采样位置"=w1914:string, "ManualSampleInfo.选定检测区域"=w1913:string)
          }
        }
        n409 = case shown="\"1区\", 默认" w1876 {
          tunnel: w1877 -> [w1882 w1900 _]
          tunnel: w1873 -> [w1880 w1896 w1909]
          tunnel: [w1881 w1895 w1909] -> w1872
          frame "1区", Default {
            n410 = String Subset(string=w1882, offset (0)=0 ("偏移量(0)"), length (rest)=6 ("长度（剩余）")) -> (substring=w1883:string)
            n411 = case shown="\"上层膜\"" w1883 {
              tunnel: [w1886 w1891] -> w1881
              tunnel: w1880 -> [w1888 w1890]
              frame "下层膜", Default {
                n412 = call "PowerElecControl.vi"("error in"=w1888, "设置通道开关"=bool[] [FALSE, FALSE, FALSE, FALSE], "线"=tag "Dev9/port0/line0:3") -> ("error out"=w1886:errorcluster)  [unwired: 8 in]
              }
              frame "上层膜" {
                n413 = call "PowerElecControl.vi"("error in"=w1890, "设置通道开关"=bool[] [FALSE, FALSE, FALSE, FALSE], "线"=tag "Dev9/port0/line0:3") -> ("error out"=w1891:errorcluster)  [unwired: 8 in]
              }
            }
          }
          frame "2区" {
            n414 = Wait (ms)(milliseconds to wait=u32 1000 ("等待时间（毫秒）")) -> ()  [unwired: 1 out]
            n415 = String Subset(string=w1900, offset (0)=0 ("偏移量(0)"), length (rest)=6 ("长度（剩余）")) -> (substring=w1897:string)
            n416 = case shown="\"下层膜\"" w1897 {
              tunnel: w1896 -> [w1902 w1907]
              tunnel: [w1901 w1908] -> w1895
              frame "下层膜" {
                n417 = call "PowerElecControl.vi"("error in"=w1902, "设置通道开关"=bool[] [FALSE, FALSE, FALSE, FALSE], "线"=tag "Dev10/port0/line0:3") -> ("error out"=w1901:errorcluster)  [unwired: 8 in]
              }
              frame "上层膜", Default {
                n418 = call "PowerElecControl.vi"("error in"=w1907, "设置通道开关"=bool[] [FALSE, FALSE, FALSE, FALSE], "线"=tag "Dev10/port0/line0:3") -> ("error out"=w1908:errorcluster)  [unwired: 8 in]
              }
            }
          }
          frame "所有区" {
          }
        }
        n419 = call <vilib>:"Add State(s) to Queue__JKI_lib_State_Machine.vi"("State(s) in (\"\")"=w1879) -> ("States Out"=w1878:string)  [unwired: 14 in]
      }
      frame "HW:PowerOutput" {
        # "获取AO与电源的线性关系"
        # "Your code here.\n(You can make a copy of, or modify, this frame)"
        n420 = flat-sequence {
          tunnel: w1921 -> [w1927]
          tunnel: w1920 -> [w1928]
          tunnel: [w1928] -> w1919
          tunnel: [w1927] -> w1917
          tunnel: w1923 -> [w1933]
          tunnel: [w1932] -> w1922
          tunnel: w1919 -> [w1931]
          tunnel: [w1931] -> w1918
          tunnel: w1917 -> [w1930]
          tunnel: [w1930] -> w1916
          tunnel: w1918 -> [w1939]
          tunnel: w1916 -> [w1938]
          frame #0 {
          }
          frame #1 {
            n421 = call "GetVandBeishu.vi"() -> ("电压倍数"=→"电压倍数":string, "电压频率"=w1934:string, "输出电压值"=→"输出电压值":string)  [unwired: 9 in]
            "电压频率" <- w1934
            n422 = Bundle By Name(cluster=w1933, "power_f"=w1934) -> (w1932:T21)
            n423 = Wait (ms)(milliseconds to wait=1000) -> ()  [unwired: 1 out]
          }
          frame #2 {
            n424 = call-poly "Enqueue Message.vi"("error in (no error)"=w1938, "Message"="Start", "Message Queue"=w1939) -> ()  [unwired: 7 in, 2 out]
            n425 = Wait (ms)(milliseconds to wait=1000) -> ()  [unwired: 1 out]
          }
        }
        n426 = call <vilib>:"Add State(s) to Queue__JKI_lib_State_Machine.vi"("State(s) in (\"\")"=w1926) -> ("States Out"=w1925:string)  [unwired: 14 in]
      }
      frame "HW:ClosePowerOutput" {
        # "获取AO与电源的线性关系"
        # "Your code here.\n(You can make a copy of, or modify, this frame)"
        n427 = disable-structure shown="禁用" {
          frame Disabled {
            n428 = call "GetVandBeishu.vi"() -> ("电压频率"=w1950:string)  [unwired: 9 in, 2 out]
            n429 = Bundle By Name("power_f"=w1950) -> ()  [unwired: 1 in, 1 out]
          }
          frame Enabled {
          }
        }
        n430 = Wait (ms)(milliseconds to wait=1000 ("延时关闭继电器")) -> ()  [unwired: 1 out]
        n431 = call-poly "Enqueue Message.vi"("error in (no error)"=w1944, "Message"="Stop", "Message Queue"=w1946) -> ()  [unwired: 7 in, 2 out]
        n432 = local write "输出电压值"("0") -> ()
        n433 = call <vilib>:"Add State(s) to Queue__JKI_lib_State_Machine.vi"("State(s) in (\"\")"=w1949) -> ("States Out"=w1948:string)  [unwired: 14 in]
      }
      frame "HW:GetVandA" {
        # "select power_v from t_power_v  where power_v_id=1;"
        # "Your code here.\n这个事件结构是获取电压和电流值\n差分模式\n第0路采集电压\n第1路采集电流"
        n434 = Unbundle By Name(w1952) -> ("power_f"=w1961:string, "基准电压"=w1958:string, "电压系数"=w1959:string)
        n435 = call "AcquireVandA.vi"("Hardware Configuration"=T16 {"Physical Channel"="Dev18/ai0", "Maximum Input"=10.0, "Minimum Input"=-10.0, "Sample Rate"=5000.0, "Number of Samples"=5000}) -> ("Graph Data"=w1964:waveform(dbl)[])  [unwired: 8 in, 1 out]
        n436 = Split Signals(w1964) -> (w1966:dynamicdata)  [unwired: 1 in]
        n437 = call "从动态数据转换"("Dynamic Data Type"=w1966) -> ("Array"=w1962:dbl[])  [unwired: 3 in]
        n438 = Decimal String To Number(string=w1961) -> (number=w1960:i32)  [unwired: 2 in, 1 out]
        n439 = Fract/Exp String To Number(string=w1958) -> (number=w1956:dbl)  [unwired: 3 in, 1 out]
        n440 = Fract/Exp String To Number(string=w1959) -> (number=w1954:dbl)  [unwired: 3 in, 1 out]
        n441 = call "1chFFT.vi"("Array"=w1962, "频率"=w1960) -> ("幅度值"=w1957:dbl)  [unwired: 2 in, 1 out]
        n442 = Divide(x=w1957, y=w1956) -> (x/y=w1955:dbl)
        n443 = Divide(x=w1955, y=w1954) -> (x/y=w1953:dbl)
        n444 = Unbundle By Name(w1952) -> ("PowTN"=w1963:bool)
        n445 = case shown="真" w1963 {
          tunnel: w1957 -> [_ w1985]
          tunnel: w1953 -> [_ w1979]
          tunnel: w1952 -> [w1970 w1973]
          tunnel: [w1970 w1972] -> w1951
          frame False {
          }
          frame True {
            n446 = Number To Fractional String(number=w1979) -> (F-format string=w1971:string)  [unwired: 3 in]
            n447 = Number To Fractional String(number=w1985, precision (6)=i16 3 ("宽度(-)")) -> (F-format string=w1977:string)  [unwired: 2 in]
            n448 = Concatenate Strings("电压:", w1977, "\r", "倍数：", w1971) -> (w1983:string)
            n449 = Concatenate Strings(w1983, "\r") -> (w1981:string)
            n450 = Bundle By Name(cluster=w1973, "电压倍数"=w1971) -> (w1972:T21)
            n451 = call "显示对话框信息"("Message"=w1981) -> ()  [unwired: 9 in, 2 out]
            n452 = Format Into String(format string="update t_power_v set power_beishu='%s',\npower_shiji_v='%s' where power_v_id=1;", w1971, w1977) -> (resulting string=w1976:string)  [unwired: 2 in, 1 out]
            n453 = call "updateData.vi"("SQL query"=w1976) -> ()  [unwired: 10 in, 1 out]
          }
        }
        n454 = call <vilib>:"Add State(s) to Queue__JKI_lib_State_Machine.vi"("State(s) in (\"\")"=w1969) -> ("States Out"=w1968:string)  [unwired: 14 in]
      }
      frame "HW:GetVandAvalue" {
        (unwired) 1.0
        # "默认频率为1Hz"
        # "每次采样完成获取电压和电流\n这个事件结构是获取电压和电流值\n差分模式\n第0路采集电压\n第1路采集电流"
        n455 = Unbundle By Name(w1995) -> ("power_f"=w1999:string)
        n456 = call "AcquireVandA.vi"("Hardware Configuration"=T16 {"Physical Channel"="Dev18/ai0:7", "Maximum Input"=10.0, "Minimum Input"=-10.0, "Sample Rate"=5000.0, "Number of Samples"=5000}) -> ("Graph Data"=w1997:waveform(dbl)[])  [unwired: 8 in, 1 out]
        n457 = Decimal String To Number(string=w1999) -> (number=w1991:i32)  [unwired: 2 in, 1 out]
        "Hz" <- w1991
        n458 = Split Signals(w1997) -> (w2002:dynamicdata, w1993:dynamicdata)  [unwired: 2 in]
        n459 = call "从动态数据转换3"("Dynamic Data Type"=w1993) -> ("Array"=w1992:dbl[])  [unwired: 3 in]
        n460 = call "从动态数据转换2"("Dynamic Data Type"=w2002) -> ("Array"=w2001:dbl[])  [unwired: 3 in]
        n461 = call "1chFFT.vi"("Array"=w2001, "频率"=w1991) -> ("幅度值"=w2000:dbl)  [unwired: 2 in, 1 out]
        n462 = call "1chFFT.vi"("Array"=w1992, "频率"=w1991) -> ("幅度值"=w1990:dbl)  [unwired: 2 in, 1 out]
        n463 = Divide(x=w1990, y=5) -> (x/y=w1988:dbl)
        n464 = Number To Fractional String(number=w1988, precision (6)=i16 4 ("宽度(-)")) -> (F-format string=w1994:string)  [unwired: 2 in]
        "电流" <- w1994
        n465 = Number To Fractional String(number=w2000, precision (6)=i16 4 ("宽度(-)")) -> (F-format string=w1996:string)  [unwired: 2 in]
        "电压回来" <- w1996
        n466 = Bundle By Name(cluster=w1995, "回来电压"=w1996, "回来电流"=w1994) -> (w1986:T21)
        n467 = case shown="\"ManualSample\"" w2003 {
          tunnel: w1986 -> [w2012 w2016]
          tunnel: [w2011 w2015] -> w1987
          tunnel: w1996 -> [w2010 w2014]
          tunnel: w1994 -> [w2009 w2013]
          frame "TimeSample", Default {
            n468 = Bundle By Name(cluster=w2012, "TimeSampleInfo.电源电压"=w2010, "TimeSampleInfo.电源电流"=w2009) -> (w2011:T21)
          }
          frame "ManualSample" {
            n469 = Bundle By Name(cluster=w2016, "ManualSampleInfo.电源电压"=w2014, "ManualSampleInfo.电源电流"=w2013) -> (w2015:T21)
          }
        }
        n470 = call <vilib>:"Add State(s) to Queue__JKI_lib_State_Machine.vi"("State(s) in (\"\")"=w2008) -> ("States Out"=w2007:string)  [unwired: 14 in]
      }
      frame "HW:OpenPowerElec" {
        # "在这事件帧下，放入控制上层膜和下层膜的供电电极\n即控制继电器"
        n471 = case shown="\"ManualSample\"" w2022 {
          tunnel: w2021 -> [w2065 w2068]
          tunnel: [w2064 w2067] -> w2020
          tunnel: [w2063 w2066] -> w2017
          frame "TimeSample", Default {
            n472 = Unbundle By Name(w2065) -> ("TimeSampleInfo.供电位置"=w2064:string, "TimeSampleInfo.检测区域"=w2063:string)
          }
          frame "ManualSample" {
            n473 = Unbundle By Name(w2068) -> ("ManualSampleInfo.采样位置"=w2067:string, "ManualSampleInfo.选定检测区域"=w2066:string)
          }
        }
        n474 = case shown="\"1区\", 默认" w2017 {
          tunnel: [w2030 w2044 "所有分区" ("字符串 2")] -> w2023
          tunnel: w2020 -> [w2029 w2050 _]
          tunnel: w2019 -> [w2027 w2046 w2062]
          tunnel: [w2028 w2045 w2062] -> w2018
          frame "1区", Default {
            n475 = String Subset(string=w2029, offset (0)=0 ("偏移量(0)"), length (rest)=6 ("长度（剩余）")) -> (substring=w2031:string)
            n476 = Wait (ms)(milliseconds to wait=1000) -> ()  [unwired: 1 out]
            n477 = case shown="\"下层膜\", 默认" w2031 {
              tunnel: ["下层膜" "上层膜"] -> w2030
              tunnel: [w2034 w2042] -> w2028
              tunnel: w2027 -> [w2035 w2041]
              frame "下层膜", Default {
                n478 = call "PowerElecControl.vi"("error in"=w2035, "设置通道开关"=bool[] [FALSE, TRUE, TRUE, FALSE], "线"=tag "Dev9/port0/line0:3") -> ("error out"=w2034:errorcluster)  [unwired: 8 in]
              }
              frame "上层膜" {
                n479 = call "PowerElecControl.vi"("error in"=w2041, "设置通道开关"=bool[] [TRUE, TRUE, FALSE, FALSE], "线"=tag "Dev9/port0/line0:3") -> ("error out"=w2042:errorcluster)  [unwired: 8 in]
              }
            }
          }
          frame "2区" {
            n480 = String Subset(string=w2050, offset (0)=0 ("偏移量(0)"), length (rest)=6 ("长度（剩余）")) -> (substring=w2047:string)
            n481 = case shown="\"下层膜\"" w2047 {
              tunnel: w2046 -> [w2053 w2059]
              tunnel: [w2052 w2060] -> w2045
              tunnel: ["下层膜" "上层膜"] -> w2044
              frame "下层膜" {
                n482 = call "PowerElecControl.vi"("error in"=w2053, "设置通道开关"=bool[] [FALSE, TRUE, TRUE, FALSE], "线"=tag "Dev10/port0/line0:3") -> ("error out"=w2052:errorcluster)  [unwired: 8 in]
              }
              frame "上层膜", Default {
                n483 = call "PowerElecControl.vi"("error in"=w2059, "设置通道开关"=bool[] [TRUE, TRUE, FALSE, TRUE], "线"=tag "Dev10/port0/line0:3") -> ("error out"=w2060:errorcluster)  [unwired: 8 in]
              }
            }
          }
          frame "所有区" {
          }
        }
        "字符串" <- w2023
        n484 = call <vilib>:"Add State(s) to Queue__JKI_lib_State_Machine.vi"("State(s) in (\"\")"=w2025) -> ("States Out"=w2024:string)  [unwired: 14 in]
      }
      frame "HW:Acquire" {
        n485 = call "Acquire Data from Hardware.vi"("Hardware Configuration"=T16 {"Physical Channel"="Dev15/ai0:31", "Maximum Input"=10.0, "Minimum Input"=-10.0, "Sample Rate"=5000.0, "Number of Samples"=5000}) -> ("Graph Data"=w2086:waveform(dbl)[])  [unwired: 8 in, 1 out]
        n486 = call "Acquire Data from Hardware.vi"("Hardware Configuration"=T16 {"Physical Channel"="Dev1/ai0:31", "Maximum Input"=10.0, "Minimum Input"=-10.0, "Sample Rate"=5000.0, "Number of Samples"=5000}) -> ("Graph Data"=w2125:waveform(dbl)[])  [unwired: 8 in, 1 out]
        n487 = call "Acquire Data from Hardware.vi"("Hardware Configuration"=T16 {"Physical Channel"="Dev2/ai0:31", "Maximum Input"=10.0, "Minimum Input"=-10.0, "Sample Rate"=5000.0, "Number of Samples"=5000}) -> ("Graph Data"=w2120:waveform(dbl)[])  [unwired: 8 in, 1 out]
        n488 = call "Acquire Data from Hardware.vi"("Hardware Configuration"=T16 {"Physical Channel"="Dev3/ai0:31", "Maximum Input"=10.0, "Minimum Input"=-10.0, "Sample Rate"=5000.0, "Number of Samples"=5000}) -> ("Graph Data"=w2116:waveform(dbl)[])  [unwired: 8 in, 1 out]
        n489 = call "Acquire Data from Hardware.vi"("Hardware Configuration"=T16 {"Physical Channel"="Dev4/ai0:31", "Maximum Input"=10.0, "Minimum Input"=-10.0, "Sample Rate"=5000.0, "Number of Samples"=5000}) -> ("Graph Data"=w2113:waveform(dbl)[])  [unwired: 8 in, 1 out]
        n490 = call "Acquire Data from Hardware.vi"("Hardware Configuration"=T16 {"Physical Channel"="Dev5/ai0:31", "Maximum Input"=10.0, "Minimum Input"=-10.0, "Sample Rate"=5000.0, "Number of Samples"=5000}) -> ("Graph Data"=w2110:waveform(dbl)[])  [unwired: 8 in, 1 out]
        n491 = call "Acquire Data from Hardware.vi"("Hardware Configuration"=T16 {"Physical Channel"="Dev6/ai0:31", "Maximum Input"=10.0, "Minimum Input"=-10.0, "Sample Rate"=5000.0, "Number of Samples"=5000}) -> ("Graph Data"=w2107:waveform(dbl)[])  [unwired: 8 in, 1 out]
        n492 = call "Acquire Data from Hardware.vi"("Hardware Configuration"=T16 {"Physical Channel"="Dev7/ai0:31", "Maximum Input"=10.0, "Minimum Input"=-10.0, "Sample Rate"=5000.0, "Number of Samples"=5000}) -> ("Graph Data"=w2104:waveform(dbl)[])  [unwired: 8 in, 1 out]
        n493 = call "Acquire Data from Hardware.vi"("Hardware Configuration"=T16 {"Physical Channel"="Dev8/ai0:31", "Maximum Input"=10.0, "Minimum Input"=-10.0, "Sample Rate"=5000.0, "Number of Samples"=5000}) -> ("Graph Data"=w2101:waveform(dbl)[])  [unwired: 8 in, 1 out]
        n494 = call "Acquire Data from Hardware.vi"("Hardware Configuration"=T16 {"Physical Channel"="Dev11/ai0:31", "Maximum Input"=10.0, "Minimum Input"=-10.0, "Sample Rate"=5000.0, "Number of Samples"=5000}) -> ("Graph Data"=w2098:waveform(dbl)[])  [unwired: 8 in, 1 out]
        n495 = call "Acquire Data from Hardware.vi"("Hardware Configuration"=T16 {"Physical Channel"="Dev12/ai0:31", "Maximum Input"=10.0, "Minimum Input"=-10.0, "Sample Rate"=5000.0, "Number of Samples"=5000}) -> ("Graph Data"=w2095:waveform(dbl)[])  [unwired: 8 in, 1 out]
        n496 = call "Acquire Data from Hardware.vi"("Hardware Configuration"=T16 {"Physical Channel"="Dev13/ai0:31", "Maximum Input"=10.0, "Minimum Input"=-10.0, "Sample Rate"=5000.0, "Number of Samples"=5000}) -> ("Graph Data"=w2092:waveform(dbl)[])  [unwired: 8 in, 1 out]
        n497 = call "Acquire Data from Hardware.vi"("Hardware Configuration"=T16 {"Physical Channel"="Dev14/ai0:31", "Maximum Input"=10.0, "Minimum Input"=-10.0, "Sample Rate"=5000.0, "Number of Samples"=5000}) -> ("Graph Data"=w2089:waveform(dbl)[])  [unwired: 8 in, 1 out]
        n498 = call "ChSetting.vi"("频率"="频率", "dsc地址"="0", "AcquireData"=w2125) -> ("DexASData"=w2082:T32)  [unwired: 5 in, 3 out]
        n499 = call "ChSetting.vi"("频率"="频率", "dsc地址"="1", "AcquireData"=w2120) -> ("DexASData"=w2081:T32)  [unwired: 5 in, 3 out]
        n500 = call "ChSetting.vi"("频率"="频率", "dsc地址"="2", "AcquireData"=w2116) -> ("DexASData"=w2080:T32)  [unwired: 5 in, 3 out]
        n501 = call "ChSetting.vi"("频率"="频率", "dsc地址"="3", "AcquireData"=w2113) -> ("DexASData"=w2079:T32)  [unwired: 5 in, 3 out]
        n502 = call "ChSetting.vi"("频率"="频率", "dsc地址"="4", "AcquireData"=w2110) -> ("DexASData"=w2078:T32)  [unwired: 5 in, 3 out]
        n503 = call "ChSetting.vi"("频率"="频率", "dsc地址"="5", "AcquireData"=w2107) -> ("DexASData"=w2077:T32)  [unwired: 5 in, 3 out]
        n504 = call "ChSetting.vi"("频率"="频率", "dsc地址"="6", "AcquireData"=w2104) -> ("DexASData"=w2076:T32)  [unwired: 5 in, 3 out]
        n505 = call "ChSetting.vi"("频率"="频率", "dsc地址"="7", "AcquireData"=w2101) -> ("DexASData"=w2075:T32)  [unwired: 5 in, 3 out]
        n506 = call "ChSetting.vi"("频率"="频率", "dsc地址"="8", "AcquireData"=w2098) -> ("DexASData"=w2074:T32)  [unwired: 5 in, 3 out]
        n507 = call "ChSetting.vi"("频率"="频率", "dsc地址"="9", "AcquireData"=w2095) -> ("DexASData"=w2073:T32)  [unwired: 5 in, 3 out]
        n508 = call "ChSetting.vi"("频率"="频率", "dsc地址"="10", "AcquireData"=w2092) -> ("DexASData"=w2072:T32)  [unwired: 5 in, 3 out]
        n509 = call "ChSetting.vi"("频率"="频率", "dsc地址"="12", "AcquireData"=w2086) -> ("DexASData"=w2070:T32)  [unwired: 5 in, 3 out]
        n510 = call "ChSetting.vi"("频率"="频率", "dsc地址"="11", "AcquireData"=w2089) -> ("DexASData"=w2071:T32)  [unwired: 5 in, 3 out]
        n511 = Bundle By Name(cluster=T17 {"Dev1ASData"={"DevChSampData"=[], "dscAddress"=""}, "Dev2ASData"={"DevChSampData"=[], "dscAddress"=""}, "Dev3ASData"={"DevChSampData"=[], "dscAddress"=""}, "Dev4ASData"={"DevChSampData"=[], "dscAddress"=""}, "Dev5ASData"={"DevChSampData"=[], "dscAddress"=""}, "Dev6ASData"={"DevChSampData"=[], "dscAddress"=""}, "Dev7ASData"={"DevChSampData"=[], "dscAddress"=""}, "Dev8ASData"={"DevChSampData"=[], "dscAddress"=""}, "Dev9ASData"={"DevChSampData"=[], "dscAddress"=""}, "Dev10ASData"={"DevChSampData"=[], "dscAddress"=""}, "Dev11ASData"={"DevChSampData"=[], "dscAddress"=""}, "Dev12ASData"={"DevChSampData"=[], "dscAddress"=""}, "Dev13ASData"={"DevChSampData"=[], "dscAddress"=""}} ("DevNASSData"), "Dev1ASData"=w2082, "Dev2ASData"=w2081, "Dev3ASData"=w2080, "Dev4ASData"=w2079, "Dev5ASData"=w2078, "Dev6ASData"=w2077, "Dev7ASData"=w2076, "Dev8ASData"=w2075, "Dev9ASData"=w2074, "Dev10ASData"=w2073, "Dev11ASData"=w2072, "Dev12ASData"=w2071, "Dev13ASData"=w2070) -> (w2083:T17)
        n512 = Bundle By Name(cluster=w2122, "DevNASSData"=w2083) -> (w2126:T21)
        n513 = call <vilib>:"Add State(s) to Queue__JKI_lib_State_Machine.vi"("State(s) in (\"\")"=w2128) -> ("States Out"=w2127:string)  [unwired: 14 in]
      }
      frame "HW:ConfigAndAcquire01" {
        # "Your code here.\n(You can make a copy of, or modify, this frame)"
        n514 = call "Acquire Data from Hardware.vi"("Hardware Configuration"=T16 {"Physical Channel"="Dev2/ai0:31", "Maximum Input"=10.0, "Minimum Input"=-10.0, "Sample Rate"=1000.0, "Number of Samples"=100}) -> ("Graph Data"=w2134:waveform(dbl)[])  [unwired: 8 in, 1 out]
        n515 = call "ChSetting.vi"("dsc地址"="1", "AcquireData"=w2134) -> ("DevChSampData"=w2131:cluster{"通道编号":string, "Data":dbl}[], "DevChSampleData"=w2132:T28)  [unwired: 6 in, 2 out]
        n516 = Bundle By Name(cluster=w2130, "DevChSampleData"=w2132, "DevChSampData"=w2131) -> (w2129:T21)
        n517 = call <vilib>:"Add State(s) to Queue__JKI_lib_State_Machine.vi"("State(s) in (\"\")"=w2138) -> ("States Out"=w2137:string)  [unwired: 14 in]
      }
      frame "HW:ConfigAndAcquire02" {
        # "Your code here.\n(You can make a copy of, or modify, this frame)"
        n518 = call "Acquire Data from Hardware.vi"("Hardware Configuration"=T16 {"Physical Channel"="Dev3/ai0:31", "Maximum Input"=10.0, "Minimum Input"=-10.0, "Sample Rate"=1000.0, "Number of Samples"=100}) -> ("Graph Data"=w2144:waveform(dbl)[])  [unwired: 8 in, 1 out]
        n519 = call "ChSetting.vi"("dsc地址"="2", "AcquireData"=w2144) -> ("DevChSampData"=w2141:cluster{"通道编号":string, "Data":dbl}[], "DevChSampleData"=w2142:T28)  [unwired: 6 in, 2 out]
        n520 = Bundle By Name(cluster=w2140, "DevChSampleData"=w2142, "DevChSampData"=w2141) -> (w2139:T21)
        n521 = call <vilib>:"Add State(s) to Queue__JKI_lib_State_Machine.vi"("State(s) in (\"\")"=w2148) -> ("States Out"=w2147:string)  [unwired: 14 in]
      }
      frame "HW:ConfigAndAcquire03" {
        w2155 = T16 {"Physical Channel"="Dev4/ai0:31", "Maximum Input"=10.0, "Minimum Input"=-10.0, "Sample Rate"=1000.0, "Number of Samples"=100} ("Hardware Configuration")
        # "Your code here.\n(You can make a copy of, or modify, this frame)"
        n522 = To Variant(anything=w2155) -> (Variant=w2156:variant)
        n523 = call "Acquire Data from Hardware.vi"("Hardware Configuration"=w2155) -> ("Graph Data"=w2154:waveform(dbl)[])  [unwired: 8 in, 1 out]
        n524 = Variant To Data(type=w2155, Variant=w2156) -> ()  [unwired: 1 in, 2 out]
        n525 = call "ChSetting.vi"("dsc地址"="3", "AcquireData"=w2154) -> ("DevChSampData"=w2151:cluster{"通道编号":string, "Data":dbl}[], "DevChSampleData"=w2152:T28)  [unwired: 6 in, 2 out]
        n526 = Bundle By Name(cluster=w2150, "DevChSampleData"=w2152, "DevChSampData"=w2151) -> (w2149:T21)
        n527 = call <vilib>:"Add State(s) to Queue__JKI_lib_State_Machine.vi"("State(s) in (\"\")"=w2159) -> ("States Out"=w2158:string)  [unwired: 14 in]
      }
      frame "HW:ConfigAndAcquire04" {
        w2166 = T16 {"Physical Channel"="Dev5/ai0:31", "Maximum Input"=10.0, "Minimum Input"=-10.0, "Sample Rate"=1000.0, "Number of Samples"=100} ("Hardware Configuration")
        # "Your code here.\n(You can make a copy of, or modify, this frame)"
        n528 = To Variant(anything=w2166) -> (Variant=w2167:variant)
        n529 = call "Acquire Data from Hardware.vi"("Hardware Configuration"=w2166) -> ("Graph Data"=w2165:waveform(dbl)[])  [unwired: 8 in, 1 out]
        n530 = Variant To Data(type=w2166, Variant=w2167) -> ()  [unwired: 1 in, 2 out]
        n531 = call "ChSetting.vi"("dsc地址"="4", "AcquireData"=w2165) -> ("DevChSampData"=w2162:cluster{"通道编号":string, "Data":dbl}[], "DevChSampleData"=w2163:T28)  [unwired: 6 in, 2 out]
        n532 = Bundle By Name(cluster=w2161, "DevChSampleData"=w2163, "DevChSampData"=w2162) -> (w2160:T21)
        n533 = call <vilib>:"Add State(s) to Queue__JKI_lib_State_Machine.vi"("State(s) in (\"\")"=w2170) -> ("States Out"=w2169:string)  [unwired: 14 in]
      }
      frame "HW:ConfigAndAcquire05" {
        w2177 = T16 {"Physical Channel"="Dev6/ai0:31", "Maximum Input"=10.0, "Minimum Input"=-10.0, "Sample Rate"=1000.0, "Number of Samples"=100} ("Hardware Configuration")
        # "Your code here.\n(You can make a copy of, or modify, this frame)"
        n534 = To Variant(anything=w2177) -> (Variant=w2178:variant)
        n535 = call "Acquire Data from Hardware.vi"("Hardware Configuration"=w2177) -> ("Graph Data"=w2176:waveform(dbl)[])  [unwired: 8 in, 1 out]
        n536 = Variant To Data(type=w2177, Variant=w2178) -> ()  [unwired: 1 in, 2 out]
        n537 = call "ChSetting.vi"("dsc地址"="5", "AcquireData"=w2176) -> ("DevChSampData"=w2173:cluster{"通道编号":string, "Data":dbl}[], "DevChSampleData"=w2174:T28)  [unwired: 6 in, 2 out]
        n538 = Bundle By Name(cluster=w2172, "DevChSampleData"=w2174, "DevChSampData"=w2173) -> (w2171:T21)
        n539 = call <vilib>:"Add State(s) to Queue__JKI_lib_State_Machine.vi"("State(s) in (\"\")"=w2181) -> ("States Out"=w2180:string)  [unwired: 14 in]
      }
      frame "HW:ConfigAndAcquire06" {
        w2188 = T16 {"Physical Channel"="Dev7/ai0:31", "Maximum Input"=10.0, "Minimum Input"=-10.0, "Sample Rate"=1000.0, "Number of Samples"=100} ("Hardware Configuration")
        # "Your code here.\n(You can make a copy of, or modify, this frame)"
        n540 = To Variant(anything=w2188) -> (Variant=w2189:variant)
        n541 = call "Acquire Data from Hardware.vi"("Hardware Configuration"=w2188) -> ("Graph Data"=w2187:waveform(dbl)[])  [unwired: 8 in, 1 out]
        n542 = Variant To Data(type=w2188, Variant=w2189) -> ()  [unwired: 1 in, 2 out]
        n543 = call "ChSetting.vi"("dsc地址"="6", "AcquireData"=w2187) -> ("DevChSampData"=w2184:cluster{"通道编号":string, "Data":dbl}[], "DevChSampleData"=w2185:T28)  [unwired: 6 in, 2 out]
        n544 = Bundle By Name(cluster=w2183, "DevChSampleData"=w2185, "DevChSampData"=w2184) -> (w2182:T21)
        n545 = call <vilib>:"Add State(s) to Queue__JKI_lib_State_Machine.vi"("State(s) in (\"\")"=w2192) -> ("States Out"=w2191:string)  [unwired: 14 in]
      }
      frame "HW:ConfigAndAcquire07" {
        w2199 = T16 {"Physical Channel"="Dev8/ai0:31", "Maximum Input"=10.0, "Minimum Input"=-10.0, "Sample Rate"=1000.0, "Number of Samples"=100} ("Hardware Configuration")
        # "Your code here.\n(You can make a copy of, or modify, this frame)"
        n546 = To Variant(anything=w2199) -> (Variant=w2200:variant)
        n547 = call "Acquire Data from Hardware.vi"("Hardware Configuration"=w2199) -> ("Graph Data"=w2198:waveform(dbl)[])  [unwired: 8 in, 1 out]
        n548 = Variant To Data(type=w2199, Variant=w2200) -> ()  [unwired: 1 in, 2 out]
        n549 = call "ChSetting.vi"("dsc地址"="7", "AcquireData"=w2198) -> ("DevChSampData"=w2195:cluster{"通道编号":string, "Data":dbl}[], "DevChSampleData"=w2196:T28)  [unwired: 6 in, 2 out]
        n550 = Bundle By Name(cluster=w2194, "DevChSampleData"=w2196, "DevChSampData"=w2195) -> (w2193:T21)
        n551 = call <vilib>:"Add State(s) to Queue__JKI_lib_State_Machine.vi"("State(s) in (\"\")"=w2203) -> ("States Out"=w2202:string)  [unwired: 14 in]
      }
      frame "HW:ConfigAndAcquire08" {
        w2210 = T16 {"Physical Channel"="Dev11/ai0:31", "Maximum Input"=10.0, "Minimum Input"=-10.0, "Sample Rate"=1000.0, "Number of Samples"=100} ("Hardware Configuration")
        # "Your code here.\n(You can make a copy of, or modify, this frame)"
        n552 = To Variant(anything=w2210) -> (Variant=w2211:variant)
        n553 = call "Acquire Data from Hardware.vi"("Hardware Configuration"=w2210) -> ("Graph Data"=w2209:waveform(dbl)[])  [unwired: 8 in, 1 out]
        n554 = Variant To Data(type=w2210, Variant=w2211) -> ()  [unwired: 1 in, 2 out]
        n555 = call "ChSetting.vi"("dsc地址"="8", "AcquireData"=w2209) -> ("DevChSampData"=w2206:cluster{"通道编号":string, "Data":dbl}[], "DevChSampleData"=w2207:T28)  [unwired: 6 in, 2 out]
        n556 = Bundle By Name(cluster=w2205, "DevChSampleData"=w2207, "DevChSampData"=w2206) -> (w2204:T21)
        n557 = call <vilib>:"Add State(s) to Queue__JKI_lib_State_Machine.vi"("State(s) in (\"\")"=w2214) -> ("States Out"=w2213:string)  [unwired: 14 in]
      }
      frame "HW:ConfigAndAcquire09" {
        w2221 = T16 {"Physical Channel"="Dev12/ai0:31", "Maximum Input"=10.0, "Minimum Input"=-10.0, "Sample Rate"=1000.0, "Number of Samples"=100} ("Hardware Configuration")
        # "Your code here.\n(You can make a copy of, or modify, this frame)"
        n558 = To Variant(anything=w2221) -> (Variant=w2222:variant)
        n559 = call "Acquire Data from Hardware.vi"("Hardware Configuration"=w2221) -> ("Graph Data"=w2220:waveform(dbl)[])  [unwired: 8 in, 1 out]
        n560 = Variant To Data(type=w2221, Variant=w2222) -> ()  [unwired: 1 in, 2 out]
        n561 = call "ChSetting.vi"("dsc地址"="9", "AcquireData"=w2220) -> ("DevChSampData"=w2217:cluster{"通道编号":string, "Data":dbl}[], "DevChSampleData"=w2218:T28)  [unwired: 6 in, 2 out]
        n562 = Bundle By Name(cluster=w2216, "DevChSampleData"=w2218, "DevChSampData"=w2217) -> (w2215:T21)
        n563 = call <vilib>:"Add State(s) to Queue__JKI_lib_State_Machine.vi"("State(s) in (\"\")"=w2225) -> ("States Out"=w2224:string)  [unwired: 14 in]
      }
      frame "HW:ConfigAndAcquire10" {
        w2232 = T16 {"Physical Channel"="Dev13/ai0:31", "Maximum Input"=10.0, "Minimum Input"=-10.0, "Sample Rate"=1000.0, "Number of Samples"=100} ("Hardware Configuration")
        # "Your code here.\n(You can make a copy of, or modify, this frame)"
        n564 = To Variant(anything=w2232) -> (Variant=w2233:variant)
        n565 = call "Acquire Data from Hardware.vi"("Hardware Configuration"=w2232) -> ("Graph Data"=w2231:waveform(dbl)[])  [unwired: 8 in, 1 out]
        n566 = Variant To Data(type=w2232, Variant=w2233) -> ()  [unwired: 1 in, 2 out]
        n567 = call "ChSetting.vi"("dsc地址"="10", "AcquireData"=w2231) -> ("DevChSampData"=w2228:cluster{"通道编号":string, "Data":dbl}[], "DevChSampleData"=w2229:T28)  [unwired: 6 in, 2 out]
        n568 = Bundle By Name(cluster=w2227, "DevChSampleData"=w2229, "DevChSampData"=w2228) -> (w2226:T21)
        n569 = call <vilib>:"Add State(s) to Queue__JKI_lib_State_Machine.vi"("State(s) in (\"\")"=w2236) -> ("States Out"=w2235:string)  [unwired: 14 in]
      }
      frame "HW:ConfigAndAcquire11" {
        w2243 = T16 {"Physical Channel"="Dev14/ai0:31", "Maximum Input"=10.0, "Minimum Input"=-10.0, "Sample Rate"=1000.0, "Number of Samples"=100} ("Hardware Configuration")
        # "Your code here.\n(You can make a copy of, or modify, this frame)"
        n570 = To Variant(anything=w2243) -> (Variant=w2244:variant)
        n571 = call "Acquire Data from Hardware.vi"("Hardware Configuration"=w2243) -> ("Graph Data"=w2242:waveform(dbl)[])  [unwired: 8 in, 1 out]
        n572 = Variant To Data(type=w2243, Variant=w2244) -> ()  [unwired: 1 in, 2 out]
        n573 = call "ChSetting.vi"("dsc地址"="11", "AcquireData"=w2242) -> ("DevChSampData"=w2239:cluster{"通道编号":string, "Data":dbl}[], "DevChSampleData"=w2240:T28)  [unwired: 6 in, 2 out]
        n574 = Bundle By Name(cluster=w2238, "DevChSampleData"=w2240, "DevChSampData"=w2239) -> (w2237:T21)
        n575 = call <vilib>:"Add State(s) to Queue__JKI_lib_State_Machine.vi"("State(s) in (\"\")"=w2247) -> ("States Out"=w2246:string)  [unwired: 14 in]
      }
      frame "HW:ConfigAndAcquire12" {
        w2254 = T16 {"Physical Channel"="Dev15/ai0:31", "Maximum Input"=10.0, "Minimum Input"=-10.0, "Sample Rate"=1000.0, "Number of Samples"=100} ("Hardware Configuration")
        # "Your code here.\n(You can make a copy of, or modify, this frame)"
        n576 = To Variant(anything=w2254) -> (Variant=w2255:variant)
        n577 = call "Acquire Data from Hardware.vi"("Hardware Configuration"=w2254) -> ("Graph Data"=w2253:waveform(dbl)[])  [unwired: 8 in, 1 out]
        n578 = Variant To Data(type=w2254, Variant=w2255) -> ()  [unwired: 1 in, 2 out]
        n579 = call "ChSetting.vi"("dsc地址"="12", "AcquireData"=w2253) -> ("DevChSampData"=w2250:cluster{"通道编号":string, "Data":dbl}[], "DevChSampleData"=w2251:T28)  [unwired: 6 in, 2 out]
        n580 = Bundle By Name(cluster=w2249, "DevChSampleData"=w2251, "DevChSampData"=w2250) -> (w2248:T21)
        n581 = call <vilib>:"Add State(s) to Queue__JKI_lib_State_Machine.vi"("State(s) in (\"\")"=w2258) -> ("States Out"=w2257:string)  [unwired: 14 in]
      }
      frame "HW:ConfigAndAcquire13" {
        w2265 = T16 {"Physical Channel"="Dev16/ai0:31", "Maximum Input"=10.0, "Minimum Input"=-10.0, "Sample Rate"=1000.0, "Number of Samples"=100} ("Hardware Configuration")
        # "Your code here.\n(You can make a copy of, or modify, this frame)"
        n582 = To Variant(anything=w2265) -> (Variant=w2266:variant)
        n583 = call "Acquire Data from Hardware.vi"("Hardware Configuration"=w2265) -> ("Graph Data"=w2264:waveform(dbl)[])  [unwired: 8 in, 1 out]
        n584 = Variant To Data(type=w2265, Variant=w2266) -> ()  [unwired: 1 in, 2 out]
        n585 = call "ChSetting.vi"("dsc地址"="13", "AcquireData"=w2264) -> ("DevChSampData"=w2261:cluster{"通道编号":string, "Data":dbl}[], "DevChSampleData"=w2262:T28)  [unwired: 6 in, 2 out]
        n586 = Bundle By Name(cluster=w2260, "DevChSampleData"=w2262, "DevChSampData"=w2261) -> (w2259:T21)
        n587 = call <vilib>:"Add State(s) to Queue__JKI_lib_State_Machine.vi"("State(s) in (\"\")"=w2269) -> ("States Out"=w2268:string)  [unwired: 14 in]
      }
      frame "HW:Configure" {
        # "Your code here.\n(You can make a copy of, or modify, this frame)"
        n588 = Unbundle By Name(w2271) -> ("User Specified"=w2275:T18)
        n589 = call "Settings Dialog.vi"("error in (no error)"=w2274, "Configuration in"=w2275) -> ("error out"=w2273:errorcluster, "Configuration out"=w2272:T18)  [unwired: 7 in, 1 out]
        n590 = Bundle By Name(cluster=w2271, "User Specified"=w2272) -> (w2270:T21)
        n591 = call <vilib>:"Add State(s) to Queue__JKI_lib_State_Machine.vi"("State(s) in (\"\")"=w2277) -> ("States Out"=w2276:string)  [unwired: 14 in]
      }
    }
  }
  n592 = Destroy User Event(user event=w14, error in=w12) -> (error out=w17:errorcluster)
  n593 = Unregister For Events(event registration refnum=w15, error in=w17) -> (error out=w16:errorcluster)
  n594 = call <vilib>:"Simple Error Handler.vi"("error in (no error)"=w16) -> ()  [unwired: 4 in, 5 out]
